vi "S2C_FPGA_SimulatedData.vi"(0 "sim I/O info in":T1, 9 "data from node input terminals":variant[](array[variant]), 11 "input from node terminal error in":errorcluster) -> (4 "sim I/O info out":T1, 10 "data to node output terminals":variant[](array[variant]), 15 "output to node terminal error out":errorcluster)   [LabVIEW 2015]
uses:
  <vilib>/FPGA/viExecutionOnDevComputer/simIO/customVI/Sim IO Info.ctl
  <vilib>/rvi/customViForEmulation/niLvFPGAUserSpecifiedEmulationVISupport.lvclass
  S2C_FPGA_InterfaceGlobals.vi
  <vilib>/FPGA/viExecutionOnDevComputer/simIO/customVI/niFPGA Simulated IO.lvlib
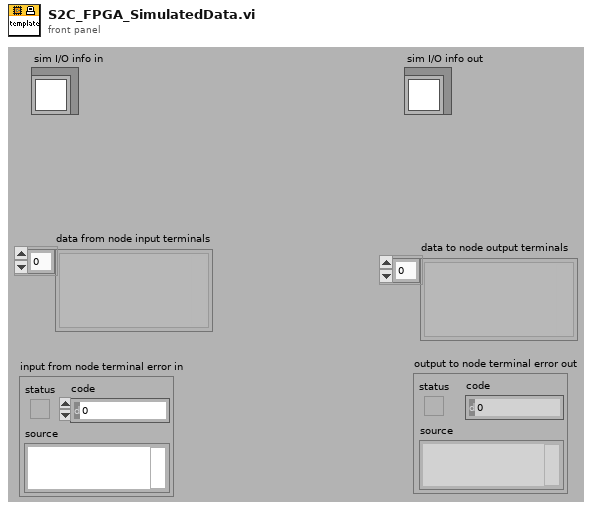
[diagram p1: front panel]
types:
  T1 = typedef "niFPGA Simulated IO.lvlib/Sim IO Info.ctl" = refnum<class "niLvFPGAUserSpecifiedEmulationVISupport.lvclass">
  T2 = typedef "niFPGA Simulated IO.lvlib/Execution Stage.ctl" = enum16{"Initializing", "Running", "Shutting Down"}
  T3 = typedef "niFPGA Simulated IO.lvlib/Node or Element Type.ctl" = enum16{"Read I/O", "Write I/O", "Method", "Read Property", "Write Property"}
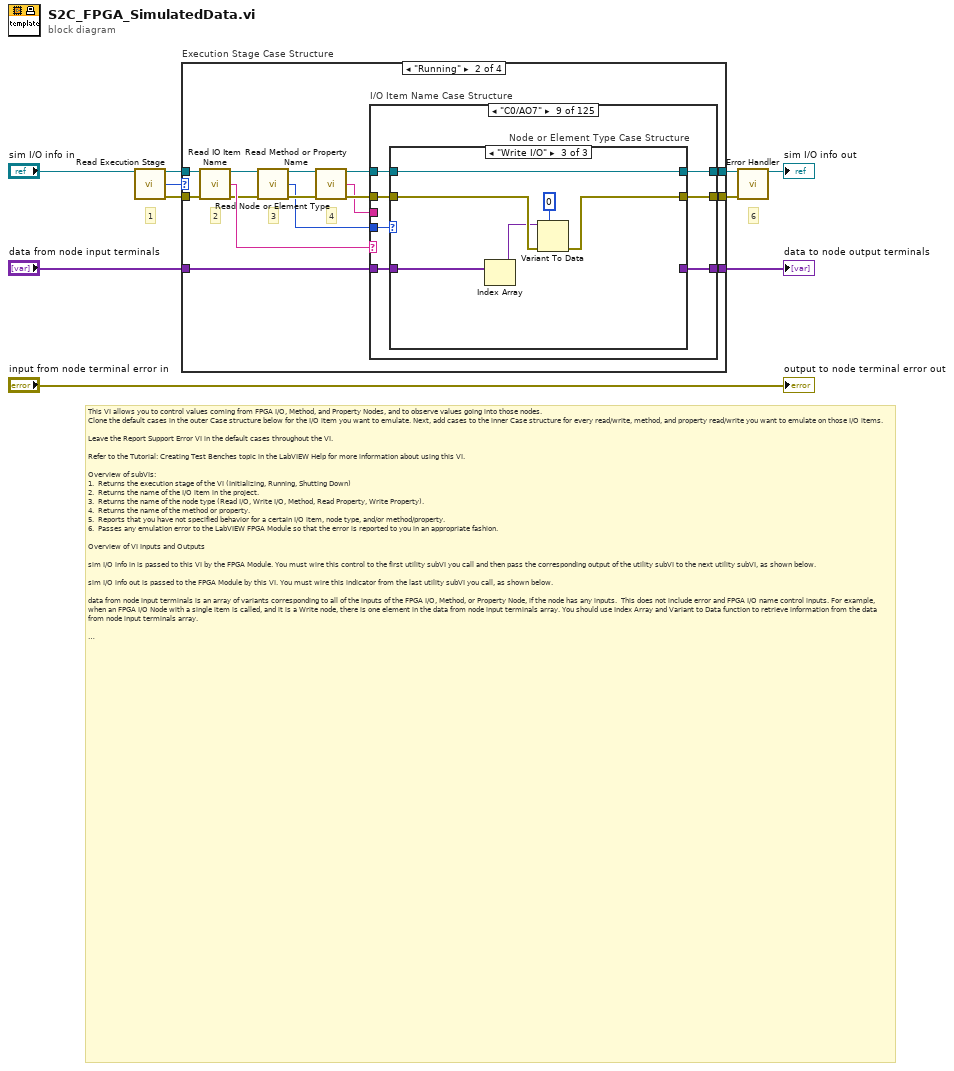
[diagram p0: block diagram]
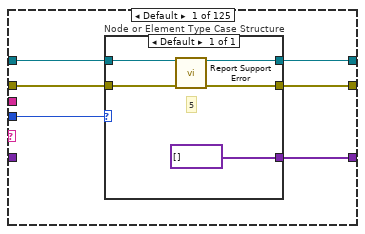
[diagram p3: hidden frame]
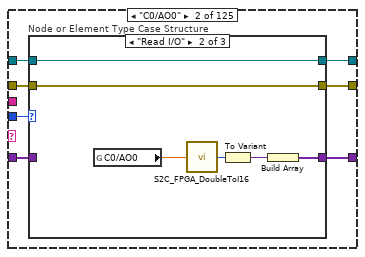
[diagram p4: hidden frame]
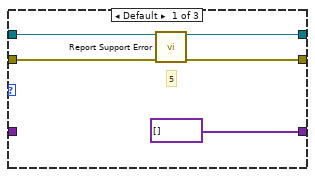
[diagram p5: hidden frame]
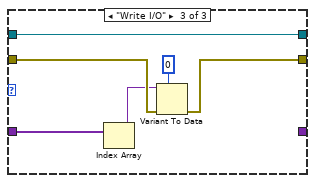
[diagram p6: hidden frame]
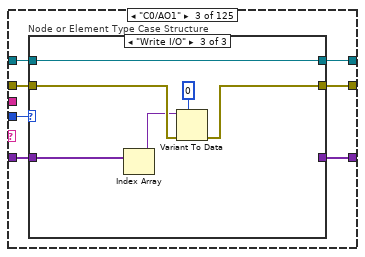
[diagram p7: hidden frame]
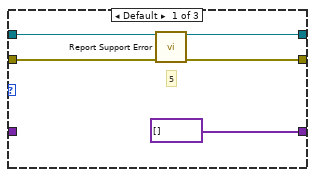
[diagram p8: hidden frame]
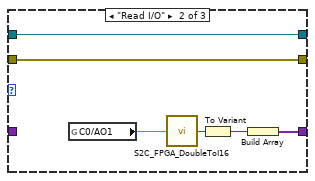
[diagram p9: hidden frame]
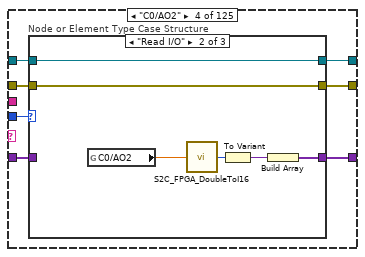
[diagram p10: hidden frame]
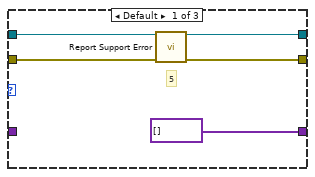
[diagram p11: hidden frame]
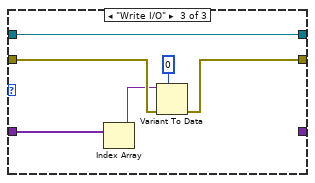
[diagram p12: hidden frame]
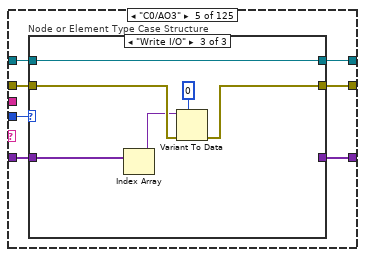
[diagram p13: hidden frame]
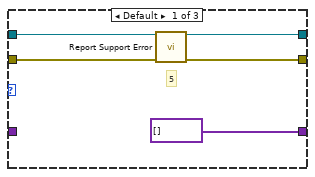
[diagram p14: hidden frame]
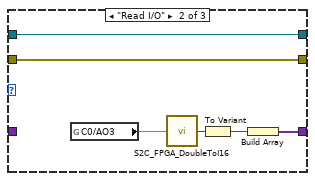
[diagram p15: hidden frame]
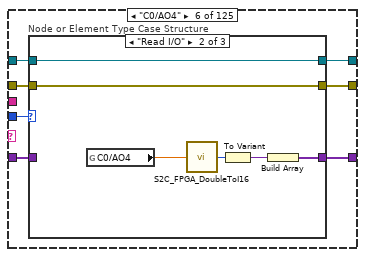
[diagram p16: hidden frame]
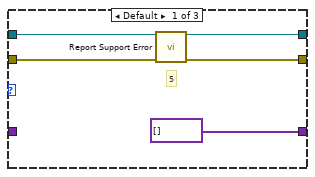
[diagram p17: hidden frame]
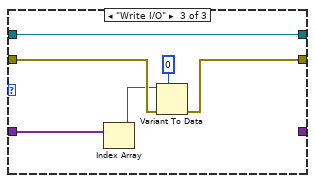
[diagram p18: hidden frame]
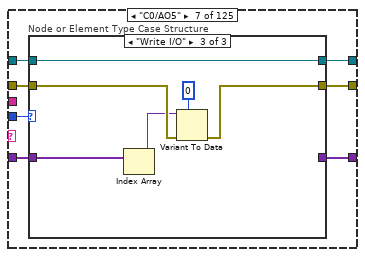
[diagram p19: hidden frame]
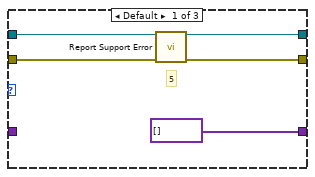
[diagram p20: hidden frame]
diagram:
  # "1"
  # "6"
  # "This VI allows you to control values coming from FPGA I/O, Method, and Property Nodes, and to observe values going into those nodes.\nClone the default cases in the outer Case structure below for the I/O item you want to emulate. Next, add cases to the inner Case structure for every read/write, method, and property read/write you want to emulate on those I/O items.  \n\nLeave the Report Support Error VI in the default cases throughout the VI.\n\nRefer to the Tutorial: Creating Test Benches topic in the LabVIEW Help for more information about using this VI.\n\nOverview of subVIs:\n1.  Returns the execution stage of the VI (Initializing, Running, Shutting Down)\n2.  Returns the name of the I/O item in the project.\n3.  Returns the name of the node type (Read I/O, Write I/O, Method, Read Property, Write Property).\n4.  Returns the name of the method or property.\n5.  Reports that you have not specified behavior for a certain I/O item, node type, and/or method/property.\n6.  Passes any emulation error to the LabVIEW FPGA Module so that the error is reported to you in an appropriate fashion.\n\nOverview of VI Inputs and Outputs\n\nsim I/O info in is passed to this VI by the FPGA Module. You must wire this control to the first utility subVI you call and then pass the corresponding output of the utility subVI to the next utility subVI, as shown below.\n\nsim I/O info out is passed to the FPGA Module by this VI. You must wire this indicator from the last utility subVI you call, as shown below.\n\ndata from node input terminals is an array of variants corresponding to all of the inputs of the FPGA I/O, Method, or Property Node, if the node has any inputs.  This does not include error and FPGA I/O name control inputs. For example, when an FPGA I/O Node with a single item is called, and it is a Write node, there is one element in the data from node input terminals array. You should use Index Array and Variant to Data function to retrieve information from the data from node input terminals array.\n\ndata to node output terminals is an array of variants corresponding to all the outputs of the FPGA I/O, Method, or Property Node, if the node has any outputs.  This does not include error and FPGA I/O name control outputs. For example, when an FPGA I/O node with a single item is called, and it is a Read node, there should be one element in the data to node output terminals array. You should use To Variant and Build Array functions to pass the information to the data to node output terminals array.\n\ninput from node terminal error in is the error that gets passed into the FPGA I/O, Method, or Property Node, if the node is configured so that the error input is shown. If the node is configured so that the error input is not shown, the value of this input corresponds to \"no error\" (status is false, error code is 0). \n\noutput to node terminal error out is the error that gets passed out of the FPGA I/O, Method, or Property Node, if the node is configured so that the error output is shown.  If the node is configured so that the error output is not shown, the value of this output is ignored."
  n1 = call <vilib>:"Read Execution Stage.vi"("sim I/O info in"="sim I/O info in") -> ("sim I/O info out"=w3:T1, "execution stage"=w1:T2, "error out"=w2:errorcluster)  [unwired: 1 in, 11 out]
  n2 = case "Execution Stage Case Structure" shown="\"Running\"" w1 {
    tunnel: [_ w26 _ _] -> w9
    tunnel: [w12 w21 w3124 w3126] -> w4
    tunnel: [w11 w17 w3123 w3125] -> w6
    tunnel: w3 -> [w11 w15 w3123 w3125]
    tunnel: w2 -> [w12 w14 w3124 w3126]
    tunnel: "data from node input terminals" -> [_ w27 _ _]
    frame "Initializing" {
    }
    frame "Running" {
      # "4"
      # "3"
      # "2"
      n3 = call <vilib>:"Read IO Item Name.vi"("sim I/O info in"=w15, "error in (no error)"=w14) -> ("sim I/O info out"=w16:T1, "I/O item name"=w25:string, "error out"=w24:errorcluster)  [unwired: 11 out]
      n4 = call <vilib>:"Read Node or Element Type.vi"("sim I/O info in"=w16, "error in (no error)"=w24) -> ("sim I/O info out"=w13:T1, "node or element type"=w22:T3, "error out"=w23:errorcluster)  [unwired: 11 out]
      n5 = call <vilib>:"Read Method or Property Name.vi"("sim I/O info in"=w13, "error in (no error)"=w23) -> ("sim I/O info out"=w19:T1, "method or property name"=w18:string, "error out"=w20:errorcluster)  [unwired: 11 out]
      n6 = case "I/O Item Name Case Structure" shown="\"C0/AO7\"" w25 {
        tunnel: w27 -> [_ w39 w63 w87 w111 w135 w159 w183 w207 w231 w255 w279 w303 w327 w351 w375 w399 w423 w456 w489 w522 w555 w588 w621 w654 w687 w720 w753 w786 w819 w843 w867 w891 w915 w939 w963 w987 w1011 w1035 w1059 w1083 w1107 w1131 w1155 w1179 w1203 w1227 w1251 w1275 w1299 w1323 w1347 w1371 w1395 w1419 w1443 w1467 w1491 w1515 w1539 w1563 w1587 w1611 w1635 w1659 w1683 w1707 w1731 w1755 w1779 w1803 w1827 w1851 w1875 w1899 w1923 w1947 w1971 w1995 w2019 w2043 w2067 w2091 w2115 w2139 w2163 w2187 w2211 w2235 w2259 w2283 w2307 w2331 w2355 w2379 w2403 w2427 w2451 w2475 w2499 w2523 w2547 w2571 w2595 w2619 w2643 w2667 w2691 w2715 w2739 w2763 w2787 w2811 w2835 w2859 w2883 w2907 w2931 w2955 w2979 w3003 w3027 w3051 w3075 w3099]
        tunnel: [w29 w41 w65 w89 w113 w137 w161 w185 w209 w233 w257 w281 w305 w329 w353 w377 w401 w425 w458 w491 w524 w557 w590 w623 w656 w689 w722 w755 w788 w821 w845 w869 w893 w917 w941 w965 w989 w1013 w1037 w1061 w1085 w1109 w1133 w1157 w1181 w1205 w1229 w1253 w1277 w1301 w1325 w1349 w1373 w1397 w1421 w1445 w1469 w1493 w1517 w1541 w1565 w1589 w1613 w1637 w1661 w1685 w1709 w1733 w1757 w1781 w1805 w1829 w1853 w1877 w1901 w1925 w1949 w1973 w1997 w2021 w2045 w2069 w2093 w2117 w2141 w2165 w2189 w2213 w2237 w2261 w2285 w2309 w2333 w2357 w2381 w2405 w2429 w2453 w2477 w2501 w2525 w2549 w2573 w2597 w2621 w2645 w2669 w2693 w2717 w2741 w2765 w2789 w2813 w2837 w2861 w2885 w2909 w2933 w2957 w2981 w3005 w3029 w3053 w3077 w3101] -> w26
        tunnel: w20 -> [w33 w45 w69 w93 w117 w141 w165 w189 w213 w237 w261 w285 w309 w333 w357 w381 w405 w429 w462 w495 w528 w561 w594 w627 w660 w693 w726 w759 w792 w825 w849 w873 w897 w921 w945 w969 w993 w1017 w1041 w1065 w1089 w1113 w1137 w1161 w1185 w1209 w1233 w1257 w1281 w1305 w1329 w1353 w1377 w1401 w1425 w1449 w1473 w1497 w1521 w1545 w1569 w1593 w1617 w1641 w1665 w1689 w1713 w1737 w1761 w1785 w1809 w1833 w1857 w1881 w1905 w1929 w1953 w1977 w2001 w2025 w2049 w2073 w2097 w2121 w2145 w2169 w2193 w2217 w2241 w2265 w2289 w2313 w2337 w2361 w2385 w2409 w2433 w2457 w2481 w2505 w2529 w2553 w2577 w2601 w2625 w2649 w2673 w2697 w2721 w2745 w2769 w2793 w2817 w2841 w2865 w2889 w2913 w2937 w2961 w2985 w3009 w3033 w3057 w3081 w3105]
        tunnel: [w32 w44 w68 w92 w116 w140 w164 w188 w212 w236 w260 w284 w308 w332 w356 w380 w404 w428 w461 w494 w527 w560 w593 w626 w659 w692 w725 w758 w791 w824 w848 w872 w896 w920 w944 w968 w992 w1016 w1040 w1064 w1088 w1112 w1136 w1160 w1184 w1208 w1232 w1256 w1280 w1304 w1328 w1352 w1376 w1400 w1424 w1448 w1472 w1496 w1520 w1544 w1568 w1592 w1616 w1640 w1664 w1688 w1712 w1736 w1760 w1784 w1808 w1832 w1856 w1880 w1904 w1928 w1952 w1976 w2000 w2024 w2048 w2072 w2096 w2120 w2144 w2168 w2192 w2216 w2240 w2264 w2288 w2312 w2336 w2360 w2384 w2408 w2432 w2456 w2480 w2504 w2528 w2552 w2576 w2600 w2624 w2648 w2672 w2696 w2720 w2744 w2768 w2792 w2816 w2840 w2864 w2888 w2912 w2936 w2960 w2984 w3008 w3032 w3056 w3080 w3104] -> w21
        tunnel: w19 -> [w31 w43 w67 w91 w115 w139 w163 w187 w211 w235 w259 w283 w307 w331 w355 w379 w403 w427 w460 w493 w526 w559 w592 w625 w658 w691 w724 w757 w790 w823 w847 w871 w895 w919 w943 w967 w991 w1015 w1039 w1063 w1087 w1111 w1135 w1159 w1183 w1207 w1231 w1255 w1279 w1303 w1327 w1351 w1375 w1399 w1423 w1447 w1471 w1495 w1519 w1543 w1567 w1591 w1615 w1639 w1663 w1687 w1711 w1735 w1759 w1783 w1807 w1831 w1855 w1879 w1903 w1927 w1951 w1975 w1999 w2023 w2047 w2071 w2095 w2119 w2143 w2167 w2191 w2215 w2239 w2263 w2287 w2311 w2335 w2359 w2383 w2407 w2431 w2455 w2479 w2503 w2527 w2551 w2575 w2599 w2623 w2647 w2671 w2695 w2719 w2743 w2767 w2791 w2815 w2839 w2863 w2887 w2911 w2935 w2959 w2983 w3007 w3031 w3055 w3079 w3103]
        tunnel: [w30 w42 w66 w90 w114 w138 w162 w186 w210 w234 w258 w282 w306 w330 w354 w378 w402 w426 w459 w492 w525 w558 w591 w624 w657 w690 w723 w756 w789 w822 w846 w870 w894 w918 w942 w966 w990 w1014 w1038 w1062 w1086 w1110 w1134 w1158 w1182 w1206 w1230 w1254 w1278 w1302 w1326 w1350 w1374 w1398 w1422 w1446 w1470 w1494 w1518 w1542 w1566 w1590 w1614 w1638 w1662 w1686 w1710 w1734 w1758 w1782 w1806 w1830 w1854 w1878 w1902 w1926 w1950 w1974 w1998 w2022 w2046 w2070 w2094 w2118 w2142 w2166 w2190 w2214 w2238 w2262 w2286 w2310 w2334 w2358 w2382 w2406 w2430 w2454 w2478 w2502 w2526 w2550 w2574 w2598 w2622 w2646 w2670 w2694 w2718 w2742 w2766 w2790 w2814 w2838 w2862 w2886 w2910 w2934 w2958 w2982 w3006 w3030 w3054 w3078 w3102] -> w17
        tunnel: w22 -> [w28 w40 w64 w88 w112 w136 w160 w184 w208 w232 w256 w280 w304 w328 w352 w376 w400 w424 w457 w490 w523 w556 w589 w622 w655 w688 w721 w754 w787 w820 w844 w868 w892 w916 w940 w964 w988 w1012 w1036 w1060 w1084 w1108 w1132 w1156 w1180 w1204 w1228 w1252 w1276 w1300 w1324 w1348 w1372 w1396 w1420 w1444 w1468 w1492 w1516 w1540 w1564 w1588 w1612 w1636 w1660 w1684 w1708 w1732 w1756 w1780 w1804 w1828 w1852 w1876 w1900 w1924 w1948 w1972 w1996 w2020 w2044 w2068 w2092 w2116 w2140 w2164 w2188 w2212 w2236 w2260 w2284 w2308 w2332 w2356 w2380 w2404 w2428 w2452 w2476 w2500 w2524 w2548 w2572 w2596 w2620 w2644 w2668 w2692 w2716 w2740 w2764 w2788 w2812 w2836 w2860 w2884 w2908 w2932 w2956 w2980 w3004 w3028 w3052 w3076 w3100]
        tunnel: w18 -> [_ _ _ _ _ _ _ _ _ _ _ _ _ _ _ _ _ _ _ _ _ _ _ _ _ _ _ _ _ _ _ _ _ _ _ _ _ _ _ _ _ _ _ _ _ _ _ _ _ _ _ _ _ _ _ _ _ _ _ _ _ _ _ _ _ _ _ _ _ _ _ _ _ _ _ _ _ _ _ _ _ _ _ _ _ _ _ _ _ _ _ _ _ _ _ _ _ _ _ _ _ _ _ _ _ _ _ _ _ _ _ _ _ _ _ _ _ _ _ _ _ _ _ _ _]
        frame Default {
          n7 = case "Node or Element Type Case Structure" shown="Default" w28 {
            tunnel: w33 -> [w38]
            tunnel: [w37] -> w32
            tunnel: w31 -> [w36]
            tunnel: [w35] -> w30
            tunnel: [variant[] []] -> w29
            frame Default {
              # "5"
              n8 = call <vilib>:"Report Support Error.vi"("sim I/O info in"=w36, "error in (no error)"=w38) -> ("sim I/O info out"=w35:T1, "error out"=w37:errorcluster)  [unwired: 12 out]
            }
          }
        }
        frame "C0/AO0" {
          n9 = case "Node or Element Type Case Structure" shown="\"Read I/O\"" w40 {
            tunnel: w45 -> [w50 w56 w60]
            tunnel: [w49 w56 w59] -> w44
            tunnel: w43 -> [w48 w55 w62]
            tunnel: [w47 w55 w62] -> w42
            tunnel: [variant[] [] w54 _] -> w41
            tunnel: w39 -> [_ _ w61]
            frame Default {
              # "5"
              n10 = call <vilib>:"Report Support Error.vi"("sim I/O info in"=w48, "error in (no error)"=w50) -> ("sim I/O info out"=w47:T1, "error out"=w49:errorcluster)  [unwired: 12 out]
            }
            frame "Read I/O" {
              n11 = global read "S2C_FPGA_InterfaceGlobals.vi" "C0/AO0"() -> (w52:dbl)
              n12 = call "S2C_FPGA_DoubleToI16.vi"("Double In"=w52) -> ("I16 Out"=w51:i16)  [unwired: 4 in]
              n13 = To Variant(anything=w51) -> (Variant=w53:variant)
              n14 = Build Array(w53) -> (w54:variant[])
            }
            frame "Write I/O" {
              n15 = Index Array(array=w61) -> (element=w58:variant)  [unwired: 1 in]
              n16 = Variant To Data(error in=w60, type=i16 0 ("C0/AI0"), Variant=w58) -> (error out=w59:errorcluster)  [unwired: 1 out]
            }
          }
        }
        frame "C0/AO1" {
          n17 = case "Node or Element Type Case Structure" shown="\"Write I/O\"" w64 {
            tunnel: w69 -> [w74 w80 w84]
            tunnel: [w73 w80 w83] -> w68
            tunnel: w67 -> [w72 w79 w86]
            tunnel: [w71 w79 w86] -> w66
            tunnel: [variant[] [] w77 _] -> w65
            tunnel: w63 -> [_ _ w85]
            frame Default {
              # "5"
              n18 = call <vilib>:"Report Support Error.vi"("sim I/O info in"=w72, "error in (no error)"=w74) -> ("sim I/O info out"=w71:T1, "error out"=w73:errorcluster)  [unwired: 12 out]
            }
            frame "Read I/O" {
              n19 = global read "S2C_FPGA_InterfaceGlobals.vi" "C0/AO1"() -> (w75:dbl)
              n20 = call "S2C_FPGA_DoubleToI16.vi"("Double In"=w75) -> ("I16 Out"=w76:i16)  [unwired: 4 in]
              n21 = To Variant(anything=w76) -> (Variant=w78:variant)
              n22 = Build Array(w78) -> (w77:variant[])
            }
            frame "Write I/O" {
              n23 = Index Array(array=w85) -> (element=w82:variant)  [unwired: 1 in]
              n24 = Variant To Data(error in=w84, type=i16 0 ("C0/AI0"), Variant=w82) -> (error out=w83:errorcluster)  [unwired: 1 out]
            }
          }
        }
        frame "C0/AO2" {
          n25 = case "Node or Element Type Case Structure" shown="\"Read I/O\"" w88 {
            tunnel: w93 -> [w98 w104 w108]
            tunnel: [w97 w104 w107] -> w92
            tunnel: w91 -> [w96 w103 w110]
            tunnel: [w95 w103 w110] -> w90
            tunnel: [variant[] [] w101 _] -> w89
            tunnel: w87 -> [_ _ w109]
            frame Default {
              # "5"
              n26 = call <vilib>:"Report Support Error.vi"("sim I/O info in"=w96, "error in (no error)"=w98) -> ("sim I/O info out"=w95:T1, "error out"=w97:errorcluster)  [unwired: 12 out]
            }
            frame "Read I/O" {
              n27 = global read "S2C_FPGA_InterfaceGlobals.vi" "C0/AO2"() -> (w99:dbl)
              n28 = call "S2C_FPGA_DoubleToI16.vi"("Double In"=w99) -> ("I16 Out"=w100:i16)  [unwired: 4 in]
              n29 = To Variant(anything=w100) -> (Variant=w102:variant)
              n30 = Build Array(w102) -> (w101:variant[])
            }
            frame "Write I/O" {
              n31 = Index Array(array=w109) -> (element=w106:variant)  [unwired: 1 in]
              n32 = Variant To Data(error in=w108, type=i16 0 ("C0/AI0"), Variant=w106) -> (error out=w107:errorcluster)  [unwired: 1 out]
            }
          }
        }
        frame "C0/AO3" {
          n33 = case "Node or Element Type Case Structure" shown="\"Write I/O\"" w112 {
            tunnel: w117 -> [w122 w128 w132]
            tunnel: [w121 w128 w131] -> w116
            tunnel: w115 -> [w120 w127 w134]
            tunnel: [w119 w127 w134] -> w114
            tunnel: [variant[] [] w125 _] -> w113
            tunnel: w111 -> [_ _ w133]
            frame Default {
              # "5"
              n34 = call <vilib>:"Report Support Error.vi"("sim I/O info in"=w120, "error in (no error)"=w122) -> ("sim I/O info out"=w119:T1, "error out"=w121:errorcluster)  [unwired: 12 out]
            }
            frame "Read I/O" {
              n35 = global read "S2C_FPGA_InterfaceGlobals.vi" "C0/AO3"() -> (w123:dbl)
              n36 = call "S2C_FPGA_DoubleToI16.vi"("Double In"=w123) -> ("I16 Out"=w124:i16)  [unwired: 4 in]
              n37 = To Variant(anything=w124) -> (Variant=w126:variant)
              n38 = Build Array(w126) -> (w125:variant[])
            }
            frame "Write I/O" {
              n39 = Index Array(array=w133) -> (element=w130:variant)  [unwired: 1 in]
              n40 = Variant To Data(error in=w132, type=i16 0 ("C0/AI0"), Variant=w130) -> (error out=w131:errorcluster)  [unwired: 1 out]
            }
          }
        }
        frame "C0/AO4" {
          n41 = case "Node or Element Type Case Structure" shown="\"Read I/O\"" w136 {
            tunnel: w141 -> [w146 w152 w156]
            tunnel: [w145 w152 w155] -> w140
            tunnel: w139 -> [w144 w151 w158]
            tunnel: [w143 w151 w158] -> w138
            tunnel: [variant[] [] w149 _] -> w137
            tunnel: w135 -> [_ _ w157]
            frame Default {
              # "5"
              n42 = call <vilib>:"Report Support Error.vi"("sim I/O info in"=w144, "error in (no error)"=w146) -> ("sim I/O info out"=w143:T1, "error out"=w145:errorcluster)  [unwired: 12 out]
            }
            frame "Read I/O" {
              n43 = global read "S2C_FPGA_InterfaceGlobals.vi" "C0/AO4"() -> (w147:dbl)
              n44 = call "S2C_FPGA_DoubleToI16.vi"("Double In"=w147) -> ("I16 Out"=w148:i16)  [unwired: 4 in]
              n45 = To Variant(anything=w148) -> (Variant=w150:variant)
              n46 = Build Array(w150) -> (w149:variant[])
            }
            frame "Write I/O" {
              n47 = Index Array(array=w157) -> (element=w154:variant)  [unwired: 1 in]
              n48 = Variant To Data(error in=w156, type=i16 0 ("C0/AI0"), Variant=w154) -> (error out=w155:errorcluster)  [unwired: 1 out]
            }
          }
        }
        frame "C0/AO5" {
          n49 = case "Node or Element Type Case Structure" shown="\"Write I/O\"" w160 {
            tunnel: w165 -> [w170 w176 w180]
            tunnel: [w169 w176 w179] -> w164
            tunnel: w163 -> [w168 w175 w182]
            tunnel: [w167 w175 w182] -> w162
            tunnel: [variant[] [] w173 _] -> w161
            tunnel: w159 -> [_ _ w181]
            frame Default {
              # "5"
              n50 = call <vilib>:"Report Support Error.vi"("sim I/O info in"=w168, "error in (no error)"=w170) -> ("sim I/O info out"=w167:T1, "error out"=w169:errorcluster)  [unwired: 12 out]
            }
            frame "Read I/O" {
              n51 = global read "S2C_FPGA_InterfaceGlobals.vi" "C0/AO5"() -> (w171:dbl)
              n52 = call "S2C_FPGA_DoubleToI16.vi"("Double In"=w171) -> ("I16 Out"=w172:i16)  [unwired: 4 in]
              n53 = To Variant(anything=w172) -> (Variant=w174:variant)
              n54 = Build Array(w174) -> (w173:variant[])
            }
            frame "Write I/O" {
              n55 = Index Array(array=w181) -> (element=w178:variant)  [unwired: 1 in]
              n56 = Variant To Data(error in=w180, type=i16 0 ("C0/AI0"), Variant=w178) -> (error out=w179:errorcluster)  [unwired: 1 out]
            }
          }
        }
        frame "C0/AO6" {
          n57 = case "Node or Element Type Case Structure" shown="\"Read I/O\"" w184 {
            tunnel: w189 -> [w194 w200 w204]
            tunnel: [w193 w200 w203] -> w188
            tunnel: w187 -> [w192 w199 w206]
            tunnel: [w191 w199 w206] -> w186
            tunnel: [variant[] [] w197 _] -> w185
            tunnel: w183 -> [_ _ w205]
            frame Default {
              # "5"
              n58 = call <vilib>:"Report Support Error.vi"("sim I/O info in"=w192, "error in (no error)"=w194) -> ("sim I/O info out"=w191:T1, "error out"=w193:errorcluster)  [unwired: 12 out]
            }
            frame "Read I/O" {
              n59 = global read "S2C_FPGA_InterfaceGlobals.vi" "C0/AO6"() -> (w195:dbl)
              n60 = call "S2C_FPGA_DoubleToI16.vi"("Double In"=w195) -> ("I16 Out"=w196:i16)  [unwired: 4 in]
              n61 = To Variant(anything=w196) -> (Variant=w198:variant)
              n62 = Build Array(w198) -> (w197:variant[])
            }
            frame "Write I/O" {
              n63 = Index Array(array=w205) -> (element=w202:variant)  [unwired: 1 in]
              n64 = Variant To Data(error in=w204, type=i16 0 ("C0/AI0"), Variant=w202) -> (error out=w203:errorcluster)  [unwired: 1 out]
            }
          }
        }
        frame "C0/AO7" {
          n65 = case "Node or Element Type Case Structure" shown="\"Write I/O\"" w208 {
            tunnel: w213 -> [w218 w224 w228]
            tunnel: [w217 w224 w227] -> w212
            tunnel: w211 -> [w216 w223 w230]
            tunnel: [w215 w223 w230] -> w210
            tunnel: [variant[] [] w221 _] -> w209
            tunnel: w207 -> [_ _ w229]
            frame Default {
              # "5"
              n66 = call <vilib>:"Report Support Error.vi"("sim I/O info in"=w216, "error in (no error)"=w218) -> ("sim I/O info out"=w215:T1, "error out"=w217:errorcluster)  [unwired: 12 out]
            }
            frame "Read I/O" {
              n67 = global read "S2C_FPGA_InterfaceGlobals.vi" "C0/AO7"() -> (w219:dbl)
              n68 = call "S2C_FPGA_DoubleToI16.vi"("Double In"=w219) -> ("I16 Out"=w220:i16)  [unwired: 4 in]
              n69 = To Variant(anything=w220) -> (Variant=w222:variant)
              n70 = Build Array(w222) -> (w221:variant[])
            }
            frame "Write I/O" {
              n71 = Index Array(array=w229) -> (element=w226:variant)  [unwired: 1 in]
              n72 = Variant To Data(error in=w228, type=i16 0 ("C0/AI0"), Variant=w226) -> (error out=w227:errorcluster)  [unwired: 1 out]
            }
          }
        }
        frame "C0/AI0" {
          n73 = case "Node or Element Type Case Structure" shown="\"Read I/O\"" w232 {
            tunnel: w237 -> [w242 w248 w252]
            tunnel: [w241 w248 w251] -> w236
            tunnel: w235 -> [w240 w247 w254]
            tunnel: [w239 w247 w254] -> w234
            tunnel: [variant[] [] w245 _] -> w233
            tunnel: w231 -> [_ _ w253]
            frame Default {
              # "5"
              n74 = call <vilib>:"Report Support Error.vi"("sim I/O info in"=w240, "error in (no error)"=w242) -> ("sim I/O info out"=w239:T1, "error out"=w241:errorcluster)  [unwired: 12 out]
            }
            frame "Read I/O" {
              n75 = global read "S2C_FPGA_InterfaceGlobals.vi" "C0/AI0"() -> (w244:dbl)
              n76 = call "S2C_FPGA_DoubleToI16.vi"("Double In"=w244) -> ("I16 Out"=w243:i16)  [unwired: 4 in]
              n77 = To Variant(anything=w243) -> (Variant=w246:variant)
              n78 = Build Array(w246) -> (w245:variant[])
            }
            frame "Write I/O" {
              n79 = Index Array(array=w253) -> (element=w250:variant)  [unwired: 1 in]
              n80 = Variant To Data(error in=w252, type=0.0 ("C0/AI0"), Variant=w250) -> (error out=w251:errorcluster)  [unwired: 1 out]
            }
          }
        }
        frame "C0/AI1" {
          n81 = case "Node or Element Type Case Structure" shown="\"Read I/O\"" w256 {
            tunnel: w261 -> [w266 w272 w276]
            tunnel: [w265 w272 w275] -> w260
            tunnel: w259 -> [w264 w271 w278]
            tunnel: [w263 w271 w278] -> w258
            tunnel: [variant[] [] w269 _] -> w257
            tunnel: w255 -> [_ _ w277]
            frame Default {
              # "5"
              n82 = call <vilib>:"Report Support Error.vi"("sim I/O info in"=w264, "error in (no error)"=w266) -> ("sim I/O info out"=w263:T1, "error out"=w265:errorcluster)  [unwired: 12 out]
            }
            frame "Read I/O" {
              n83 = global read "S2C_FPGA_InterfaceGlobals.vi" "C0/AI1"() -> (w267:dbl)
              n84 = call "S2C_FPGA_DoubleToI16.vi"("Double In"=w267) -> ("I16 Out"=w268:i16)  [unwired: 4 in]
              n85 = To Variant(anything=w268) -> (Variant=w270:variant)
              n86 = Build Array(w270) -> (w269:variant[])
            }
            frame "Write I/O" {
              n87 = Index Array(array=w277) -> (element=w274:variant)  [unwired: 1 in]
              n88 = Variant To Data(error in=w276, type=0.0 ("C0/AI0"), Variant=w274) -> (error out=w275:errorcluster)  [unwired: 1 out]
            }
          }
        }
        frame "C0/AI2" {
          n89 = case "Node or Element Type Case Structure" shown="\"Read I/O\"" w280 {
            tunnel: w285 -> [w290 w296 w300]
            tunnel: [w289 w296 w299] -> w284
            tunnel: w283 -> [w288 w295 w302]
            tunnel: [w287 w295 w302] -> w282
            tunnel: [variant[] [] w293 _] -> w281
            tunnel: w279 -> [_ _ w301]
            frame Default {
              # "5"
              n90 = call <vilib>:"Report Support Error.vi"("sim I/O info in"=w288, "error in (no error)"=w290) -> ("sim I/O info out"=w287:T1, "error out"=w289:errorcluster)  [unwired: 12 out]
            }
            frame "Read I/O" {
              n91 = global read "S2C_FPGA_InterfaceGlobals.vi" "C0/AI2"() -> (w291:dbl)
              n92 = call "S2C_FPGA_DoubleToI16.vi"("Double In"=w291) -> ("I16 Out"=w292:i16)  [unwired: 4 in]
              n93 = To Variant(anything=w292) -> (Variant=w294:variant)
              n94 = Build Array(w294) -> (w293:variant[])
            }
            frame "Write I/O" {
              n95 = Index Array(array=w301) -> (element=w298:variant)  [unwired: 1 in]
              n96 = Variant To Data(error in=w300, type=0.0 ("C0/AI0"), Variant=w298) -> (error out=w299:errorcluster)  [unwired: 1 out]
            }
          }
        }
        frame "C0/AI3" {
          n97 = case "Node or Element Type Case Structure" shown="\"Read I/O\"" w304 {
            tunnel: w309 -> [w314 w320 w324]
            tunnel: [w313 w320 w323] -> w308
            tunnel: w307 -> [w312 w319 w326]
            tunnel: [w311 w319 w326] -> w306
            tunnel: [variant[] [] w317 _] -> w305
            tunnel: w303 -> [_ _ w325]
            frame Default {
              # "5"
              n98 = call <vilib>:"Report Support Error.vi"("sim I/O info in"=w312, "error in (no error)"=w314) -> ("sim I/O info out"=w311:T1, "error out"=w313:errorcluster)  [unwired: 12 out]
            }
            frame "Read I/O" {
              n99 = global read "S2C_FPGA_InterfaceGlobals.vi" "C0/AI3"() -> (w315:dbl)
              n100 = call "S2C_FPGA_DoubleToI16.vi"("Double In"=w315) -> ("I16 Out"=w316:i16)  [unwired: 4 in]
              n101 = To Variant(anything=w316) -> (Variant=w318:variant)
              n102 = Build Array(w318) -> (w317:variant[])
            }
            frame "Write I/O" {
              n103 = Index Array(array=w325) -> (element=w322:variant)  [unwired: 1 in]
              n104 = Variant To Data(error in=w324, type=0.0 ("C0/AI0"), Variant=w322) -> (error out=w323:errorcluster)  [unwired: 1 out]
            }
          }
        }
        frame "C0/AI4" {
          n105 = case "Node or Element Type Case Structure" shown="\"Read I/O\"" w328 {
            tunnel: w333 -> [w338 w344 w348]
            tunnel: [w337 w344 w347] -> w332
            tunnel: w331 -> [w336 w343 w350]
            tunnel: [w335 w343 w350] -> w330
            tunnel: [variant[] [] w341 _] -> w329
            tunnel: w327 -> [_ _ w349]
            frame Default {
              # "5"
              n106 = call <vilib>:"Report Support Error.vi"("sim I/O info in"=w336, "error in (no error)"=w338) -> ("sim I/O info out"=w335:T1, "error out"=w337:errorcluster)  [unwired: 12 out]
            }
            frame "Read I/O" {
              n107 = global read "S2C_FPGA_InterfaceGlobals.vi" "C0/AI4"() -> (w339:dbl)
              n108 = call "S2C_FPGA_DoubleToI16.vi"("Double In"=w339) -> ("I16 Out"=w340:i16)  [unwired: 4 in]
              n109 = To Variant(anything=w340) -> (Variant=w342:variant)
              n110 = Build Array(w342) -> (w341:variant[])
            }
            frame "Write I/O" {
              n111 = Index Array(array=w349) -> (element=w346:variant)  [unwired: 1 in]
              n112 = Variant To Data(error in=w348, type=0.0 ("C0/AI0"), Variant=w346) -> (error out=w347:errorcluster)  [unwired: 1 out]
            }
          }
        }
        frame "C0/AI5" {
          n113 = case "Node or Element Type Case Structure" shown="\"Read I/O\"" w352 {
            tunnel: w357 -> [w362 w368 w372]
            tunnel: [w361 w368 w371] -> w356
            tunnel: w355 -> [w360 w367 w374]
            tunnel: [w359 w367 w374] -> w354
            tunnel: [variant[] [] w365 _] -> w353
            tunnel: w351 -> [_ _ w373]
            frame Default {
              # "5"
              n114 = call <vilib>:"Report Support Error.vi"("sim I/O info in"=w360, "error in (no error)"=w362) -> ("sim I/O info out"=w359:T1, "error out"=w361:errorcluster)  [unwired: 12 out]
            }
            frame "Read I/O" {
              n115 = global read "S2C_FPGA_InterfaceGlobals.vi" "C0/AI5"() -> (w363:dbl)
              n116 = call "S2C_FPGA_DoubleToI16.vi"("Double In"=w363) -> ("I16 Out"=w364:i16)  [unwired: 4 in]
              n117 = To Variant(anything=w364) -> (Variant=w366:variant)
              n118 = Build Array(w366) -> (w365:variant[])
            }
            frame "Write I/O" {
              n119 = Index Array(array=w373) -> (element=w370:variant)  [unwired: 1 in]
              n120 = Variant To Data(error in=w372, type=0.0 ("C0/AI0"), Variant=w370) -> (error out=w371:errorcluster)  [unwired: 1 out]
            }
          }
        }
        frame "C0/AI6" {
          n121 = case "Node or Element Type Case Structure" shown="\"Read I/O\"" w376 {
            tunnel: w381 -> [w386 w392 w396]
            tunnel: [w385 w392 w395] -> w380
            tunnel: w379 -> [w384 w391 w398]
            tunnel: [w383 w391 w398] -> w378
            tunnel: [variant[] [] w389 _] -> w377
            tunnel: w375 -> [_ _ w397]
            frame Default {
              # "5"
              n122 = call <vilib>:"Report Support Error.vi"("sim I/O info in"=w384, "error in (no error)"=w386) -> ("sim I/O info out"=w383:T1, "error out"=w385:errorcluster)  [unwired: 12 out]
            }
            frame "Read I/O" {
              n123 = global read "S2C_FPGA_InterfaceGlobals.vi" "C0/AI6"() -> (w387:dbl)
              n124 = call "S2C_FPGA_DoubleToI16.vi"("Double In"=w387) -> ("I16 Out"=w388:i16)  [unwired: 4 in]
              n125 = To Variant(anything=w388) -> (Variant=w390:variant)
              n126 = Build Array(w390) -> (w389:variant[])
            }
            frame "Write I/O" {
              n127 = Index Array(array=w397) -> (element=w394:variant)  [unwired: 1 in]
              n128 = Variant To Data(error in=w396, type=0.0 ("C0/AI0"), Variant=w394) -> (error out=w395:errorcluster)  [unwired: 1 out]
            }
          }
        }
        frame "C0/AI7" {
          n129 = case "Node or Element Type Case Structure" shown="\"Read I/O\"" w400 {
            tunnel: w405 -> [w410 w416 w420]
            tunnel: [w409 w416 w419] -> w404
            tunnel: w403 -> [w408 w415 w422]
            tunnel: [w407 w415 w422] -> w402
            tunnel: [variant[] [] w413 _] -> w401
            tunnel: w399 -> [_ _ w421]
            frame Default {
              # "5"
              n130 = call <vilib>:"Report Support Error.vi"("sim I/O info in"=w408, "error in (no error)"=w410) -> ("sim I/O info out"=w407:T1, "error out"=w409:errorcluster)  [unwired: 12 out]
            }
            frame "Read I/O" {
              n131 = global read "S2C_FPGA_InterfaceGlobals.vi" "C0/AI7"() -> (w411:dbl)
              n132 = call "S2C_FPGA_DoubleToI16.vi"("Double In"=w411) -> ("I16 Out"=w412:i16)  [unwired: 4 in]
              n133 = To Variant(anything=w412) -> (Variant=w414:variant)
              n134 = Build Array(w414) -> (w413:variant[])
            }
            frame "Write I/O" {
              n135 = Index Array(array=w421) -> (element=w418:variant)  [unwired: 1 in]
              n136 = Variant To Data(error in=w420, type=0.0 ("C0/AI0"), Variant=w418) -> (error out=w419:errorcluster)  [unwired: 1 out]
            }
          }
        }
        frame "C0/P0" {
          n137 = case "Node or Element Type Case Structure" shown="\"Read I/O\"" w424 {
            tunnel: w429 -> [w434 w448 w453]
            tunnel: [w433 w448 w452] -> w428
            tunnel: w427 -> [w432 w447 w455]
            tunnel: [w431 w447 w455] -> w426
            tunnel: [variant[] [] w445 _] -> w425
            tunnel: w423 -> [_ _ w454]
            frame Default {
              # "5"
              n138 = call <vilib>:"Report Support Error.vi"("sim I/O info in"=w432, "error in (no error)"=w434) -> ("sim I/O info out"=w431:T1, "error out"=w433:errorcluster)  [unwired: 12 out]
            }
            frame "Read I/O" {
              n139 = global read "S2C_FPGA_InterfaceGlobals.vi" "C0/P0/B0"() -> (w444:bool)
              n140 = global read "S2C_FPGA_InterfaceGlobals.vi" "C0/P0/B1"() -> (w441:bool)
              n141 = global read "S2C_FPGA_InterfaceGlobals.vi" "C0/P0/B2"() -> (w439:bool)
              n142 = global read "S2C_FPGA_InterfaceGlobals.vi" "C0/P0/B3"() -> (w438:bool)
              n143 = global read "S2C_FPGA_InterfaceGlobals.vi" "C0/P0/B4"() -> (w437:bool)
              n144 = global read "S2C_FPGA_InterfaceGlobals.vi" "C0/P0/B5"() -> (w440:bool)
              n145 = global read "S2C_FPGA_InterfaceGlobals.vi" "C0/P0/B6"() -> (w442:bool)
              n146 = global read "S2C_FPGA_InterfaceGlobals.vi" "C0/P0/B7"() -> (w443:bool)
              n147 = Build Array(w444, w441, w439, w438, w437, w440, w442, w443) -> (w436:bool[])
              n148 = Boolean Array To Number(Boolean array=w436) -> (number=w435:u32)
              n149 = To Variant(anything=w435) -> (Variant=w446:variant)
              n150 = Build Array(w446) -> (w445:variant[])
            }
            frame "Write I/O" {
              n151 = Index Array(array=w454) -> (element=w450:variant)  [unwired: 1 in]
              n152 = Variant To Data(error in=w453, type=u8 0, Variant=w450) -> (data=w449:u8, error out=w452:errorcluster)
              n153 = global write "S2C_FPGA_InterfaceGlobals.vi" "C0_P0 Out"(w449) -> ()
            }
          }
        }
        frame "C0/P1" {
          n154 = case "Node or Element Type Case Structure" shown="\"Read I/O\"" w457 {
            tunnel: w462 -> [w467 w481 w486]
            tunnel: [w466 w481 w485] -> w461
            tunnel: w460 -> [w465 w480 w488]
            tunnel: [w464 w480 w488] -> w459
            tunnel: [variant[] [] w478 _] -> w458
            tunnel: w456 -> [_ _ w487]
            frame Default {
              # "5"
              n155 = call <vilib>:"Report Support Error.vi"("sim I/O info in"=w465, "error in (no error)"=w467) -> ("sim I/O info out"=w464:T1, "error out"=w466:errorcluster)  [unwired: 12 out]
            }
            frame "Read I/O" {
              n156 = global read "S2C_FPGA_InterfaceGlobals.vi" "C0/P1/B0"() -> (w477:bool)
              n157 = global read "S2C_FPGA_InterfaceGlobals.vi" "C0/P1/B1"() -> (w474:bool)
              n158 = global read "S2C_FPGA_InterfaceGlobals.vi" "C0/P1/B2"() -> (w472:bool)
              n159 = global read "S2C_FPGA_InterfaceGlobals.vi" "C0/P1/B3"() -> (w471:bool)
              n160 = global read "S2C_FPGA_InterfaceGlobals.vi" "C0/P1/B4"() -> (w470:bool)
              n161 = global read "S2C_FPGA_InterfaceGlobals.vi" "C0/P1/B5"() -> (w473:bool)
              n162 = global read "S2C_FPGA_InterfaceGlobals.vi" "C0/P1/B6"() -> (w475:bool)
              n163 = global read "S2C_FPGA_InterfaceGlobals.vi" "C0/P1/B7"() -> (w476:bool)
              n164 = Build Array(w477, w474, w472, w471, w470, w473, w475, w476) -> (w469:bool[])
              n165 = Boolean Array To Number(Boolean array=w469) -> (number=w468:u32)
              n166 = To Variant(anything=w468) -> (Variant=w479:variant)
              n167 = Build Array(w479) -> (w478:variant[])
            }
            frame "Write I/O" {
              n168 = Index Array(array=w487) -> (element=w483:variant)  [unwired: 1 in]
              n169 = Variant To Data(error in=w486, type=u8 0, Variant=w483) -> (data=w482:u8, error out=w485:errorcluster)
              n170 = global write "S2C_FPGA_InterfaceGlobals.vi" "C0_P1 Out"(w482) -> ()
            }
          }
        }
        frame "C1/P0" {
          n171 = case "Node or Element Type Case Structure" shown="\"Read I/O\"" w490 {
            tunnel: w495 -> [w500 w514 w519]
            tunnel: [w499 w514 w518] -> w494
            tunnel: w493 -> [w498 w513 w521]
            tunnel: [w497 w513 w521] -> w492
            tunnel: [variant[] [] w511 _] -> w491
            tunnel: w489 -> [_ _ w520]
            frame Default {
              # "5"
              n172 = call <vilib>:"Report Support Error.vi"("sim I/O info in"=w498, "error in (no error)"=w500) -> ("sim I/O info out"=w497:T1, "error out"=w499:errorcluster)  [unwired: 12 out]
            }
            frame "Read I/O" {
              n173 = global read "S2C_FPGA_InterfaceGlobals.vi" "C1/P0/B0"() -> (w510:bool)
              n174 = global read "S2C_FPGA_InterfaceGlobals.vi" "C1/P0/B1"() -> (w507:bool)
              n175 = global read "S2C_FPGA_InterfaceGlobals.vi" "C1/P0/B2"() -> (w505:bool)
              n176 = global read "S2C_FPGA_InterfaceGlobals.vi" "C1/P0/B3"() -> (w504:bool)
              n177 = global read "S2C_FPGA_InterfaceGlobals.vi" "C1/P0/B4"() -> (w503:bool)
              n178 = global read "S2C_FPGA_InterfaceGlobals.vi" "C1/P0/B5"() -> (w506:bool)
              n179 = global read "S2C_FPGA_InterfaceGlobals.vi" "C1/P0/B6"() -> (w508:bool)
              n180 = global read "S2C_FPGA_InterfaceGlobals.vi" "C1/P0/B7"() -> (w509:bool)
              n181 = Build Array(w510, w507, w505, w504, w503, w506, w508, w509) -> (w501:bool[])
              n182 = Boolean Array To Number(Boolean array=w501) -> (number=w502:u32)
              n183 = To Variant(anything=w502) -> (Variant=w512:variant)
              n184 = Build Array(w512) -> (w511:variant[])
            }
            frame "Write I/O" {
              n185 = Index Array(array=w520) -> (element=w516:variant)  [unwired: 1 in]
              n186 = Variant To Data(error in=w519, type=u8 0, Variant=w516) -> (data=w515:u8, error out=w518:errorcluster)
              n187 = global write "S2C_FPGA_InterfaceGlobals.vi" "C1_P0 Out"(w515) -> ()
            }
          }
        }
        frame "C1/P1" {
          n188 = case "Node or Element Type Case Structure" shown="\"Read I/O\"" w523 {
            tunnel: w528 -> [w533 w547 w552]
            tunnel: [w532 w547 w551] -> w527
            tunnel: w526 -> [w531 w546 w554]
            tunnel: [w530 w546 w554] -> w525
            tunnel: [variant[] [] w544 _] -> w524
            tunnel: w522 -> [_ _ w553]
            frame Default {
              # "5"
              n189 = call <vilib>:"Report Support Error.vi"("sim I/O info in"=w531, "error in (no error)"=w533) -> ("sim I/O info out"=w530:T1, "error out"=w532:errorcluster)  [unwired: 12 out]
            }
            frame "Read I/O" {
              n190 = global read "S2C_FPGA_InterfaceGlobals.vi" "C1/P1/B0"() -> (w542:bool)
              n191 = global read "S2C_FPGA_InterfaceGlobals.vi" "C1/P1/B1"() -> (w539:bool)
              n192 = global read "S2C_FPGA_InterfaceGlobals.vi" "C1/P1/B2"() -> (w537:bool)
              n193 = global read "S2C_FPGA_InterfaceGlobals.vi" "C1/P1/B3"() -> (w536:bool)
              n194 = global read "S2C_FPGA_InterfaceGlobals.vi" "C1/P1/B4"() -> (w535:bool)
              n195 = global read "S2C_FPGA_InterfaceGlobals.vi" "C1/P1/B5"() -> (w538:bool)
              n196 = global read "S2C_FPGA_InterfaceGlobals.vi" "C1/P1/B6"() -> (w540:bool)
              n197 = global read "S2C_FPGA_InterfaceGlobals.vi" "C1/P1/B7"() -> (w541:bool)
              n198 = Build Array(w542, w539, w537, w536, w535, w538, w540, w541) -> (w543:bool[])
              n199 = Boolean Array To Number(Boolean array=w543) -> (number=w534:u32)
              n200 = To Variant(anything=w534) -> (Variant=w545:variant)
              n201 = Build Array(w545) -> (w544:variant[])
            }
            frame "Write I/O" {
              n202 = Index Array(array=w553) -> (element=w549:variant)  [unwired: 1 in]
              n203 = Variant To Data(error in=w552, type=u8 0, Variant=w549) -> (data=w548:u8, error out=w551:errorcluster)
              n204 = global write "S2C_FPGA_InterfaceGlobals.vi" "C1_P1 Out"(w548) -> ()
            }
          }
        }
        frame "C1/P2" {
          n205 = case "Node or Element Type Case Structure" shown="\"Read I/O\"" w556 {
            tunnel: w561 -> [w566 w580 w585]
            tunnel: [w565 w580 w584] -> w560
            tunnel: w559 -> [w564 w579 w587]
            tunnel: [w563 w579 w587] -> w558
            tunnel: [variant[] [] w577 _] -> w557
            tunnel: w555 -> [_ _ w586]
            frame Default {
              # "5"
              n206 = call <vilib>:"Report Support Error.vi"("sim I/O info in"=w564, "error in (no error)"=w566) -> ("sim I/O info out"=w563:T1, "error out"=w565:errorcluster)  [unwired: 12 out]
            }
            frame "Read I/O" {
              n207 = global read "S2C_FPGA_InterfaceGlobals.vi" "C1/P2/B0"() -> (w575:bool)
              n208 = global read "S2C_FPGA_InterfaceGlobals.vi" "C1/P2/B1"() -> (w572:bool)
              n209 = global read "S2C_FPGA_InterfaceGlobals.vi" "C1/P2/B2"() -> (w570:bool)
              n210 = global read "S2C_FPGA_InterfaceGlobals.vi" "C1/P2/B3"() -> (w569:bool)
              n211 = global read "S2C_FPGA_InterfaceGlobals.vi" "C1/P2/B4"() -> (w568:bool)
              n212 = global read "S2C_FPGA_InterfaceGlobals.vi" "C1/P2/B5"() -> (w571:bool)
              n213 = global read "S2C_FPGA_InterfaceGlobals.vi" "C1/P2/B6"() -> (w573:bool)
              n214 = global read "S2C_FPGA_InterfaceGlobals.vi" "C1/P2/B7"() -> (w574:bool)
              n215 = Build Array(w575, w572, w570, w569, w568, w571, w573, w574) -> (w576:bool[])
              n216 = Boolean Array To Number(Boolean array=w576) -> (number=w567:u32)
              n217 = To Variant(anything=w567) -> (Variant=w578:variant)
              n218 = Build Array(w578) -> (w577:variant[])
            }
            frame "Write I/O" {
              n219 = Index Array(array=w586) -> (element=w582:variant)  [unwired: 1 in]
              n220 = Variant To Data(error in=w585, type=u8 0, Variant=w582) -> (data=w581:u8, error out=w584:errorcluster)
              n221 = global write "S2C_FPGA_InterfaceGlobals.vi" "C1_P2 Out"(w581) -> ()
            }
          }
        }
        frame "C1/P3" {
          n222 = case "Node or Element Type Case Structure" shown="\"Read I/O\"" w589 {
            tunnel: w594 -> [w599 w613 w618]
            tunnel: [w598 w613 w617] -> w593
            tunnel: w592 -> [w597 w612 w620]
            tunnel: [w596 w612 w620] -> w591
            tunnel: [variant[] [] w610 _] -> w590
            tunnel: w588 -> [_ _ w619]
            frame Default {
              # "5"
              n223 = call <vilib>:"Report Support Error.vi"("sim I/O info in"=w597, "error in (no error)"=w599) -> ("sim I/O info out"=w596:T1, "error out"=w598:errorcluster)  [unwired: 12 out]
            }
            frame "Read I/O" {
              n224 = global read "S2C_FPGA_InterfaceGlobals.vi" "C1/P3/B0"() -> (w608:bool)
              n225 = global read "S2C_FPGA_InterfaceGlobals.vi" "C1/P3/B1"() -> (w605:bool)
              n226 = global read "S2C_FPGA_InterfaceGlobals.vi" "C1/P3/B2"() -> (w603:bool)
              n227 = global read "S2C_FPGA_InterfaceGlobals.vi" "C1/P3/B3"() -> (w602:bool)
              n228 = global read "S2C_FPGA_InterfaceGlobals.vi" "C1/P3/B4"() -> (w601:bool)
              n229 = global read "S2C_FPGA_InterfaceGlobals.vi" "C1/P3/B5"() -> (w604:bool)
              n230 = global read "S2C_FPGA_InterfaceGlobals.vi" "C1/P3/B6"() -> (w606:bool)
              n231 = global read "S2C_FPGA_InterfaceGlobals.vi" "C1/P3/B7"() -> (w607:bool)
              n232 = Build Array(w608, w605, w603, w602, w601, w604, w606, w607) -> (w609:bool[])
              n233 = Boolean Array To Number(Boolean array=w609) -> (number=w600:u32)
              n234 = To Variant(anything=w600) -> (Variant=w611:variant)
              n235 = Build Array(w611) -> (w610:variant[])
            }
            frame "Write I/O" {
              n236 = Index Array(array=w619) -> (element=w615:variant)  [unwired: 1 in]
              n237 = Variant To Data(error in=w618, type=u8 0, Variant=w615) -> (data=w614:u8, error out=w617:errorcluster)
              n238 = global write "S2C_FPGA_InterfaceGlobals.vi" "C1_P3 Out"(w614) -> ()
            }
          }
        }
        frame "C1/P4" {
          n239 = case "Node or Element Type Case Structure" shown="\"Read I/O\"" w622 {
            tunnel: w627 -> [w632 w646 w651]
            tunnel: [w631 w646 w650] -> w626
            tunnel: w625 -> [w630 w645 w653]
            tunnel: [w629 w645 w653] -> w624
            tunnel: [variant[] [] w643 _] -> w623
            tunnel: w621 -> [_ _ w652]
            frame Default {
              # "5"
              n240 = call <vilib>:"Report Support Error.vi"("sim I/O info in"=w630, "error in (no error)"=w632) -> ("sim I/O info out"=w629:T1, "error out"=w631:errorcluster)  [unwired: 12 out]
            }
            frame "Read I/O" {
              n241 = global read "S2C_FPGA_InterfaceGlobals.vi" "C1/P4/B0"() -> (w641:bool)
              n242 = global read "S2C_FPGA_InterfaceGlobals.vi" "C1/P4/B1"() -> (w638:bool)
              n243 = global read "S2C_FPGA_InterfaceGlobals.vi" "C1/P4/B2"() -> (w636:bool)
              n244 = global read "S2C_FPGA_InterfaceGlobals.vi" "C1/P4/B3"() -> (w635:bool)
              n245 = global read "S2C_FPGA_InterfaceGlobals.vi" "C1/P4/B4"() -> (w634:bool)
              n246 = global read "S2C_FPGA_InterfaceGlobals.vi" "C1/P4/B5"() -> (w637:bool)
              n247 = global read "S2C_FPGA_InterfaceGlobals.vi" "C1/P4/B6"() -> (w639:bool)
              n248 = global read "S2C_FPGA_InterfaceGlobals.vi" "C1/P4/B7"() -> (w640:bool)
              n249 = Build Array(w641, w638, w636, w635, w634, w637, w639, w640) -> (w642:bool[])
              n250 = Boolean Array To Number(Boolean array=w642) -> (number=w633:u32)
              n251 = To Variant(anything=w633) -> (Variant=w644:variant)
              n252 = Build Array(w644) -> (w643:variant[])
            }
            frame "Write I/O" {
              n253 = Index Array(array=w652) -> (element=w648:variant)  [unwired: 1 in]
              n254 = Variant To Data(error in=w651, type=u8 0, Variant=w648) -> (data=w647:u8, error out=w650:errorcluster)
              n255 = global write "S2C_FPGA_InterfaceGlobals.vi" "C1_P4 Out"(w647) -> ()
            }
          }
        }
        frame "C2/P0" {
          n256 = case "Node or Element Type Case Structure" shown="\"Read I/O\"" w655 {
            tunnel: w660 -> [w665 w679 w684]
            tunnel: [w664 w679 w683] -> w659
            tunnel: w658 -> [w663 w678 w686]
            tunnel: [w662 w678 w686] -> w657
            tunnel: [variant[] [] w676 _] -> w656
            tunnel: w654 -> [_ _ w685]
            frame Default {
              # "5"
              n257 = call <vilib>:"Report Support Error.vi"("sim I/O info in"=w663, "error in (no error)"=w665) -> ("sim I/O info out"=w662:T1, "error out"=w664:errorcluster)  [unwired: 12 out]
            }
            frame "Read I/O" {
              n258 = global read "S2C_FPGA_InterfaceGlobals.vi" "C2/P0/B0"() -> (w674:bool)
              n259 = global read "S2C_FPGA_InterfaceGlobals.vi" "C2/P0/B1"() -> (w671:bool)
              n260 = global read "S2C_FPGA_InterfaceGlobals.vi" "C2/P0/B2"() -> (w669:bool)
              n261 = global read "S2C_FPGA_InterfaceGlobals.vi" "C2/P0/B3"() -> (w668:bool)
              n262 = global read "S2C_FPGA_InterfaceGlobals.vi" "C2/P0/B4"() -> (w667:bool)
              n263 = global read "S2C_FPGA_InterfaceGlobals.vi" "C2/P0/B5"() -> (w670:bool)
              n264 = global read "S2C_FPGA_InterfaceGlobals.vi" "C2/P0/B6"() -> (w672:bool)
              n265 = global read "S2C_FPGA_InterfaceGlobals.vi" "C2/P0/B7"() -> (w673:bool)
              n266 = Build Array(w674, w671, w669, w668, w667, w670, w672, w673) -> (w675:bool[])
              n267 = Boolean Array To Number(Boolean array=w675) -> (number=w666:u32)
              n268 = To Variant(anything=w666) -> (Variant=w677:variant)
              n269 = Build Array(w677) -> (w676:variant[])
            }
            frame "Write I/O" {
              n270 = Index Array(array=w685) -> (element=w681:variant)  [unwired: 1 in]
              n271 = Variant To Data(error in=w684, type=u8 0, Variant=w681) -> (data=w680:u8, error out=w683:errorcluster)
              n272 = global write "S2C_FPGA_InterfaceGlobals.vi" "C2_P0 Out"(w680) -> ()
            }
          }
        }
        frame "C2/P1" {
          n273 = case "Node or Element Type Case Structure" shown="\"Read I/O\"" w688 {
            tunnel: w693 -> [w698 w712 w717]
            tunnel: [w697 w712 w716] -> w692
            tunnel: w691 -> [w696 w711 w719]
            tunnel: [w695 w711 w719] -> w690
            tunnel: [variant[] [] w709 _] -> w689
            tunnel: w687 -> [_ _ w718]
            frame Default {
              # "5"
              n274 = call <vilib>:"Report Support Error.vi"("sim I/O info in"=w696, "error in (no error)"=w698) -> ("sim I/O info out"=w695:T1, "error out"=w697:errorcluster)  [unwired: 12 out]
            }
            frame "Read I/O" {
              n275 = global read "S2C_FPGA_InterfaceGlobals.vi" "C2/P1/B0"() -> (w707:bool)
              n276 = global read "S2C_FPGA_InterfaceGlobals.vi" "C2/P1/B1"() -> (w704:bool)
              n277 = global read "S2C_FPGA_InterfaceGlobals.vi" "C2/P1/B2"() -> (w702:bool)
              n278 = global read "S2C_FPGA_InterfaceGlobals.vi" "C2/P1/B3"() -> (w701:bool)
              n279 = global read "S2C_FPGA_InterfaceGlobals.vi" "C2/P1/B4"() -> (w700:bool)
              n280 = global read "S2C_FPGA_InterfaceGlobals.vi" "C2/P1/B5"() -> (w703:bool)
              n281 = global read "S2C_FPGA_InterfaceGlobals.vi" "C2/P1/B6"() -> (w705:bool)
              n282 = global read "S2C_FPGA_InterfaceGlobals.vi" "C2/P1/B7"() -> (w706:bool)
              n283 = Build Array(w707, w704, w702, w701, w700, w703, w705, w706) -> (w708:bool[])
              n284 = Boolean Array To Number(Boolean array=w708) -> (number=w699:u32)
              n285 = To Variant(anything=w699) -> (Variant=w710:variant)
              n286 = Build Array(w710) -> (w709:variant[])
            }
            frame "Write I/O" {
              n287 = Index Array(array=w718) -> (element=w714:variant)  [unwired: 1 in]
              n288 = Variant To Data(error in=w717, type=u8 0, Variant=w714) -> (data=w713:u8, error out=w716:errorcluster)
              n289 = global write "S2C_FPGA_InterfaceGlobals.vi" "C2_P1 Out"(w713) -> ()
            }
          }
        }
        frame "C2/P2" {
          n290 = case "Node or Element Type Case Structure" shown="\"Read I/O\"" w721 {
            tunnel: w726 -> [w731 w745 w750]
            tunnel: [w730 w745 w749] -> w725
            tunnel: w724 -> [w729 w744 w752]
            tunnel: [w728 w744 w752] -> w723
            tunnel: [variant[] [] w742 _] -> w722
            tunnel: w720 -> [_ _ w751]
            frame Default {
              # "5"
              n291 = call <vilib>:"Report Support Error.vi"("sim I/O info in"=w729, "error in (no error)"=w731) -> ("sim I/O info out"=w728:T1, "error out"=w730:errorcluster)  [unwired: 12 out]
            }
            frame "Read I/O" {
              n292 = global read "S2C_FPGA_InterfaceGlobals.vi" "C2/P2/B0"() -> (w740:bool)
              n293 = global read "S2C_FPGA_InterfaceGlobals.vi" "C2/P2/B1"() -> (w737:bool)
              n294 = global read "S2C_FPGA_InterfaceGlobals.vi" "C2/P2/B2"() -> (w735:bool)
              n295 = global read "S2C_FPGA_InterfaceGlobals.vi" "C2/P2/B3"() -> (w734:bool)
              n296 = global read "S2C_FPGA_InterfaceGlobals.vi" "C2/P2/B4"() -> (w733:bool)
              n297 = global read "S2C_FPGA_InterfaceGlobals.vi" "C2/P2/B5"() -> (w736:bool)
              n298 = global read "S2C_FPGA_InterfaceGlobals.vi" "C2/P2/B6"() -> (w738:bool)
              n299 = global read "S2C_FPGA_InterfaceGlobals.vi" "C2/P2/B7"() -> (w739:bool)
              n300 = Build Array(w740, w737, w735, w734, w733, w736, w738, w739) -> (w741:bool[])
              n301 = Boolean Array To Number(Boolean array=w741) -> (number=w732:u32)
              n302 = To Variant(anything=w732) -> (Variant=w743:variant)
              n303 = Build Array(w743) -> (w742:variant[])
            }
            frame "Write I/O" {
              n304 = Index Array(array=w751) -> (element=w747:variant)  [unwired: 1 in]
              n305 = Variant To Data(error in=w750, type=u8 0, Variant=w747) -> (data=w746:u8, error out=w749:errorcluster)
              n306 = global write "S2C_FPGA_InterfaceGlobals.vi" "C2_P2 Out"(w746) -> ()
            }
          }
        }
        frame "C2/P3" {
          n307 = case "Node or Element Type Case Structure" shown="\"Read I/O\"" w754 {
            tunnel: w759 -> [w764 w778 w783]
            tunnel: [w763 w778 w782] -> w758
            tunnel: w757 -> [w762 w777 w785]
            tunnel: [w761 w777 w785] -> w756
            tunnel: [variant[] [] w775 _] -> w755
            tunnel: w753 -> [_ _ w784]
            frame Default {
              # "5"
              n308 = call <vilib>:"Report Support Error.vi"("sim I/O info in"=w762, "error in (no error)"=w764) -> ("sim I/O info out"=w761:T1, "error out"=w763:errorcluster)  [unwired: 12 out]
            }
            frame "Read I/O" {
              n309 = global read "S2C_FPGA_InterfaceGlobals.vi" "C2/P3/B0"() -> (w773:bool)
              n310 = global read "S2C_FPGA_InterfaceGlobals.vi" "C2/P3/B1"() -> (w770:bool)
              n311 = global read "S2C_FPGA_InterfaceGlobals.vi" "C2/P3/B2"() -> (w768:bool)
              n312 = global read "S2C_FPGA_InterfaceGlobals.vi" "C2/P3/B3"() -> (w767:bool)
              n313 = global read "S2C_FPGA_InterfaceGlobals.vi" "C2/P3/B4"() -> (w766:bool)
              n314 = global read "S2C_FPGA_InterfaceGlobals.vi" "C2/P3/B5"() -> (w769:bool)
              n315 = global read "S2C_FPGA_InterfaceGlobals.vi" "C2/P3/B6"() -> (w771:bool)
              n316 = global read "S2C_FPGA_InterfaceGlobals.vi" "C2/P3/B7"() -> (w772:bool)
              n317 = Build Array(w773, w770, w768, w767, w766, w769, w771, w772) -> (w774:bool[])
              n318 = Boolean Array To Number(Boolean array=w774) -> (number=w765:u32)
              n319 = To Variant(anything=w765) -> (Variant=w776:variant)
              n320 = Build Array(w776) -> (w775:variant[])
            }
            frame "Write I/O" {
              n321 = Index Array(array=w784) -> (element=w780:variant)  [unwired: 1 in]
              n322 = Variant To Data(error in=w783, type=u8 0, Variant=w780) -> (data=w779:u8, error out=w782:errorcluster)
              n323 = global write "S2C_FPGA_InterfaceGlobals.vi" "C2_P3 Out"(w779) -> ()
            }
          }
        }
        frame "C2/P4" {
          n324 = case "Node or Element Type Case Structure" shown="\"Read I/O\"" w787 {
            tunnel: w792 -> [w797 w811 w816]
            tunnel: [w796 w811 w815] -> w791
            tunnel: w790 -> [w795 w810 w818]
            tunnel: [w794 w810 w818] -> w789
            tunnel: [variant[] [] w808 _] -> w788
            tunnel: w786 -> [_ _ w817]
            frame Default {
              # "5"
              n325 = call <vilib>:"Report Support Error.vi"("sim I/O info in"=w795, "error in (no error)"=w797) -> ("sim I/O info out"=w794:T1, "error out"=w796:errorcluster)  [unwired: 12 out]
            }
            frame "Read I/O" {
              n326 = global read "S2C_FPGA_InterfaceGlobals.vi" "C2/P4/B0"() -> (w806:bool)
              n327 = global read "S2C_FPGA_InterfaceGlobals.vi" "C2/P4/B1"() -> (w803:bool)
              n328 = global read "S2C_FPGA_InterfaceGlobals.vi" "C2/P4/B2"() -> (w801:bool)
              n329 = global read "S2C_FPGA_InterfaceGlobals.vi" "C2/P4/B3"() -> (w800:bool)
              n330 = global read "S2C_FPGA_InterfaceGlobals.vi" "C2/P4/B4"() -> (w799:bool)
              n331 = global read "S2C_FPGA_InterfaceGlobals.vi" "C2/P4/B5"() -> (w802:bool)
              n332 = global read "S2C_FPGA_InterfaceGlobals.vi" "C2/P4/B6"() -> (w804:bool)
              n333 = global read "S2C_FPGA_InterfaceGlobals.vi" "C2/P4/B7"() -> (w805:bool)
              n334 = Build Array(w806, w803, w801, w800, w799, w802, w804, w805) -> (w807:bool[])
              n335 = Boolean Array To Number(Boolean array=w807) -> (number=w798:u32)
              n336 = To Variant(anything=w798) -> (Variant=w809:variant)
              n337 = Build Array(w809) -> (w808:variant[])
            }
            frame "Write I/O" {
              n338 = Index Array(array=w817) -> (element=w813:variant)  [unwired: 1 in]
              n339 = Variant To Data(error in=w816, type=u8 0, Variant=w813) -> (data=w812:u8, error out=w815:errorcluster)
              n340 = global write "S2C_FPGA_InterfaceGlobals.vi" "C2_P4 Out"(w812) -> ()
            }
          }
        }
        frame "C0/P0/B0" {
          n341 = case "Node or Element Type Case Structure" shown="\"Read I/O\"" w820 {
            tunnel: w825 -> [w830 w835 w840]
            tunnel: [w829 w835 w839] -> w824
            tunnel: w823 -> [w828 w834 w842]
            tunnel: [w827 w834 w842] -> w822
            tunnel: [variant[] [] w831 _] -> w821
            tunnel: w819 -> [_ _ w841]
            frame Default {
              # "5"
              n342 = call <vilib>:"Report Support Error.vi"("sim I/O info in"=w828, "error in (no error)"=w830) -> ("sim I/O info out"=w827:T1, "error out"=w829:errorcluster)  [unwired: 12 out]
            }
            frame "Read I/O" {
              n343 = global read "S2C_FPGA_InterfaceGlobals.vi" "C0/P0/B0"() -> (w833:bool)
              n344 = To Variant(anything=w833) -> (Variant=w832:variant)
              n345 = Build Array(w832) -> (w831:variant[])
            }
            frame "Write I/O" {
              n346 = Index Array(array=w841) -> (element=w837:variant)  [unwired: 1 in]
              n347 = Variant To Data(error in=w840, type=TRUE, Variant=w837) -> (data=w836:bool, error out=w839:errorcluster)
              n348 = global write "S2C_FPGA_InterfaceGlobals.vi" "C0/P0/B0"(w836) -> ()
            }
          }
        }
        frame "C0/P0/B1" {
          n349 = case "Node or Element Type Case Structure" shown="\"Write I/O\"" w844 {
            tunnel: w849 -> [w854 w859 w864]
            tunnel: [w853 w859 w863] -> w848
            tunnel: w847 -> [w852 w858 w866]
            tunnel: [w851 w858 w866] -> w846
            tunnel: [variant[] [] w855 _] -> w845
            tunnel: w843 -> [_ _ w865]
            frame Default {
              # "5"
              n350 = call <vilib>:"Report Support Error.vi"("sim I/O info in"=w852, "error in (no error)"=w854) -> ("sim I/O info out"=w851:T1, "error out"=w853:errorcluster)  [unwired: 12 out]
            }
            frame "Read I/O" {
              n351 = global read "S2C_FPGA_InterfaceGlobals.vi" "C0/P0/B1"() -> (w857:bool)
              n352 = To Variant(anything=w857) -> (Variant=w856:variant)
              n353 = Build Array(w856) -> (w855:variant[])
            }
            frame "Write I/O" {
              n354 = Index Array(array=w865) -> (element=w861:variant)  [unwired: 1 in]
              n355 = Variant To Data(error in=w864, type=TRUE, Variant=w861) -> (data=w860:bool, error out=w863:errorcluster)
              n356 = global write "S2C_FPGA_InterfaceGlobals.vi" "C0/P0/B1"(w860) -> ()
            }
          }
        }
        frame "C0/P0/B2" {
          n357 = case "Node or Element Type Case Structure" shown="\"Write I/O\"" w868 {
            tunnel: w873 -> [w878 w883 w888]
            tunnel: [w877 w883 w887] -> w872
            tunnel: w871 -> [w876 w882 w890]
            tunnel: [w875 w882 w890] -> w870
            tunnel: [variant[] [] w879 _] -> w869
            tunnel: w867 -> [_ _ w889]
            frame Default {
              # "5"
              n358 = call <vilib>:"Report Support Error.vi"("sim I/O info in"=w876, "error in (no error)"=w878) -> ("sim I/O info out"=w875:T1, "error out"=w877:errorcluster)  [unwired: 12 out]
            }
            frame "Read I/O" {
              n359 = global read "S2C_FPGA_InterfaceGlobals.vi" "C0/P0/B2"() -> (w880:bool)
              n360 = To Variant(anything=w880) -> (Variant=w881:variant)
              n361 = Build Array(w881) -> (w879:variant[])
            }
            frame "Write I/O" {
              n362 = Index Array(array=w889) -> (element=w885:variant)  [unwired: 1 in]
              n363 = Variant To Data(error in=w888, type=TRUE, Variant=w885) -> (data=w884:bool, error out=w887:errorcluster)
              n364 = global write "S2C_FPGA_InterfaceGlobals.vi" "C0/P0/B2"(w884) -> ()
            }
          }
        }
        frame "C0/P0/B3" {
          n365 = case "Node or Element Type Case Structure" shown="\"Read I/O\"" w892 {
            tunnel: w897 -> [w902 w907 w912]
            tunnel: [w901 w907 w911] -> w896
            tunnel: w895 -> [w900 w906 w914]
            tunnel: [w899 w906 w914] -> w894
            tunnel: [variant[] [] w903 _] -> w893
            tunnel: w891 -> [_ _ w913]
            frame Default {
              # "5"
              n366 = call <vilib>:"Report Support Error.vi"("sim I/O info in"=w900, "error in (no error)"=w902) -> ("sim I/O info out"=w899:T1, "error out"=w901:errorcluster)  [unwired: 12 out]
            }
            frame "Read I/O" {
              n367 = global read "S2C_FPGA_InterfaceGlobals.vi" "C0/P0/B3"() -> (w905:bool)
              n368 = To Variant(anything=w905) -> (Variant=w904:variant)
              n369 = Build Array(w904) -> (w903:variant[])
            }
            frame "Write I/O" {
              n370 = Index Array(array=w913) -> (element=w909:variant)  [unwired: 1 in]
              n371 = Variant To Data(error in=w912, type=TRUE, Variant=w909) -> (data=w908:bool, error out=w911:errorcluster)
              n372 = global write "S2C_FPGA_InterfaceGlobals.vi" "C0/P0/B3"(w908) -> ()
            }
          }
        }
        frame "C0/P0/B4" {
          n373 = case "Node or Element Type Case Structure" shown="\"Read I/O\"" w916 {
            tunnel: w921 -> [w926 w931 w936]
            tunnel: [w925 w931 w935] -> w920
            tunnel: w919 -> [w924 w930 w938]
            tunnel: [w923 w930 w938] -> w918
            tunnel: [variant[] [] w927 _] -> w917
            tunnel: w915 -> [_ _ w937]
            frame Default {
              # "5"
              n374 = call <vilib>:"Report Support Error.vi"("sim I/O info in"=w924, "error in (no error)"=w926) -> ("sim I/O info out"=w923:T1, "error out"=w925:errorcluster)  [unwired: 12 out]
            }
            frame "Read I/O" {
              n375 = global read "S2C_FPGA_InterfaceGlobals.vi" "C0/P0/B4"() -> (w929:bool)
              n376 = To Variant(anything=w929) -> (Variant=w928:variant)
              n377 = Build Array(w928) -> (w927:variant[])
            }
            frame "Write I/O" {
              n378 = Index Array(array=w937) -> (element=w933:variant)  [unwired: 1 in]
              n379 = Variant To Data(error in=w936, type=TRUE, Variant=w933) -> (data=w932:bool, error out=w935:errorcluster)
              n380 = global write "S2C_FPGA_InterfaceGlobals.vi" "C0/P0/B4"(w932) -> ()
            }
          }
        }
        frame "C0/P0/B5" {
          n381 = case "Node or Element Type Case Structure" shown="\"Read I/O\"" w940 {
            tunnel: w945 -> [w950 w955 w960]
            tunnel: [w949 w955 w959] -> w944
            tunnel: w943 -> [w948 w954 w962]
            tunnel: [w947 w954 w962] -> w942
            tunnel: [variant[] [] w951 _] -> w941
            tunnel: w939 -> [_ _ w961]
            frame Default {
              # "5"
              n382 = call <vilib>:"Report Support Error.vi"("sim I/O info in"=w948, "error in (no error)"=w950) -> ("sim I/O info out"=w947:T1, "error out"=w949:errorcluster)  [unwired: 12 out]
            }
            frame "Read I/O" {
              n383 = global read "S2C_FPGA_InterfaceGlobals.vi" "C0/P0/B5"() -> (w953:bool)
              n384 = To Variant(anything=w953) -> (Variant=w952:variant)
              n385 = Build Array(w952) -> (w951:variant[])
            }
            frame "Write I/O" {
              n386 = Index Array(array=w961) -> (element=w957:variant)  [unwired: 1 in]
              n387 = Variant To Data(error in=w960, type=TRUE, Variant=w957) -> (data=w956:bool, error out=w959:errorcluster)
              n388 = global write "S2C_FPGA_InterfaceGlobals.vi" "C0/P0/B5"(w956) -> ()
            }
          }
        }
        frame "C0/P0/B6" {
          n389 = case "Node or Element Type Case Structure" shown="\"Read I/O\"" w964 {
            tunnel: w969 -> [w974 w979 w984]
            tunnel: [w973 w979 w983] -> w968
            tunnel: w967 -> [w972 w978 w986]
            tunnel: [w971 w978 w986] -> w966
            tunnel: [variant[] [] w975 _] -> w965
            tunnel: w963 -> [_ _ w985]
            frame Default {
              # "5"
              n390 = call <vilib>:"Report Support Error.vi"("sim I/O info in"=w972, "error in (no error)"=w974) -> ("sim I/O info out"=w971:T1, "error out"=w973:errorcluster)  [unwired: 12 out]
            }
            frame "Read I/O" {
              n391 = global read "S2C_FPGA_InterfaceGlobals.vi" "C0/P0/B6"() -> (w977:bool)
              n392 = To Variant(anything=w977) -> (Variant=w976:variant)
              n393 = Build Array(w976) -> (w975:variant[])
            }
            frame "Write I/O" {
              n394 = Index Array(array=w985) -> (element=w981:variant)  [unwired: 1 in]
              n395 = Variant To Data(error in=w984, type=TRUE, Variant=w981) -> (data=w980:bool, error out=w983:errorcluster)
              n396 = global write "S2C_FPGA_InterfaceGlobals.vi" "C0/P0/B6"(w980) -> ()
            }
          }
        }
        frame "C0/P0/B7" {
          n397 = case "Node or Element Type Case Structure" shown="\"Read I/O\"" w988 {
            tunnel: w993 -> [w998 w1003 w1008]
            tunnel: [w997 w1003 w1007] -> w992
            tunnel: w991 -> [w996 w1002 w1010]
            tunnel: [w995 w1002 w1010] -> w990
            tunnel: [variant[] [] w999 _] -> w989
            tunnel: w987 -> [_ _ w1009]
            frame Default {
              # "5"
              n398 = call <vilib>:"Report Support Error.vi"("sim I/O info in"=w996, "error in (no error)"=w998) -> ("sim I/O info out"=w995:T1, "error out"=w997:errorcluster)  [unwired: 12 out]
            }
            frame "Read I/O" {
              n399 = global read "S2C_FPGA_InterfaceGlobals.vi" "C0/P0/B7"() -> (w1001:bool)
              n400 = To Variant(anything=w1001) -> (Variant=w1000:variant)
              n401 = Build Array(w1000) -> (w999:variant[])
            }
            frame "Write I/O" {
              n402 = Index Array(array=w1009) -> (element=w1005:variant)  [unwired: 1 in]
              n403 = Variant To Data(error in=w1008, type=TRUE, Variant=w1005) -> (data=w1004:bool, error out=w1007:errorcluster)
              n404 = global write "S2C_FPGA_InterfaceGlobals.vi" "C0/P0/B7"(w1004) -> ()
            }
          }
        }
        frame "C0/P1/B0" {
          n405 = case "Node or Element Type Case Structure" shown="\"Read I/O\"" w1012 {
            tunnel: w1017 -> [w1022 w1027 w1032]
            tunnel: [w1021 w1027 w1031] -> w1016
            tunnel: w1015 -> [w1020 w1026 w1034]
            tunnel: [w1019 w1026 w1034] -> w1014
            tunnel: [variant[] [] w1023 _] -> w1013
            tunnel: w1011 -> [_ _ w1033]
            frame Default {
              # "5"
              n406 = call <vilib>:"Report Support Error.vi"("sim I/O info in"=w1020, "error in (no error)"=w1022) -> ("sim I/O info out"=w1019:T1, "error out"=w1021:errorcluster)  [unwired: 12 out]
            }
            frame "Read I/O" {
              n407 = global read "S2C_FPGA_InterfaceGlobals.vi" "C0/P1/B0"() -> (w1025:bool)
              n408 = To Variant(anything=w1025) -> (Variant=w1024:variant)
              n409 = Build Array(w1024) -> (w1023:variant[])
            }
            frame "Write I/O" {
              n410 = Index Array(array=w1033) -> (element=w1029:variant)  [unwired: 1 in]
              n411 = Variant To Data(error in=w1032, type=TRUE, Variant=w1029) -> (data=w1028:bool, error out=w1031:errorcluster)
              n412 = global write "S2C_FPGA_InterfaceGlobals.vi" "C0/P1/B0"(w1028) -> ()
            }
          }
        }
        frame "C0/P1/B1" {
          n413 = case "Node or Element Type Case Structure" shown="\"Read I/O\"" w1036 {
            tunnel: w1041 -> [w1046 w1051 w1056]
            tunnel: [w1045 w1051 w1055] -> w1040
            tunnel: w1039 -> [w1044 w1050 w1058]
            tunnel: [w1043 w1050 w1058] -> w1038
            tunnel: [variant[] [] w1047 _] -> w1037
            tunnel: w1035 -> [_ _ w1057]
            frame Default {
              # "5"
              n414 = call <vilib>:"Report Support Error.vi"("sim I/O info in"=w1044, "error in (no error)"=w1046) -> ("sim I/O info out"=w1043:T1, "error out"=w1045:errorcluster)  [unwired: 12 out]
            }
            frame "Read I/O" {
              n415 = global read "S2C_FPGA_InterfaceGlobals.vi" "C0/P1/B1"() -> (w1049:bool)
              n416 = To Variant(anything=w1049) -> (Variant=w1048:variant)
              n417 = Build Array(w1048) -> (w1047:variant[])
            }
            frame "Write I/O" {
              n418 = Index Array(array=w1057) -> (element=w1053:variant)  [unwired: 1 in]
              n419 = Variant To Data(error in=w1056, type=TRUE, Variant=w1053) -> (data=w1052:bool, error out=w1055:errorcluster)
              n420 = global write "S2C_FPGA_InterfaceGlobals.vi" "C0/P1/B1"(w1052) -> ()
            }
          }
        }
        frame "C0/P1/B2" {
          n421 = case "Node or Element Type Case Structure" shown="\"Read I/O\"" w1060 {
            tunnel: w1065 -> [w1070 w1075 w1080]
            tunnel: [w1069 w1075 w1079] -> w1064
            tunnel: w1063 -> [w1068 w1074 w1082]
            tunnel: [w1067 w1074 w1082] -> w1062
            tunnel: [variant[] [] w1071 _] -> w1061
            tunnel: w1059 -> [_ _ w1081]
            frame Default {
              # "5"
              n422 = call <vilib>:"Report Support Error.vi"("sim I/O info in"=w1068, "error in (no error)"=w1070) -> ("sim I/O info out"=w1067:T1, "error out"=w1069:errorcluster)  [unwired: 12 out]
            }
            frame "Read I/O" {
              n423 = global read "S2C_FPGA_InterfaceGlobals.vi" "C0/P1/B2"() -> (w1073:bool)
              n424 = To Variant(anything=w1073) -> (Variant=w1072:variant)
              n425 = Build Array(w1072) -> (w1071:variant[])
            }
            frame "Write I/O" {
              n426 = Index Array(array=w1081) -> (element=w1077:variant)  [unwired: 1 in]
              n427 = Variant To Data(error in=w1080, type=TRUE, Variant=w1077) -> (data=w1076:bool, error out=w1079:errorcluster)
              n428 = global write "S2C_FPGA_InterfaceGlobals.vi" "C0/P1/B2"(w1076) -> ()
            }
          }
        }
        frame "C0/P1/B3" {
          n429 = case "Node or Element Type Case Structure" shown="\"Read I/O\"" w1084 {
            tunnel: w1089 -> [w1094 w1099 w1104]
            tunnel: [w1093 w1099 w1103] -> w1088
            tunnel: w1087 -> [w1092 w1098 w1106]
            tunnel: [w1091 w1098 w1106] -> w1086
            tunnel: [variant[] [] w1095 _] -> w1085
            tunnel: w1083 -> [_ _ w1105]
            frame Default {
              # "5"
              n430 = call <vilib>:"Report Support Error.vi"("sim I/O info in"=w1092, "error in (no error)"=w1094) -> ("sim I/O info out"=w1091:T1, "error out"=w1093:errorcluster)  [unwired: 12 out]
            }
            frame "Read I/O" {
              n431 = global read "S2C_FPGA_InterfaceGlobals.vi" "C0/P1/B3"() -> (w1097:bool)
              n432 = To Variant(anything=w1097) -> (Variant=w1096:variant)
              n433 = Build Array(w1096) -> (w1095:variant[])
            }
            frame "Write I/O" {
              n434 = Index Array(array=w1105) -> (element=w1101:variant)  [unwired: 1 in]
              n435 = Variant To Data(error in=w1104, type=TRUE, Variant=w1101) -> (data=w1100:bool, error out=w1103:errorcluster)
              n436 = global write "S2C_FPGA_InterfaceGlobals.vi" "C0/P1/B3"(w1100) -> ()
            }
          }
        }
        frame "C0/P1/B4" {
          n437 = case "Node or Element Type Case Structure" shown="\"Read I/O\"" w1108 {
            tunnel: w1113 -> [w1118 w1123 w1128]
            tunnel: [w1117 w1123 w1127] -> w1112
            tunnel: w1111 -> [w1116 w1122 w1130]
            tunnel: [w1115 w1122 w1130] -> w1110
            tunnel: [variant[] [] w1119 _] -> w1109
            tunnel: w1107 -> [_ _ w1129]
            frame Default {
              # "5"
              n438 = call <vilib>:"Report Support Error.vi"("sim I/O info in"=w1116, "error in (no error)"=w1118) -> ("sim I/O info out"=w1115:T1, "error out"=w1117:errorcluster)  [unwired: 12 out]
            }
            frame "Read I/O" {
              n439 = global read "S2C_FPGA_InterfaceGlobals.vi" "C0/P1/B4"() -> (w1121:bool)
              n440 = To Variant(anything=w1121) -> (Variant=w1120:variant)
              n441 = Build Array(w1120) -> (w1119:variant[])
            }
            frame "Write I/O" {
              n442 = Index Array(array=w1129) -> (element=w1125:variant)  [unwired: 1 in]
              n443 = Variant To Data(error in=w1128, type=TRUE, Variant=w1125) -> (data=w1124:bool, error out=w1127:errorcluster)
              n444 = global write "S2C_FPGA_InterfaceGlobals.vi" "C0/P1/B4"(w1124) -> ()
            }
          }
        }
        frame "C0/P1/B5" {
          n445 = case "Node or Element Type Case Structure" shown="\"Read I/O\"" w1132 {
            tunnel: w1137 -> [w1142 w1147 w1152]
            tunnel: [w1141 w1147 w1151] -> w1136
            tunnel: w1135 -> [w1140 w1146 w1154]
            tunnel: [w1139 w1146 w1154] -> w1134
            tunnel: [variant[] [] w1143 _] -> w1133
            tunnel: w1131 -> [_ _ w1153]
            frame Default {
              # "5"
              n446 = call <vilib>:"Report Support Error.vi"("sim I/O info in"=w1140, "error in (no error)"=w1142) -> ("sim I/O info out"=w1139:T1, "error out"=w1141:errorcluster)  [unwired: 12 out]
            }
            frame "Read I/O" {
              n447 = global read "S2C_FPGA_InterfaceGlobals.vi" "C0/P1/B5"() -> (w1145:bool)
              n448 = To Variant(anything=w1145) -> (Variant=w1144:variant)
              n449 = Build Array(w1144) -> (w1143:variant[])
            }
            frame "Write I/O" {
              n450 = Index Array(array=w1153) -> (element=w1149:variant)  [unwired: 1 in]
              n451 = Variant To Data(error in=w1152, type=TRUE, Variant=w1149) -> (data=w1148:bool, error out=w1151:errorcluster)
              n452 = global write "S2C_FPGA_InterfaceGlobals.vi" "C0/P1/B5"(w1148) -> ()
            }
          }
        }
        frame "C0/P1/B6" {
          n453 = case "Node or Element Type Case Structure" shown="\"Read I/O\"" w1156 {
            tunnel: w1161 -> [w1166 w1171 w1176]
            tunnel: [w1165 w1171 w1175] -> w1160
            tunnel: w1159 -> [w1164 w1170 w1178]
            tunnel: [w1163 w1170 w1178] -> w1158
            tunnel: [variant[] [] w1167 _] -> w1157
            tunnel: w1155 -> [_ _ w1177]
            frame Default {
              # "5"
              n454 = call <vilib>:"Report Support Error.vi"("sim I/O info in"=w1164, "error in (no error)"=w1166) -> ("sim I/O info out"=w1163:T1, "error out"=w1165:errorcluster)  [unwired: 12 out]
            }
            frame "Read I/O" {
              n455 = global read "S2C_FPGA_InterfaceGlobals.vi" "C0/P1/B6"() -> (w1169:bool)
              n456 = To Variant(anything=w1169) -> (Variant=w1168:variant)
              n457 = Build Array(w1168) -> (w1167:variant[])
            }
            frame "Write I/O" {
              n458 = Index Array(array=w1177) -> (element=w1173:variant)  [unwired: 1 in]
              n459 = Variant To Data(error in=w1176, type=TRUE, Variant=w1173) -> (data=w1172:bool, error out=w1175:errorcluster)
              n460 = global write "S2C_FPGA_InterfaceGlobals.vi" "C0/P1/B6"(w1172) -> ()
            }
          }
        }
        frame "C0/P1/B7" {
          n461 = case "Node or Element Type Case Structure" shown="\"Write I/O\"" w1180 {
            tunnel: w1185 -> [w1190 w1195 w1200]
            tunnel: [w1189 w1195 w1199] -> w1184
            tunnel: w1183 -> [w1188 w1194 w1202]
            tunnel: [w1187 w1194 w1202] -> w1182
            tunnel: [variant[] [] w1191 _] -> w1181
            tunnel: w1179 -> [_ _ w1201]
            frame Default {
              # "5"
              n462 = call <vilib>:"Report Support Error.vi"("sim I/O info in"=w1188, "error in (no error)"=w1190) -> ("sim I/O info out"=w1187:T1, "error out"=w1189:errorcluster)  [unwired: 12 out]
            }
            frame "Read I/O" {
              n463 = global read "S2C_FPGA_InterfaceGlobals.vi" "C0/P1/B7"() -> (w1193:bool)
              n464 = To Variant(anything=w1193) -> (Variant=w1192:variant)
              n465 = Build Array(w1192) -> (w1191:variant[])
            }
            frame "Write I/O" {
              n466 = Index Array(array=w1201) -> (element=w1197:variant)  [unwired: 1 in]
              n467 = Variant To Data(error in=w1200, type=TRUE, Variant=w1197) -> (data=w1196:bool, error out=w1199:errorcluster)
              n468 = global write "S2C_FPGA_InterfaceGlobals.vi" "C0/P1/B7"(w1196) -> ()
            }
          }
        }
        frame "C1/P0/B0" {
          n469 = case "Node or Element Type Case Structure" shown="\"Read I/O\"" w1204 {
            tunnel: w1209 -> [w1214 w1219 w1224]
            tunnel: [w1213 w1219 w1223] -> w1208
            tunnel: w1207 -> [w1212 w1218 w1226]
            tunnel: [w1211 w1218 w1226] -> w1206
            tunnel: [variant[] [] w1215 _] -> w1205
            tunnel: w1203 -> [_ _ w1225]
            frame Default {
              # "5"
              n470 = call <vilib>:"Report Support Error.vi"("sim I/O info in"=w1212, "error in (no error)"=w1214) -> ("sim I/O info out"=w1211:T1, "error out"=w1213:errorcluster)  [unwired: 12 out]
            }
            frame "Read I/O" {
              n471 = global read "S2C_FPGA_InterfaceGlobals.vi" "C1/P0/B0"() -> (w1217:bool)
              n472 = To Variant(anything=w1217) -> (Variant=w1216:variant)
              n473 = Build Array(w1216) -> (w1215:variant[])
            }
            frame "Write I/O" {
              n474 = Index Array(array=w1225) -> (element=w1221:variant)  [unwired: 1 in]
              n475 = Variant To Data(error in=w1224, type=TRUE, Variant=w1221) -> (data=w1220:bool, error out=w1223:errorcluster)
              n476 = global write "S2C_FPGA_InterfaceGlobals.vi" "C1/P0/B0"(w1220) -> ()
            }
          }
        }
        frame "C1/P0/B1" {
          n477 = case "Node or Element Type Case Structure" shown="\"Read I/O\"" w1228 {
            tunnel: w1233 -> [w1238 w1243 w1248]
            tunnel: [w1237 w1243 w1247] -> w1232
            tunnel: w1231 -> [w1236 w1242 w1250]
            tunnel: [w1235 w1242 w1250] -> w1230
            tunnel: [variant[] [] w1239 _] -> w1229
            tunnel: w1227 -> [_ _ w1249]
            frame Default {
              # "5"
              n478 = call <vilib>:"Report Support Error.vi"("sim I/O info in"=w1236, "error in (no error)"=w1238) -> ("sim I/O info out"=w1235:T1, "error out"=w1237:errorcluster)  [unwired: 12 out]
            }
            frame "Read I/O" {
              n479 = global read "S2C_FPGA_InterfaceGlobals.vi" "C1/P0/B1"() -> (w1241:bool)
              n480 = To Variant(anything=w1241) -> (Variant=w1240:variant)
              n481 = Build Array(w1240) -> (w1239:variant[])
            }
            frame "Write I/O" {
              n482 = Index Array(array=w1249) -> (element=w1245:variant)  [unwired: 1 in]
              n483 = Variant To Data(error in=w1248, type=TRUE, Variant=w1245) -> (data=w1244:bool, error out=w1247:errorcluster)
              n484 = global write "S2C_FPGA_InterfaceGlobals.vi" "C1/P0/B1"(w1244) -> ()
            }
          }
        }
        frame "C1/P0/B2" {
          n485 = case "Node or Element Type Case Structure" shown="\"Read I/O\"" w1252 {
            tunnel: w1257 -> [w1262 w1267 w1272]
            tunnel: [w1261 w1267 w1271] -> w1256
            tunnel: w1255 -> [w1260 w1266 w1274]
            tunnel: [w1259 w1266 w1274] -> w1254
            tunnel: [variant[] [] w1263 _] -> w1253
            tunnel: w1251 -> [_ _ w1273]
            frame Default {
              # "5"
              n486 = call <vilib>:"Report Support Error.vi"("sim I/O info in"=w1260, "error in (no error)"=w1262) -> ("sim I/O info out"=w1259:T1, "error out"=w1261:errorcluster)  [unwired: 12 out]
            }
            frame "Read I/O" {
              n487 = global read "S2C_FPGA_InterfaceGlobals.vi" "C1/P0/B2"() -> (w1265:bool)
              n488 = To Variant(anything=w1265) -> (Variant=w1264:variant)
              n489 = Build Array(w1264) -> (w1263:variant[])
            }
            frame "Write I/O" {
              n490 = Index Array(array=w1273) -> (element=w1269:variant)  [unwired: 1 in]
              n491 = Variant To Data(error in=w1272, type=TRUE, Variant=w1269) -> (data=w1268:bool, error out=w1271:errorcluster)
              n492 = global write "S2C_FPGA_InterfaceGlobals.vi" "C1/P0/B2"(w1268) -> ()
            }
          }
        }
        frame "C1/P0/B3" {
          n493 = case "Node or Element Type Case Structure" shown="\"Read I/O\"" w1276 {
            tunnel: w1281 -> [w1286 w1291 w1296]
            tunnel: [w1285 w1291 w1295] -> w1280
            tunnel: w1279 -> [w1284 w1290 w1298]
            tunnel: [w1283 w1290 w1298] -> w1278
            tunnel: [variant[] [] w1287 _] -> w1277
            tunnel: w1275 -> [_ _ w1297]
            frame Default {
              # "5"
              n494 = call <vilib>:"Report Support Error.vi"("sim I/O info in"=w1284, "error in (no error)"=w1286) -> ("sim I/O info out"=w1283:T1, "error out"=w1285:errorcluster)  [unwired: 12 out]
            }
            frame "Read I/O" {
              n495 = global read "S2C_FPGA_InterfaceGlobals.vi" "C1/P0/B3"() -> (w1289:bool)
              n496 = To Variant(anything=w1289) -> (Variant=w1288:variant)
              n497 = Build Array(w1288) -> (w1287:variant[])
            }
            frame "Write I/O" {
              n498 = Index Array(array=w1297) -> (element=w1293:variant)  [unwired: 1 in]
              n499 = Variant To Data(error in=w1296, type=TRUE, Variant=w1293) -> (data=w1292:bool, error out=w1295:errorcluster)
              n500 = global write "S2C_FPGA_InterfaceGlobals.vi" "C1/P0/B3"(w1292) -> ()
            }
          }
        }
        frame "C1/P0/B4" {
          n501 = case "Node or Element Type Case Structure" shown="\"Read I/O\"" w1300 {
            tunnel: w1305 -> [w1310 w1315 w1320]
            tunnel: [w1309 w1315 w1319] -> w1304
            tunnel: w1303 -> [w1308 w1314 w1322]
            tunnel: [w1307 w1314 w1322] -> w1302
            tunnel: [variant[] [] w1311 _] -> w1301
            tunnel: w1299 -> [_ _ w1321]
            frame Default {
              # "5"
              n502 = call <vilib>:"Report Support Error.vi"("sim I/O info in"=w1308, "error in (no error)"=w1310) -> ("sim I/O info out"=w1307:T1, "error out"=w1309:errorcluster)  [unwired: 12 out]
            }
            frame "Read I/O" {
              n503 = global read "S2C_FPGA_InterfaceGlobals.vi" "C1/P0/B4"() -> (w1313:bool)
              n504 = To Variant(anything=w1313) -> (Variant=w1312:variant)
              n505 = Build Array(w1312) -> (w1311:variant[])
            }
            frame "Write I/O" {
              n506 = Index Array(array=w1321) -> (element=w1317:variant)  [unwired: 1 in]
              n507 = Variant To Data(error in=w1320, type=TRUE, Variant=w1317) -> (data=w1316:bool, error out=w1319:errorcluster)
              n508 = global write "S2C_FPGA_InterfaceGlobals.vi" "C1/P0/B4"(w1316) -> ()
            }
          }
        }
        frame "C1/P0/B5" {
          n509 = case "Node or Element Type Case Structure" shown="\"Read I/O\"" w1324 {
            tunnel: w1329 -> [w1334 w1339 w1344]
            tunnel: [w1333 w1339 w1343] -> w1328
            tunnel: w1327 -> [w1332 w1338 w1346]
            tunnel: [w1331 w1338 w1346] -> w1326
            tunnel: [variant[] [] w1335 _] -> w1325
            tunnel: w1323 -> [_ _ w1345]
            frame Default {
              # "5"
              n510 = call <vilib>:"Report Support Error.vi"("sim I/O info in"=w1332, "error in (no error)"=w1334) -> ("sim I/O info out"=w1331:T1, "error out"=w1333:errorcluster)  [unwired: 12 out]
            }
            frame "Read I/O" {
              n511 = global read "S2C_FPGA_InterfaceGlobals.vi" "C1/P0/B5"() -> (w1337:bool)
              n512 = To Variant(anything=w1337) -> (Variant=w1336:variant)
              n513 = Build Array(w1336) -> (w1335:variant[])
            }
            frame "Write I/O" {
              n514 = Index Array(array=w1345) -> (element=w1341:variant)  [unwired: 1 in]
              n515 = Variant To Data(error in=w1344, type=TRUE, Variant=w1341) -> (data=w1340:bool, error out=w1343:errorcluster)
              n516 = global write "S2C_FPGA_InterfaceGlobals.vi" "C1/P0/B5"(w1340) -> ()
            }
          }
        }
        frame "C1/P0/B6" {
          n517 = case "Node or Element Type Case Structure" shown="\"Read I/O\"" w1348 {
            tunnel: w1353 -> [w1358 w1363 w1368]
            tunnel: [w1357 w1363 w1367] -> w1352
            tunnel: w1351 -> [w1356 w1362 w1370]
            tunnel: [w1355 w1362 w1370] -> w1350
            tunnel: [variant[] [] w1359 _] -> w1349
            tunnel: w1347 -> [_ _ w1369]
            frame Default {
              # "5"
              n518 = call <vilib>:"Report Support Error.vi"("sim I/O info in"=w1356, "error in (no error)"=w1358) -> ("sim I/O info out"=w1355:T1, "error out"=w1357:errorcluster)  [unwired: 12 out]
            }
            frame "Read I/O" {
              n519 = global read "S2C_FPGA_InterfaceGlobals.vi" "C1/P0/B6"() -> (w1361:bool)
              n520 = To Variant(anything=w1361) -> (Variant=w1360:variant)
              n521 = Build Array(w1360) -> (w1359:variant[])
            }
            frame "Write I/O" {
              n522 = Index Array(array=w1369) -> (element=w1365:variant)  [unwired: 1 in]
              n523 = Variant To Data(error in=w1368, type=TRUE, Variant=w1365) -> (data=w1364:bool, error out=w1367:errorcluster)
              n524 = global write "S2C_FPGA_InterfaceGlobals.vi" "C1/P0/B6"(w1364) -> ()
            }
          }
        }
        frame "C1/P0/B7" {
          n525 = case "Node or Element Type Case Structure" shown="\"Read I/O\"" w1372 {
            tunnel: w1377 -> [w1382 w1387 w1392]
            tunnel: [w1381 w1387 w1391] -> w1376
            tunnel: w1375 -> [w1380 w1386 w1394]
            tunnel: [w1379 w1386 w1394] -> w1374
            tunnel: [variant[] [] w1383 _] -> w1373
            tunnel: w1371 -> [_ _ w1393]
            frame Default {
              # "5"
              n526 = call <vilib>:"Report Support Error.vi"("sim I/O info in"=w1380, "error in (no error)"=w1382) -> ("sim I/O info out"=w1379:T1, "error out"=w1381:errorcluster)  [unwired: 12 out]
            }
            frame "Read I/O" {
              n527 = global read "S2C_FPGA_InterfaceGlobals.vi" "C1/P0/B7"() -> (w1385:bool)
              n528 = To Variant(anything=w1385) -> (Variant=w1384:variant)
              n529 = Build Array(w1384) -> (w1383:variant[])
            }
            frame "Write I/O" {
              n530 = Index Array(array=w1393) -> (element=w1389:variant)  [unwired: 1 in]
              n531 = Variant To Data(error in=w1392, type=TRUE, Variant=w1389) -> (data=w1388:bool, error out=w1391:errorcluster)
              n532 = global write "S2C_FPGA_InterfaceGlobals.vi" "C1/P0/B7"(w1388) -> ()
            }
          }
        }
        frame "C1/P1/B0" {
          n533 = case "Node or Element Type Case Structure" shown="\"Read I/O\"" w1396 {
            tunnel: w1401 -> [w1406 w1411 w1416]
            tunnel: [w1405 w1411 w1415] -> w1400
            tunnel: w1399 -> [w1404 w1410 w1418]
            tunnel: [w1403 w1410 w1418] -> w1398
            tunnel: [variant[] [] w1407 _] -> w1397
            tunnel: w1395 -> [_ _ w1417]
            frame Default {
              # "5"
              n534 = call <vilib>:"Report Support Error.vi"("sim I/O info in"=w1404, "error in (no error)"=w1406) -> ("sim I/O info out"=w1403:T1, "error out"=w1405:errorcluster)  [unwired: 12 out]
            }
            frame "Read I/O" {
              n535 = global read "S2C_FPGA_InterfaceGlobals.vi" "C1/P1/B0"() -> (w1409:bool)
              n536 = To Variant(anything=w1409) -> (Variant=w1408:variant)
              n537 = Build Array(w1408) -> (w1407:variant[])
            }
            frame "Write I/O" {
              n538 = Index Array(array=w1417) -> (element=w1413:variant)  [unwired: 1 in]
              n539 = Variant To Data(error in=w1416, type=TRUE, Variant=w1413) -> (data=w1412:bool, error out=w1415:errorcluster)
              n540 = global write "S2C_FPGA_InterfaceGlobals.vi" "C1/P1/B0"(w1412) -> ()
            }
          }
        }
        frame "C1/P1/B1" {
          n541 = case "Node or Element Type Case Structure" shown="\"Read I/O\"" w1420 {
            tunnel: w1425 -> [w1430 w1435 w1440]
            tunnel: [w1429 w1435 w1439] -> w1424
            tunnel: w1423 -> [w1428 w1434 w1442]
            tunnel: [w1427 w1434 w1442] -> w1422
            tunnel: [variant[] [] w1431 _] -> w1421
            tunnel: w1419 -> [_ _ w1441]
            frame Default {
              # "5"
              n542 = call <vilib>:"Report Support Error.vi"("sim I/O info in"=w1428, "error in (no error)"=w1430) -> ("sim I/O info out"=w1427:T1, "error out"=w1429:errorcluster)  [unwired: 12 out]
            }
            frame "Read I/O" {
              n543 = global read "S2C_FPGA_InterfaceGlobals.vi" "C1/P1/B1"() -> (w1433:bool)
              n544 = To Variant(anything=w1433) -> (Variant=w1432:variant)
              n545 = Build Array(w1432) -> (w1431:variant[])
            }
            frame "Write I/O" {
              n546 = Index Array(array=w1441) -> (element=w1437:variant)  [unwired: 1 in]
              n547 = Variant To Data(error in=w1440, type=TRUE, Variant=w1437) -> (data=w1436:bool, error out=w1439:errorcluster)
              n548 = global write "S2C_FPGA_InterfaceGlobals.vi" "C1/P1/B1"(w1436) -> ()
            }
          }
        }
        frame "C1/P1/B2" {
          n549 = case "Node or Element Type Case Structure" shown="\"Read I/O\"" w1444 {
            tunnel: w1449 -> [w1454 w1459 w1464]
            tunnel: [w1453 w1459 w1463] -> w1448
            tunnel: w1447 -> [w1452 w1458 w1466]
            tunnel: [w1451 w1458 w1466] -> w1446
            tunnel: [variant[] [] w1455 _] -> w1445
            tunnel: w1443 -> [_ _ w1465]
            frame Default {
              # "5"
              n550 = call <vilib>:"Report Support Error.vi"("sim I/O info in"=w1452, "error in (no error)"=w1454) -> ("sim I/O info out"=w1451:T1, "error out"=w1453:errorcluster)  [unwired: 12 out]
            }
            frame "Read I/O" {
              n551 = global read "S2C_FPGA_InterfaceGlobals.vi" "C1/P1/B2"() -> (w1457:bool)
              n552 = To Variant(anything=w1457) -> (Variant=w1456:variant)
              n553 = Build Array(w1456) -> (w1455:variant[])
            }
            frame "Write I/O" {
              n554 = Index Array(array=w1465) -> (element=w1461:variant)  [unwired: 1 in]
              n555 = Variant To Data(error in=w1464, type=TRUE, Variant=w1461) -> (data=w1460:bool, error out=w1463:errorcluster)
              n556 = global write "S2C_FPGA_InterfaceGlobals.vi" "C1/P1/B2"(w1460) -> ()
            }
          }
        }
        frame "C1/P1/B3" {
          n557 = case "Node or Element Type Case Structure" shown="\"Read I/O\"" w1468 {
            tunnel: w1473 -> [w1478 w1483 w1488]
            tunnel: [w1477 w1483 w1487] -> w1472
            tunnel: w1471 -> [w1476 w1482 w1490]
            tunnel: [w1475 w1482 w1490] -> w1470
            tunnel: [variant[] [] w1479 _] -> w1469
            tunnel: w1467 -> [_ _ w1489]
            frame Default {
              # "5"
              n558 = call <vilib>:"Report Support Error.vi"("sim I/O info in"=w1476, "error in (no error)"=w1478) -> ("sim I/O info out"=w1475:T1, "error out"=w1477:errorcluster)  [unwired: 12 out]
            }
            frame "Read I/O" {
              n559 = global read "S2C_FPGA_InterfaceGlobals.vi" "C1/P1/B3"() -> (w1481:bool)
              n560 = To Variant(anything=w1481) -> (Variant=w1480:variant)
              n561 = Build Array(w1480) -> (w1479:variant[])
            }
            frame "Write I/O" {
              n562 = Index Array(array=w1489) -> (element=w1485:variant)  [unwired: 1 in]
              n563 = Variant To Data(error in=w1488, type=TRUE, Variant=w1485) -> (data=w1484:bool, error out=w1487:errorcluster)
              n564 = global write "S2C_FPGA_InterfaceGlobals.vi" "C1/P1/B3"(w1484) -> ()
            }
          }
        }
        frame "C1/P1/B4" {
          n565 = case "Node or Element Type Case Structure" shown="\"Read I/O\"" w1492 {
            tunnel: w1497 -> [w1502 w1507 w1512]
            tunnel: [w1501 w1507 w1511] -> w1496
            tunnel: w1495 -> [w1500 w1506 w1514]
            tunnel: [w1499 w1506 w1514] -> w1494
            tunnel: [variant[] [] w1503 _] -> w1493
            tunnel: w1491 -> [_ _ w1513]
            frame Default {
              # "5"
              n566 = call <vilib>:"Report Support Error.vi"("sim I/O info in"=w1500, "error in (no error)"=w1502) -> ("sim I/O info out"=w1499:T1, "error out"=w1501:errorcluster)  [unwired: 12 out]
            }
            frame "Read I/O" {
              n567 = global read "S2C_FPGA_InterfaceGlobals.vi" "C1/P1/B4"() -> (w1505:bool)
              n568 = To Variant(anything=w1505) -> (Variant=w1504:variant)
              n569 = Build Array(w1504) -> (w1503:variant[])
            }
            frame "Write I/O" {
              n570 = Index Array(array=w1513) -> (element=w1509:variant)  [unwired: 1 in]
              n571 = Variant To Data(error in=w1512, type=TRUE, Variant=w1509) -> (data=w1508:bool, error out=w1511:errorcluster)
              n572 = global write "S2C_FPGA_InterfaceGlobals.vi" "C1/P1/B4"(w1508) -> ()
            }
          }
        }
        frame "C1/P1/B5" {
          n573 = case "Node or Element Type Case Structure" shown="\"Read I/O\"" w1516 {
            tunnel: w1521 -> [w1526 w1531 w1536]
            tunnel: [w1525 w1531 w1535] -> w1520
            tunnel: w1519 -> [w1524 w1530 w1538]
            tunnel: [w1523 w1530 w1538] -> w1518
            tunnel: [variant[] [] w1527 _] -> w1517
            tunnel: w1515 -> [_ _ w1537]
            frame Default {
              # "5"
              n574 = call <vilib>:"Report Support Error.vi"("sim I/O info in"=w1524, "error in (no error)"=w1526) -> ("sim I/O info out"=w1523:T1, "error out"=w1525:errorcluster)  [unwired: 12 out]
            }
            frame "Read I/O" {
              n575 = global read "S2C_FPGA_InterfaceGlobals.vi" "C1/P1/B5"() -> (w1529:bool)
              n576 = To Variant(anything=w1529) -> (Variant=w1528:variant)
              n577 = Build Array(w1528) -> (w1527:variant[])
            }
            frame "Write I/O" {
              n578 = Index Array(array=w1537) -> (element=w1533:variant)  [unwired: 1 in]
              n579 = Variant To Data(error in=w1536, type=TRUE, Variant=w1533) -> (data=w1532:bool, error out=w1535:errorcluster)
              n580 = global write "S2C_FPGA_InterfaceGlobals.vi" "C1/P1/B5"(w1532) -> ()
            }
          }
        }
        frame "C1/P1/B6" {
          n581 = case "Node or Element Type Case Structure" shown="\"Read I/O\"" w1540 {
            tunnel: w1545 -> [w1550 w1555 w1560]
            tunnel: [w1549 w1555 w1559] -> w1544
            tunnel: w1543 -> [w1548 w1554 w1562]
            tunnel: [w1547 w1554 w1562] -> w1542
            tunnel: [variant[] [] w1551 _] -> w1541
            tunnel: w1539 -> [_ _ w1561]
            frame Default {
              # "5"
              n582 = call <vilib>:"Report Support Error.vi"("sim I/O info in"=w1548, "error in (no error)"=w1550) -> ("sim I/O info out"=w1547:T1, "error out"=w1549:errorcluster)  [unwired: 12 out]
            }
            frame "Read I/O" {
              n583 = global read "S2C_FPGA_InterfaceGlobals.vi" "C1/P1/B6"() -> (w1553:bool)
              n584 = To Variant(anything=w1553) -> (Variant=w1552:variant)
              n585 = Build Array(w1552) -> (w1551:variant[])
            }
            frame "Write I/O" {
              n586 = Index Array(array=w1561) -> (element=w1557:variant)  [unwired: 1 in]
              n587 = Variant To Data(error in=w1560, type=TRUE, Variant=w1557) -> (data=w1556:bool, error out=w1559:errorcluster)
              n588 = global write "S2C_FPGA_InterfaceGlobals.vi" "C1/P1/B6"(w1556) -> ()
            }
          }
        }
        frame "C1/P1/B7" {
          n589 = case "Node or Element Type Case Structure" shown="\"Read I/O\"" w1564 {
            tunnel: w1569 -> [w1574 w1579 w1584]
            tunnel: [w1573 w1579 w1583] -> w1568
            tunnel: w1567 -> [w1572 w1578 w1586]
            tunnel: [w1571 w1578 w1586] -> w1566
            tunnel: [variant[] [] w1575 _] -> w1565
            tunnel: w1563 -> [_ _ w1585]
            frame Default {
              # "5"
              n590 = call <vilib>:"Report Support Error.vi"("sim I/O info in"=w1572, "error in (no error)"=w1574) -> ("sim I/O info out"=w1571:T1, "error out"=w1573:errorcluster)  [unwired: 12 out]
            }
            frame "Read I/O" {
              n591 = global read "S2C_FPGA_InterfaceGlobals.vi" "C1/P1/B7"() -> (w1577:bool)
              n592 = To Variant(anything=w1577) -> (Variant=w1576:variant)
              n593 = Build Array(w1576) -> (w1575:variant[])
            }
            frame "Write I/O" {
              n594 = Index Array(array=w1585) -> (element=w1581:variant)  [unwired: 1 in]
              n595 = Variant To Data(error in=w1584, type=TRUE, Variant=w1581) -> (data=w1580:bool, error out=w1583:errorcluster)
              n596 = global write "S2C_FPGA_InterfaceGlobals.vi" "C1/P1/B7"(w1580) -> ()
            }
          }
        }
        frame "C1/P2/B0" {
          n597 = case "Node or Element Type Case Structure" shown="\"Read I/O\"" w1588 {
            tunnel: w1593 -> [w1598 w1603 w1608]
            tunnel: [w1597 w1603 w1607] -> w1592
            tunnel: w1591 -> [w1596 w1602 w1610]
            tunnel: [w1595 w1602 w1610] -> w1590
            tunnel: [variant[] [] w1599 _] -> w1589
            tunnel: w1587 -> [_ _ w1609]
            frame Default {
              # "5"
              n598 = call <vilib>:"Report Support Error.vi"("sim I/O info in"=w1596, "error in (no error)"=w1598) -> ("sim I/O info out"=w1595:T1, "error out"=w1597:errorcluster)  [unwired: 12 out]
            }
            frame "Read I/O" {
              n599 = global read "S2C_FPGA_InterfaceGlobals.vi" "C1/P2/B0"() -> (w1601:bool)
              n600 = To Variant(anything=w1601) -> (Variant=w1600:variant)
              n601 = Build Array(w1600) -> (w1599:variant[])
            }
            frame "Write I/O" {
              n602 = Index Array(array=w1609) -> (element=w1605:variant)  [unwired: 1 in]
              n603 = Variant To Data(error in=w1608, type=TRUE, Variant=w1605) -> (data=w1604:bool, error out=w1607:errorcluster)
              n604 = global write "S2C_FPGA_InterfaceGlobals.vi" "C1/P2/B0"(w1604) -> ()
            }
          }
        }
        frame "C1/P2/B1" {
          n605 = case "Node or Element Type Case Structure" shown="\"Read I/O\"" w1612 {
            tunnel: w1617 -> [w1622 w1627 w1632]
            tunnel: [w1621 w1627 w1631] -> w1616
            tunnel: w1615 -> [w1620 w1626 w1634]
            tunnel: [w1619 w1626 w1634] -> w1614
            tunnel: [variant[] [] w1623 _] -> w1613
            tunnel: w1611 -> [_ _ w1633]
            frame Default {
              # "5"
              n606 = call <vilib>:"Report Support Error.vi"("sim I/O info in"=w1620, "error in (no error)"=w1622) -> ("sim I/O info out"=w1619:T1, "error out"=w1621:errorcluster)  [unwired: 12 out]
            }
            frame "Read I/O" {
              n607 = global read "S2C_FPGA_InterfaceGlobals.vi" "C1/P2/B1"() -> (w1625:bool)
              n608 = To Variant(anything=w1625) -> (Variant=w1624:variant)
              n609 = Build Array(w1624) -> (w1623:variant[])
            }
            frame "Write I/O" {
              n610 = Index Array(array=w1633) -> (element=w1629:variant)  [unwired: 1 in]
              n611 = Variant To Data(error in=w1632, type=TRUE, Variant=w1629) -> (data=w1628:bool, error out=w1631:errorcluster)
              n612 = global write "S2C_FPGA_InterfaceGlobals.vi" "C1/P2/B1"(w1628) -> ()
            }
          }
        }
        frame "C1/P2/B2" {
          n613 = case "Node or Element Type Case Structure" shown="\"Read I/O\"" w1636 {
            tunnel: w1641 -> [w1646 w1651 w1656]
            tunnel: [w1645 w1651 w1655] -> w1640
            tunnel: w1639 -> [w1644 w1650 w1658]
            tunnel: [w1643 w1650 w1658] -> w1638
            tunnel: [variant[] [] w1647 _] -> w1637
            tunnel: w1635 -> [_ _ w1657]
            frame Default {
              # "5"
              n614 = call <vilib>:"Report Support Error.vi"("sim I/O info in"=w1644, "error in (no error)"=w1646) -> ("sim I/O info out"=w1643:T1, "error out"=w1645:errorcluster)  [unwired: 12 out]
            }
            frame "Read I/O" {
              n615 = global read "S2C_FPGA_InterfaceGlobals.vi" "C1/P2/B2"() -> (w1649:bool)
              n616 = To Variant(anything=w1649) -> (Variant=w1648:variant)
              n617 = Build Array(w1648) -> (w1647:variant[])
            }
            frame "Write I/O" {
              n618 = Index Array(array=w1657) -> (element=w1653:variant)  [unwired: 1 in]
              n619 = Variant To Data(error in=w1656, type=TRUE, Variant=w1653) -> (data=w1652:bool, error out=w1655:errorcluster)
              n620 = global write "S2C_FPGA_InterfaceGlobals.vi" "C1/P2/B2"(w1652) -> ()
            }
          }
        }
        frame "C1/P2/B3" {
          n621 = case "Node or Element Type Case Structure" shown="\"Read I/O\"" w1660 {
            tunnel: w1665 -> [w1670 w1675 w1680]
            tunnel: [w1669 w1675 w1679] -> w1664
            tunnel: w1663 -> [w1668 w1674 w1682]
            tunnel: [w1667 w1674 w1682] -> w1662
            tunnel: [variant[] [] w1671 _] -> w1661
            tunnel: w1659 -> [_ _ w1681]
            frame Default {
              # "5"
              n622 = call <vilib>:"Report Support Error.vi"("sim I/O info in"=w1668, "error in (no error)"=w1670) -> ("sim I/O info out"=w1667:T1, "error out"=w1669:errorcluster)  [unwired: 12 out]
            }
            frame "Read I/O" {
              n623 = global read "S2C_FPGA_InterfaceGlobals.vi" "C1/P2/B3"() -> (w1673:bool)
              n624 = To Variant(anything=w1673) -> (Variant=w1672:variant)
              n625 = Build Array(w1672) -> (w1671:variant[])
            }
            frame "Write I/O" {
              n626 = Index Array(array=w1681) -> (element=w1677:variant)  [unwired: 1 in]
              n627 = Variant To Data(error in=w1680, type=TRUE, Variant=w1677) -> (data=w1676:bool, error out=w1679:errorcluster)
              n628 = global write "S2C_FPGA_InterfaceGlobals.vi" "C1/P2/B3"(w1676) -> ()
            }
          }
        }
        frame "C1/P2/B4" {
          n629 = case "Node or Element Type Case Structure" shown="\"Read I/O\"" w1684 {
            tunnel: w1689 -> [w1694 w1699 w1704]
            tunnel: [w1693 w1699 w1703] -> w1688
            tunnel: w1687 -> [w1692 w1698 w1706]
            tunnel: [w1691 w1698 w1706] -> w1686
            tunnel: [variant[] [] w1695 _] -> w1685
            tunnel: w1683 -> [_ _ w1705]
            frame Default {
              # "5"
              n630 = call <vilib>:"Report Support Error.vi"("sim I/O info in"=w1692, "error in (no error)"=w1694) -> ("sim I/O info out"=w1691:T1, "error out"=w1693:errorcluster)  [unwired: 12 out]
            }
            frame "Read I/O" {
              n631 = global read "S2C_FPGA_InterfaceGlobals.vi" "C1/P2/B4"() -> (w1697:bool)
              n632 = To Variant(anything=w1697) -> (Variant=w1696:variant)
              n633 = Build Array(w1696) -> (w1695:variant[])
            }
            frame "Write I/O" {
              n634 = Index Array(array=w1705) -> (element=w1701:variant)  [unwired: 1 in]
              n635 = Variant To Data(error in=w1704, type=TRUE, Variant=w1701) -> (data=w1700:bool, error out=w1703:errorcluster)
              n636 = global write "S2C_FPGA_InterfaceGlobals.vi" "C1/P2/B4"(w1700) -> ()
            }
          }
        }
        frame "C1/P2/B5" {
          n637 = case "Node or Element Type Case Structure" shown="\"Read I/O\"" w1708 {
            tunnel: w1713 -> [w1718 w1723 w1728]
            tunnel: [w1717 w1723 w1727] -> w1712
            tunnel: w1711 -> [w1716 w1722 w1730]
            tunnel: [w1715 w1722 w1730] -> w1710
            tunnel: [variant[] [] w1719 _] -> w1709
            tunnel: w1707 -> [_ _ w1729]
            frame Default {
              # "5"
              n638 = call <vilib>:"Report Support Error.vi"("sim I/O info in"=w1716, "error in (no error)"=w1718) -> ("sim I/O info out"=w1715:T1, "error out"=w1717:errorcluster)  [unwired: 12 out]
            }
            frame "Read I/O" {
              n639 = global read "S2C_FPGA_InterfaceGlobals.vi" "C1/P2/B5"() -> (w1721:bool)
              n640 = To Variant(anything=w1721) -> (Variant=w1720:variant)
              n641 = Build Array(w1720) -> (w1719:variant[])
            }
            frame "Write I/O" {
              n642 = Index Array(array=w1729) -> (element=w1725:variant)  [unwired: 1 in]
              n643 = Variant To Data(error in=w1728, type=TRUE, Variant=w1725) -> (data=w1724:bool, error out=w1727:errorcluster)
              n644 = global write "S2C_FPGA_InterfaceGlobals.vi" "C1/P2/B5"(w1724) -> ()
            }
          }
        }
        frame "C1/P2/B6" {
          n645 = case "Node or Element Type Case Structure" shown="\"Read I/O\"" w1732 {
            tunnel: w1737 -> [w1742 w1747 w1752]
            tunnel: [w1741 w1747 w1751] -> w1736
            tunnel: w1735 -> [w1740 w1746 w1754]
            tunnel: [w1739 w1746 w1754] -> w1734
            tunnel: [variant[] [] w1743 _] -> w1733
            tunnel: w1731 -> [_ _ w1753]
            frame Default {
              # "5"
              n646 = call <vilib>:"Report Support Error.vi"("sim I/O info in"=w1740, "error in (no error)"=w1742) -> ("sim I/O info out"=w1739:T1, "error out"=w1741:errorcluster)  [unwired: 12 out]
            }
            frame "Read I/O" {
              n647 = global read "S2C_FPGA_InterfaceGlobals.vi" "C1/P2/B6"() -> (w1745:bool)
              n648 = To Variant(anything=w1745) -> (Variant=w1744:variant)
              n649 = Build Array(w1744) -> (w1743:variant[])
            }
            frame "Write I/O" {
              n650 = Index Array(array=w1753) -> (element=w1749:variant)  [unwired: 1 in]
              n651 = Variant To Data(error in=w1752, type=TRUE, Variant=w1749) -> (data=w1748:bool, error out=w1751:errorcluster)
              n652 = global write "S2C_FPGA_InterfaceGlobals.vi" "C1/P2/B6"(w1748) -> ()
            }
          }
        }
        frame "C1/P2/B7" {
          n653 = case "Node or Element Type Case Structure" shown="\"Write I/O\"" w1756 {
            tunnel: w1761 -> [w1766 w1771 w1776]
            tunnel: [w1765 w1771 w1775] -> w1760
            tunnel: w1759 -> [w1764 w1770 w1778]
            tunnel: [w1763 w1770 w1778] -> w1758
            tunnel: [variant[] [] w1767 _] -> w1757
            tunnel: w1755 -> [_ _ w1777]
            frame Default {
              # "5"
              n654 = call <vilib>:"Report Support Error.vi"("sim I/O info in"=w1764, "error in (no error)"=w1766) -> ("sim I/O info out"=w1763:T1, "error out"=w1765:errorcluster)  [unwired: 12 out]
            }
            frame "Read I/O" {
              n655 = global read "S2C_FPGA_InterfaceGlobals.vi" "C1/P2/B7"() -> (w1769:bool)
              n656 = To Variant(anything=w1769) -> (Variant=w1768:variant)
              n657 = Build Array(w1768) -> (w1767:variant[])
            }
            frame "Write I/O" {
              n658 = Index Array(array=w1777) -> (element=w1773:variant)  [unwired: 1 in]
              n659 = Variant To Data(error in=w1776, type=TRUE, Variant=w1773) -> (data=w1772:bool, error out=w1775:errorcluster)
              n660 = global write "S2C_FPGA_InterfaceGlobals.vi" "C1/P2/B7"(w1772) -> ()
            }
          }
        }
        frame "C1/P3/B0" {
          n661 = case "Node or Element Type Case Structure" shown="\"Read I/O\"" w1780 {
            tunnel: w1785 -> [w1790 w1795 w1800]
            tunnel: [w1789 w1795 w1799] -> w1784
            tunnel: w1783 -> [w1788 w1794 w1802]
            tunnel: [w1787 w1794 w1802] -> w1782
            tunnel: [variant[] [] w1791 _] -> w1781
            tunnel: w1779 -> [_ _ w1801]
            frame Default {
              # "5"
              n662 = call <vilib>:"Report Support Error.vi"("sim I/O info in"=w1788, "error in (no error)"=w1790) -> ("sim I/O info out"=w1787:T1, "error out"=w1789:errorcluster)  [unwired: 12 out]
            }
            frame "Read I/O" {
              n663 = global read "S2C_FPGA_InterfaceGlobals.vi" "C1/P3/B0"() -> (w1793:bool)
              n664 = To Variant(anything=w1793) -> (Variant=w1792:variant)
              n665 = Build Array(w1792) -> (w1791:variant[])
            }
            frame "Write I/O" {
              n666 = Index Array(array=w1801) -> (element=w1797:variant)  [unwired: 1 in]
              n667 = Variant To Data(error in=w1800, type=TRUE, Variant=w1797) -> (data=w1796:bool, error out=w1799:errorcluster)
              n668 = global write "S2C_FPGA_InterfaceGlobals.vi" "C1/P3/B0"(w1796) -> ()
            }
          }
        }
        frame "C1/P3/B1" {
          n669 = case "Node or Element Type Case Structure" shown="\"Read I/O\"" w1804 {
            tunnel: w1809 -> [w1814 w1819 w1824]
            tunnel: [w1813 w1819 w1823] -> w1808
            tunnel: w1807 -> [w1812 w1818 w1826]
            tunnel: [w1811 w1818 w1826] -> w1806
            tunnel: [variant[] [] w1815 _] -> w1805
            tunnel: w1803 -> [_ _ w1825]
            frame Default {
              # "5"
              n670 = call <vilib>:"Report Support Error.vi"("sim I/O info in"=w1812, "error in (no error)"=w1814) -> ("sim I/O info out"=w1811:T1, "error out"=w1813:errorcluster)  [unwired: 12 out]
            }
            frame "Read I/O" {
              n671 = global read "S2C_FPGA_InterfaceGlobals.vi" "C1/P3/B1"() -> (w1817:bool)
              n672 = To Variant(anything=w1817) -> (Variant=w1816:variant)
              n673 = Build Array(w1816) -> (w1815:variant[])
            }
            frame "Write I/O" {
              n674 = Index Array(array=w1825) -> (element=w1821:variant)  [unwired: 1 in]
              n675 = Variant To Data(error in=w1824, type=TRUE, Variant=w1821) -> (data=w1820:bool, error out=w1823:errorcluster)
              n676 = global write "S2C_FPGA_InterfaceGlobals.vi" "C1/P3/B1"(w1820) -> ()
            }
          }
        }
        frame "C1/P3/B2" {
          n677 = case "Node or Element Type Case Structure" shown="\"Read I/O\"" w1828 {
            tunnel: w1833 -> [w1838 w1843 w1848]
            tunnel: [w1837 w1843 w1847] -> w1832
            tunnel: w1831 -> [w1836 w1842 w1850]
            tunnel: [w1835 w1842 w1850] -> w1830
            tunnel: [variant[] [] w1839 _] -> w1829
            tunnel: w1827 -> [_ _ w1849]
            frame Default {
              # "5"
              n678 = call <vilib>:"Report Support Error.vi"("sim I/O info in"=w1836, "error in (no error)"=w1838) -> ("sim I/O info out"=w1835:T1, "error out"=w1837:errorcluster)  [unwired: 12 out]
            }
            frame "Read I/O" {
              n679 = global read "S2C_FPGA_InterfaceGlobals.vi" "C1/P3/B2"() -> (w1841:bool)
              n680 = To Variant(anything=w1841) -> (Variant=w1840:variant)
              n681 = Build Array(w1840) -> (w1839:variant[])
            }
            frame "Write I/O" {
              n682 = Index Array(array=w1849) -> (element=w1845:variant)  [unwired: 1 in]
              n683 = Variant To Data(error in=w1848, type=TRUE, Variant=w1845) -> (data=w1844:bool, error out=w1847:errorcluster)
              n684 = global write "S2C_FPGA_InterfaceGlobals.vi" "C1/P3/B2"(w1844) -> ()
            }
          }
        }
        frame "C1/P3/B3" {
          n685 = case "Node or Element Type Case Structure" shown="\"Read I/O\"" w1852 {
            tunnel: w1857 -> [w1862 w1867 w1872]
            tunnel: [w1861 w1867 w1871] -> w1856
            tunnel: w1855 -> [w1860 w1866 w1874]
            tunnel: [w1859 w1866 w1874] -> w1854
            tunnel: [variant[] [] w1863 _] -> w1853
            tunnel: w1851 -> [_ _ w1873]
            frame Default {
              # "5"
              n686 = call <vilib>:"Report Support Error.vi"("sim I/O info in"=w1860, "error in (no error)"=w1862) -> ("sim I/O info out"=w1859:T1, "error out"=w1861:errorcluster)  [unwired: 12 out]
            }
            frame "Read I/O" {
              n687 = global read "S2C_FPGA_InterfaceGlobals.vi" "C1/P3/B3"() -> (w1865:bool)
              n688 = To Variant(anything=w1865) -> (Variant=w1864:variant)
              n689 = Build Array(w1864) -> (w1863:variant[])
            }
            frame "Write I/O" {
              n690 = Index Array(array=w1873) -> (element=w1869:variant)  [unwired: 1 in]
              n691 = Variant To Data(error in=w1872, type=TRUE, Variant=w1869) -> (data=w1868:bool, error out=w1871:errorcluster)
              n692 = global write "S2C_FPGA_InterfaceGlobals.vi" "C1/P3/B3"(w1868) -> ()
            }
          }
        }
        frame "C1/P3/B4" {
          n693 = case "Node or Element Type Case Structure" shown="\"Read I/O\"" w1876 {
            tunnel: w1881 -> [w1886 w1891 w1896]
            tunnel: [w1885 w1891 w1895] -> w1880
            tunnel: w1879 -> [w1884 w1890 w1898]
            tunnel: [w1883 w1890 w1898] -> w1878
            tunnel: [variant[] [] w1887 _] -> w1877
            tunnel: w1875 -> [_ _ w1897]
            frame Default {
              # "5"
              n694 = call <vilib>:"Report Support Error.vi"("sim I/O info in"=w1884, "error in (no error)"=w1886) -> ("sim I/O info out"=w1883:T1, "error out"=w1885:errorcluster)  [unwired: 12 out]
            }
            frame "Read I/O" {
              n695 = global read "S2C_FPGA_InterfaceGlobals.vi" "C1/P3/B4"() -> (w1889:bool)
              n696 = To Variant(anything=w1889) -> (Variant=w1888:variant)
              n697 = Build Array(w1888) -> (w1887:variant[])
            }
            frame "Write I/O" {
              n698 = Index Array(array=w1897) -> (element=w1893:variant)  [unwired: 1 in]
              n699 = Variant To Data(error in=w1896, type=TRUE, Variant=w1893) -> (data=w1892:bool, error out=w1895:errorcluster)
              n700 = global write "S2C_FPGA_InterfaceGlobals.vi" "C1/P3/B4"(w1892) -> ()
            }
          }
        }
        frame "C1/P3/B5" {
          n701 = case "Node or Element Type Case Structure" shown="\"Read I/O\"" w1900 {
            tunnel: w1905 -> [w1910 w1915 w1920]
            tunnel: [w1909 w1915 w1919] -> w1904
            tunnel: w1903 -> [w1908 w1914 w1922]
            tunnel: [w1907 w1914 w1922] -> w1902
            tunnel: [variant[] [] w1911 _] -> w1901
            tunnel: w1899 -> [_ _ w1921]
            frame Default {
              # "5"
              n702 = call <vilib>:"Report Support Error.vi"("sim I/O info in"=w1908, "error in (no error)"=w1910) -> ("sim I/O info out"=w1907:T1, "error out"=w1909:errorcluster)  [unwired: 12 out]
            }
            frame "Read I/O" {
              n703 = global read "S2C_FPGA_InterfaceGlobals.vi" "C1/P3/B5"() -> (w1913:bool)
              n704 = To Variant(anything=w1913) -> (Variant=w1912:variant)
              n705 = Build Array(w1912) -> (w1911:variant[])
            }
            frame "Write I/O" {
              n706 = Index Array(array=w1921) -> (element=w1917:variant)  [unwired: 1 in]
              n707 = Variant To Data(error in=w1920, type=TRUE, Variant=w1917) -> (data=w1916:bool, error out=w1919:errorcluster)
              n708 = global write "S2C_FPGA_InterfaceGlobals.vi" "C1/P3/B5"(w1916) -> ()
            }
          }
        }
        frame "C1/P3/B6" {
          n709 = case "Node or Element Type Case Structure" shown="\"Read I/O\"" w1924 {
            tunnel: w1929 -> [w1934 w1939 w1944]
            tunnel: [w1933 w1939 w1943] -> w1928
            tunnel: w1927 -> [w1932 w1938 w1946]
            tunnel: [w1931 w1938 w1946] -> w1926
            tunnel: [variant[] [] w1935 _] -> w1925
            tunnel: w1923 -> [_ _ w1945]
            frame Default {
              # "5"
              n710 = call <vilib>:"Report Support Error.vi"("sim I/O info in"=w1932, "error in (no error)"=w1934) -> ("sim I/O info out"=w1931:T1, "error out"=w1933:errorcluster)  [unwired: 12 out]
            }
            frame "Read I/O" {
              n711 = global read "S2C_FPGA_InterfaceGlobals.vi" "C1/P3/B6"() -> (w1937:bool)
              n712 = To Variant(anything=w1937) -> (Variant=w1936:variant)
              n713 = Build Array(w1936) -> (w1935:variant[])
            }
            frame "Write I/O" {
              n714 = Index Array(array=w1945) -> (element=w1941:variant)  [unwired: 1 in]
              n715 = Variant To Data(error in=w1944, type=TRUE, Variant=w1941) -> (data=w1940:bool, error out=w1943:errorcluster)
              n716 = global write "S2C_FPGA_InterfaceGlobals.vi" "C1/P3/B6"(w1940) -> ()
            }
          }
        }
        frame "C1/P3/B7" {
          n717 = case "Node or Element Type Case Structure" shown="\"Read I/O\"" w1948 {
            tunnel: w1953 -> [w1958 w1963 w1968]
            tunnel: [w1957 w1963 w1967] -> w1952
            tunnel: w1951 -> [w1956 w1962 w1970]
            tunnel: [w1955 w1962 w1970] -> w1950
            tunnel: [variant[] [] w1959 _] -> w1949
            tunnel: w1947 -> [_ _ w1969]
            frame Default {
              # "5"
              n718 = call <vilib>:"Report Support Error.vi"("sim I/O info in"=w1956, "error in (no error)"=w1958) -> ("sim I/O info out"=w1955:T1, "error out"=w1957:errorcluster)  [unwired: 12 out]
            }
            frame "Read I/O" {
              n719 = global read "S2C_FPGA_InterfaceGlobals.vi" "C1/P3/B7"() -> (w1961:bool)
              n720 = To Variant(anything=w1961) -> (Variant=w1960:variant)
              n721 = Build Array(w1960) -> (w1959:variant[])
            }
            frame "Write I/O" {
              n722 = Index Array(array=w1969) -> (element=w1965:variant)  [unwired: 1 in]
              n723 = Variant To Data(error in=w1968, type=TRUE, Variant=w1965) -> (data=w1964:bool, error out=w1967:errorcluster)
              n724 = global write "S2C_FPGA_InterfaceGlobals.vi" "C1/P3/B7"(w1964) -> ()
            }
          }
        }
        frame "C1/P4/B0" {
          n725 = case "Node or Element Type Case Structure" shown="\"Read I/O\"" w1972 {
            tunnel: w1977 -> [w1982 w1987 w1992]
            tunnel: [w1981 w1987 w1991] -> w1976
            tunnel: w1975 -> [w1980 w1986 w1994]
            tunnel: [w1979 w1986 w1994] -> w1974
            tunnel: [variant[] [] w1983 _] -> w1973
            tunnel: w1971 -> [_ _ w1993]
            frame Default {
              # "5"
              n726 = call <vilib>:"Report Support Error.vi"("sim I/O info in"=w1980, "error in (no error)"=w1982) -> ("sim I/O info out"=w1979:T1, "error out"=w1981:errorcluster)  [unwired: 12 out]
            }
            frame "Read I/O" {
              n727 = global read "S2C_FPGA_InterfaceGlobals.vi" "C1/P4/B0"() -> (w1985:bool)
              n728 = To Variant(anything=w1985) -> (Variant=w1984:variant)
              n729 = Build Array(w1984) -> (w1983:variant[])
            }
            frame "Write I/O" {
              n730 = Index Array(array=w1993) -> (element=w1989:variant)  [unwired: 1 in]
              n731 = Variant To Data(error in=w1992, type=TRUE, Variant=w1989) -> (data=w1988:bool, error out=w1991:errorcluster)
              n732 = global write "S2C_FPGA_InterfaceGlobals.vi" "C1/P4/B0"(w1988) -> ()
            }
          }
        }
        frame "C1/P4/B1" {
          n733 = case "Node or Element Type Case Structure" shown="\"Read I/O\"" w1996 {
            tunnel: w2001 -> [w2006 w2011 w2016]
            tunnel: [w2005 w2011 w2015] -> w2000
            tunnel: w1999 -> [w2004 w2010 w2018]
            tunnel: [w2003 w2010 w2018] -> w1998
            tunnel: [variant[] [] w2007 _] -> w1997
            tunnel: w1995 -> [_ _ w2017]
            frame Default {
              # "5"
              n734 = call <vilib>:"Report Support Error.vi"("sim I/O info in"=w2004, "error in (no error)"=w2006) -> ("sim I/O info out"=w2003:T1, "error out"=w2005:errorcluster)  [unwired: 12 out]
            }
            frame "Read I/O" {
              n735 = global read "S2C_FPGA_InterfaceGlobals.vi" "C1/P4/B1"() -> (w2009:bool)
              n736 = To Variant(anything=w2009) -> (Variant=w2008:variant)
              n737 = Build Array(w2008) -> (w2007:variant[])
            }
            frame "Write I/O" {
              n738 = Index Array(array=w2017) -> (element=w2013:variant)  [unwired: 1 in]
              n739 = Variant To Data(error in=w2016, type=TRUE, Variant=w2013) -> (data=w2012:bool, error out=w2015:errorcluster)
              n740 = global write "S2C_FPGA_InterfaceGlobals.vi" "C1/P4/B1"(w2012) -> ()
            }
          }
        }
        frame "C1/P4/B2" {
          n741 = case "Node or Element Type Case Structure" shown="\"Read I/O\"" w2020 {
            tunnel: w2025 -> [w2030 w2035 w2040]
            tunnel: [w2029 w2035 w2039] -> w2024
            tunnel: w2023 -> [w2028 w2034 w2042]
            tunnel: [w2027 w2034 w2042] -> w2022
            tunnel: [variant[] [] w2031 _] -> w2021
            tunnel: w2019 -> [_ _ w2041]
            frame Default {
              # "5"
              n742 = call <vilib>:"Report Support Error.vi"("sim I/O info in"=w2028, "error in (no error)"=w2030) -> ("sim I/O info out"=w2027:T1, "error out"=w2029:errorcluster)  [unwired: 12 out]
            }
            frame "Read I/O" {
              n743 = global read "S2C_FPGA_InterfaceGlobals.vi" "C1/P4/B2"() -> (w2033:bool)
              n744 = To Variant(anything=w2033) -> (Variant=w2032:variant)
              n745 = Build Array(w2032) -> (w2031:variant[])
            }
            frame "Write I/O" {
              n746 = Index Array(array=w2041) -> (element=w2037:variant)  [unwired: 1 in]
              n747 = Variant To Data(error in=w2040, type=TRUE, Variant=w2037) -> (data=w2036:bool, error out=w2039:errorcluster)
              n748 = global write "S2C_FPGA_InterfaceGlobals.vi" "C1/P4/B2"(w2036) -> ()
            }
          }
        }
        frame "C1/P4/B3" {
          n749 = case "Node or Element Type Case Structure" shown="\"Read I/O\"" w2044 {
            tunnel: w2049 -> [w2054 w2059 w2064]
            tunnel: [w2053 w2059 w2063] -> w2048
            tunnel: w2047 -> [w2052 w2058 w2066]
            tunnel: [w2051 w2058 w2066] -> w2046
            tunnel: [variant[] [] w2055 _] -> w2045
            tunnel: w2043 -> [_ _ w2065]
            frame Default {
              # "5"
              n750 = call <vilib>:"Report Support Error.vi"("sim I/O info in"=w2052, "error in (no error)"=w2054) -> ("sim I/O info out"=w2051:T1, "error out"=w2053:errorcluster)  [unwired: 12 out]
            }
            frame "Read I/O" {
              n751 = global read "S2C_FPGA_InterfaceGlobals.vi" "C1/P4/B3"() -> (w2057:bool)
              n752 = To Variant(anything=w2057) -> (Variant=w2056:variant)
              n753 = Build Array(w2056) -> (w2055:variant[])
            }
            frame "Write I/O" {
              n754 = Index Array(array=w2065) -> (element=w2061:variant)  [unwired: 1 in]
              n755 = Variant To Data(error in=w2064, type=TRUE, Variant=w2061) -> (data=w2060:bool, error out=w2063:errorcluster)
              n756 = global write "S2C_FPGA_InterfaceGlobals.vi" "C1/P4/B3"(w2060) -> ()
            }
          }
        }
        frame "C1/P4/B4" {
          n757 = case "Node or Element Type Case Structure" shown="\"Read I/O\"" w2068 {
            tunnel: w2073 -> [w2078 w2083 w2088]
            tunnel: [w2077 w2083 w2087] -> w2072
            tunnel: w2071 -> [w2076 w2082 w2090]
            tunnel: [w2075 w2082 w2090] -> w2070
            tunnel: [variant[] [] w2079 _] -> w2069
            tunnel: w2067 -> [_ _ w2089]
            frame Default {
              # "5"
              n758 = call <vilib>:"Report Support Error.vi"("sim I/O info in"=w2076, "error in (no error)"=w2078) -> ("sim I/O info out"=w2075:T1, "error out"=w2077:errorcluster)  [unwired: 12 out]
            }
            frame "Read I/O" {
              n759 = global read "S2C_FPGA_InterfaceGlobals.vi" "C1/P4/B4"() -> (w2081:bool)
              n760 = To Variant(anything=w2081) -> (Variant=w2080:variant)
              n761 = Build Array(w2080) -> (w2079:variant[])
            }
            frame "Write I/O" {
              n762 = Index Array(array=w2089) -> (element=w2085:variant)  [unwired: 1 in]
              n763 = Variant To Data(error in=w2088, type=TRUE, Variant=w2085) -> (data=w2084:bool, error out=w2087:errorcluster)
              n764 = global write "S2C_FPGA_InterfaceGlobals.vi" "C1/P4/B4"(w2084) -> ()
            }
          }
        }
        frame "C1/P4/B5" {
          n765 = case "Node or Element Type Case Structure" shown="\"Read I/O\"" w2092 {
            tunnel: w2097 -> [w2102 w2107 w2112]
            tunnel: [w2101 w2107 w2111] -> w2096
            tunnel: w2095 -> [w2100 w2106 w2114]
            tunnel: [w2099 w2106 w2114] -> w2094
            tunnel: [variant[] [] w2103 _] -> w2093
            tunnel: w2091 -> [_ _ w2113]
            frame Default {
              # "5"
              n766 = call <vilib>:"Report Support Error.vi"("sim I/O info in"=w2100, "error in (no error)"=w2102) -> ("sim I/O info out"=w2099:T1, "error out"=w2101:errorcluster)  [unwired: 12 out]
            }
            frame "Read I/O" {
              n767 = global read "S2C_FPGA_InterfaceGlobals.vi" "C1/P4/B5"() -> (w2105:bool)
              n768 = To Variant(anything=w2105) -> (Variant=w2104:variant)
              n769 = Build Array(w2104) -> (w2103:variant[])
            }
            frame "Write I/O" {
              n770 = Index Array(array=w2113) -> (element=w2109:variant)  [unwired: 1 in]
              n771 = Variant To Data(error in=w2112, type=TRUE, Variant=w2109) -> (data=w2108:bool, error out=w2111:errorcluster)
              n772 = global write "S2C_FPGA_InterfaceGlobals.vi" "C1/P4/B5"(w2108) -> ()
            }
          }
        }
        frame "C1/P4/B6" {
          n773 = case "Node or Element Type Case Structure" shown="\"Read I/O\"" w2116 {
            tunnel: w2121 -> [w2126 w2131 w2136]
            tunnel: [w2125 w2131 w2135] -> w2120
            tunnel: w2119 -> [w2124 w2130 w2138]
            tunnel: [w2123 w2130 w2138] -> w2118
            tunnel: [variant[] [] w2127 _] -> w2117
            tunnel: w2115 -> [_ _ w2137]
            frame Default {
              # "5"
              n774 = call <vilib>:"Report Support Error.vi"("sim I/O info in"=w2124, "error in (no error)"=w2126) -> ("sim I/O info out"=w2123:T1, "error out"=w2125:errorcluster)  [unwired: 12 out]
            }
            frame "Read I/O" {
              n775 = global read "S2C_FPGA_InterfaceGlobals.vi" "C1/P4/B6"() -> (w2129:bool)
              n776 = To Variant(anything=w2129) -> (Variant=w2128:variant)
              n777 = Build Array(w2128) -> (w2127:variant[])
            }
            frame "Write I/O" {
              n778 = Index Array(array=w2137) -> (element=w2133:variant)  [unwired: 1 in]
              n779 = Variant To Data(error in=w2136, type=TRUE, Variant=w2133) -> (data=w2132:bool, error out=w2135:errorcluster)
              n780 = global write "S2C_FPGA_InterfaceGlobals.vi" "C1/P4/B6"(w2132) -> ()
            }
          }
        }
        frame "C1/P4/B7" {
          n781 = case "Node or Element Type Case Structure" shown="\"Write I/O\"" w2140 {
            tunnel: w2145 -> [w2150 w2155 w2160]
            tunnel: [w2149 w2155 w2159] -> w2144
            tunnel: w2143 -> [w2148 w2154 w2162]
            tunnel: [w2147 w2154 w2162] -> w2142
            tunnel: [variant[] [] w2151 _] -> w2141
            tunnel: w2139 -> [_ _ w2161]
            frame Default {
              # "5"
              n782 = call <vilib>:"Report Support Error.vi"("sim I/O info in"=w2148, "error in (no error)"=w2150) -> ("sim I/O info out"=w2147:T1, "error out"=w2149:errorcluster)  [unwired: 12 out]
            }
            frame "Read I/O" {
              n783 = global read "S2C_FPGA_InterfaceGlobals.vi" "C1/P4/B7"() -> (w2153:bool)
              n784 = To Variant(anything=w2153) -> (Variant=w2152:variant)
              n785 = Build Array(w2152) -> (w2151:variant[])
            }
            frame "Write I/O" {
              n786 = Index Array(array=w2161) -> (element=w2157:variant)  [unwired: 1 in]
              n787 = Variant To Data(error in=w2160, type=TRUE, Variant=w2157) -> (data=w2156:bool, error out=w2159:errorcluster)
              n788 = global write "S2C_FPGA_InterfaceGlobals.vi" "C1/P4/B7"(w2156) -> ()
            }
          }
        }
        frame "C2/P0/B0" {
          n789 = case "Node or Element Type Case Structure" shown="\"Read I/O\"" w2164 {
            tunnel: w2169 -> [w2174 w2179 w2184]
            tunnel: [w2173 w2179 w2183] -> w2168
            tunnel: w2167 -> [w2172 w2178 w2186]
            tunnel: [w2171 w2178 w2186] -> w2166
            tunnel: [variant[] [] w2175 _] -> w2165
            tunnel: w2163 -> [_ _ w2185]
            frame Default {
              # "5"
              n790 = call <vilib>:"Report Support Error.vi"("sim I/O info in"=w2172, "error in (no error)"=w2174) -> ("sim I/O info out"=w2171:T1, "error out"=w2173:errorcluster)  [unwired: 12 out]
            }
            frame "Read I/O" {
              n791 = global read "S2C_FPGA_InterfaceGlobals.vi" "C2/P0/B0"() -> (w2177:bool)
              n792 = To Variant(anything=w2177) -> (Variant=w2176:variant)
              n793 = Build Array(w2176) -> (w2175:variant[])
            }
            frame "Write I/O" {
              n794 = Index Array(array=w2185) -> (element=w2181:variant)  [unwired: 1 in]
              n795 = Variant To Data(error in=w2184, type=TRUE, Variant=w2181) -> (data=w2180:bool, error out=w2183:errorcluster)
              n796 = global write "S2C_FPGA_InterfaceGlobals.vi" "C2/P0/B0"(w2180) -> ()
            }
          }
        }
        frame "C2/P0/B1" {
          n797 = case "Node or Element Type Case Structure" shown="\"Write I/O\"" w2188 {
            tunnel: w2193 -> [w2198 w2203 w2208]
            tunnel: [w2197 w2203 w2207] -> w2192
            tunnel: w2191 -> [w2196 w2202 w2210]
            tunnel: [w2195 w2202 w2210] -> w2190
            tunnel: [variant[] [] w2199 _] -> w2189
            tunnel: w2187 -> [_ _ w2209]
            frame Default {
              # "5"
              n798 = call <vilib>:"Report Support Error.vi"("sim I/O info in"=w2196, "error in (no error)"=w2198) -> ("sim I/O info out"=w2195:T1, "error out"=w2197:errorcluster)  [unwired: 12 out]
            }
            frame "Read I/O" {
              n799 = global read "S2C_FPGA_InterfaceGlobals.vi" "C2/P0/B1"() -> (w2201:bool)
              n800 = To Variant(anything=w2201) -> (Variant=w2200:variant)
              n801 = Build Array(w2200) -> (w2199:variant[])
            }
            frame "Write I/O" {
              n802 = Index Array(array=w2209) -> (element=w2205:variant)  [unwired: 1 in]
              n803 = Variant To Data(error in=w2208, type=TRUE, Variant=w2205) -> (data=w2204:bool, error out=w2207:errorcluster)
              n804 = global write "S2C_FPGA_InterfaceGlobals.vi" "C2/P0/B1"(w2204) -> ()
            }
          }
        }
        frame "C2/P0/B2" {
          n805 = case "Node or Element Type Case Structure" shown="\"Read I/O\"" w2212 {
            tunnel: w2217 -> [w2222 w2227 w2232]
            tunnel: [w2221 w2227 w2231] -> w2216
            tunnel: w2215 -> [w2220 w2226 w2234]
            tunnel: [w2219 w2226 w2234] -> w2214
            tunnel: [variant[] [] w2223 _] -> w2213
            tunnel: w2211 -> [_ _ w2233]
            frame Default {
              # "5"
              n806 = call <vilib>:"Report Support Error.vi"("sim I/O info in"=w2220, "error in (no error)"=w2222) -> ("sim I/O info out"=w2219:T1, "error out"=w2221:errorcluster)  [unwired: 12 out]
            }
            frame "Read I/O" {
              n807 = global read "S2C_FPGA_InterfaceGlobals.vi" "C2/P0/B2"() -> (w2225:bool)
              n808 = To Variant(anything=w2225) -> (Variant=w2224:variant)
              n809 = Build Array(w2224) -> (w2223:variant[])
            }
            frame "Write I/O" {
              n810 = Index Array(array=w2233) -> (element=w2229:variant)  [unwired: 1 in]
              n811 = Variant To Data(error in=w2232, type=TRUE, Variant=w2229) -> (data=w2228:bool, error out=w2231:errorcluster)
              n812 = global write "S2C_FPGA_InterfaceGlobals.vi" "C2/P0/B2"(w2228) -> ()
            }
          }
        }
        frame "C2/P0/B3" {
          n813 = case "Node or Element Type Case Structure" shown="\"Write I/O\"" w2236 {
            tunnel: w2241 -> [w2246 w2251 w2256]
            tunnel: [w2245 w2251 w2255] -> w2240
            tunnel: w2239 -> [w2244 w2250 w2258]
            tunnel: [w2243 w2250 w2258] -> w2238
            tunnel: [variant[] [] w2247 _] -> w2237
            tunnel: w2235 -> [_ _ w2257]
            frame Default {
              # "5"
              n814 = call <vilib>:"Report Support Error.vi"("sim I/O info in"=w2244, "error in (no error)"=w2246) -> ("sim I/O info out"=w2243:T1, "error out"=w2245:errorcluster)  [unwired: 12 out]
            }
            frame "Read I/O" {
              n815 = global read "S2C_FPGA_InterfaceGlobals.vi" "C2/P0/B3"() -> (w2249:bool)
              n816 = To Variant(anything=w2249) -> (Variant=w2248:variant)
              n817 = Build Array(w2248) -> (w2247:variant[])
            }
            frame "Write I/O" {
              n818 = Index Array(array=w2257) -> (element=w2253:variant)  [unwired: 1 in]
              n819 = Variant To Data(error in=w2256, type=TRUE, Variant=w2253) -> (data=w2252:bool, error out=w2255:errorcluster)
              n820 = global write "S2C_FPGA_InterfaceGlobals.vi" "C2/P0/B3"(w2252) -> ()
            }
          }
        }
        frame "C2/P0/B4" {
          n821 = case "Node or Element Type Case Structure" shown="\"Read I/O\"" w2260 {
            tunnel: w2265 -> [w2270 w2275 w2280]
            tunnel: [w2269 w2275 w2279] -> w2264
            tunnel: w2263 -> [w2268 w2274 w2282]
            tunnel: [w2267 w2274 w2282] -> w2262
            tunnel: [variant[] [] w2271 _] -> w2261
            tunnel: w2259 -> [_ _ w2281]
            frame Default {
              # "5"
              n822 = call <vilib>:"Report Support Error.vi"("sim I/O info in"=w2268, "error in (no error)"=w2270) -> ("sim I/O info out"=w2267:T1, "error out"=w2269:errorcluster)  [unwired: 12 out]
            }
            frame "Read I/O" {
              n823 = global read "S2C_FPGA_InterfaceGlobals.vi" "C2/P0/B4"() -> (w2273:bool)
              n824 = To Variant(anything=w2273) -> (Variant=w2272:variant)
              n825 = Build Array(w2272) -> (w2271:variant[])
            }
            frame "Write I/O" {
              n826 = Index Array(array=w2281) -> (element=w2277:variant)  [unwired: 1 in]
              n827 = Variant To Data(error in=w2280, type=TRUE, Variant=w2277) -> (data=w2276:bool, error out=w2279:errorcluster)
              n828 = global write "S2C_FPGA_InterfaceGlobals.vi" "C2/P0/B4"(w2276) -> ()
            }
          }
        }
        frame "C2/P0/B5" {
          n829 = case "Node or Element Type Case Structure" shown="\"Write I/O\"" w2284 {
            tunnel: w2289 -> [w2294 w2299 w2304]
            tunnel: [w2293 w2299 w2303] -> w2288
            tunnel: w2287 -> [w2292 w2298 w2306]
            tunnel: [w2291 w2298 w2306] -> w2286
            tunnel: [variant[] [] w2295 _] -> w2285
            tunnel: w2283 -> [_ _ w2305]
            frame Default {
              # "5"
              n830 = call <vilib>:"Report Support Error.vi"("sim I/O info in"=w2292, "error in (no error)"=w2294) -> ("sim I/O info out"=w2291:T1, "error out"=w2293:errorcluster)  [unwired: 12 out]
            }
            frame "Read I/O" {
              n831 = global read "S2C_FPGA_InterfaceGlobals.vi" "C2/P0/B5"() -> (w2297:bool)
              n832 = To Variant(anything=w2297) -> (Variant=w2296:variant)
              n833 = Build Array(w2296) -> (w2295:variant[])
            }
            frame "Write I/O" {
              n834 = Index Array(array=w2305) -> (element=w2301:variant)  [unwired: 1 in]
              n835 = Variant To Data(error in=w2304, type=TRUE, Variant=w2301) -> (data=w2300:bool, error out=w2303:errorcluster)
              n836 = global write "S2C_FPGA_InterfaceGlobals.vi" "C2/P0/B5"(w2300) -> ()
            }
          }
        }
        frame "C2/P0/B6" {
          n837 = case "Node or Element Type Case Structure" shown="\"Read I/O\"" w2308 {
            tunnel: w2313 -> [w2318 w2323 w2328]
            tunnel: [w2317 w2323 w2327] -> w2312
            tunnel: w2311 -> [w2316 w2322 w2330]
            tunnel: [w2315 w2322 w2330] -> w2310
            tunnel: [variant[] [] w2319 _] -> w2309
            tunnel: w2307 -> [_ _ w2329]
            frame Default {
              # "5"
              n838 = call <vilib>:"Report Support Error.vi"("sim I/O info in"=w2316, "error in (no error)"=w2318) -> ("sim I/O info out"=w2315:T1, "error out"=w2317:errorcluster)  [unwired: 12 out]
            }
            frame "Read I/O" {
              n839 = global read "S2C_FPGA_InterfaceGlobals.vi" "C2/P0/B6"() -> (w2321:bool)
              n840 = To Variant(anything=w2321) -> (Variant=w2320:variant)
              n841 = Build Array(w2320) -> (w2319:variant[])
            }
            frame "Write I/O" {
              n842 = Index Array(array=w2329) -> (element=w2325:variant)  [unwired: 1 in]
              n843 = Variant To Data(error in=w2328, type=TRUE, Variant=w2325) -> (data=w2324:bool, error out=w2327:errorcluster)
              n844 = global write "S2C_FPGA_InterfaceGlobals.vi" "C2/P0/B6"(w2324) -> ()
            }
          }
        }
        frame "C2/P0/B7" {
          n845 = case "Node or Element Type Case Structure" shown="\"Write I/O\"" w2332 {
            tunnel: w2337 -> [w2342 w2347 w2352]
            tunnel: [w2341 w2347 w2351] -> w2336
            tunnel: w2335 -> [w2340 w2346 w2354]
            tunnel: [w2339 w2346 w2354] -> w2334
            tunnel: [variant[] [] w2343 _] -> w2333
            tunnel: w2331 -> [_ _ w2353]
            frame Default {
              # "5"
              n846 = call <vilib>:"Report Support Error.vi"("sim I/O info in"=w2340, "error in (no error)"=w2342) -> ("sim I/O info out"=w2339:T1, "error out"=w2341:errorcluster)  [unwired: 12 out]
            }
            frame "Read I/O" {
              n847 = global read "S2C_FPGA_InterfaceGlobals.vi" "C2/P0/B7"() -> (w2345:bool)
              n848 = To Variant(anything=w2345) -> (Variant=w2344:variant)
              n849 = Build Array(w2344) -> (w2343:variant[])
            }
            frame "Write I/O" {
              n850 = Index Array(array=w2353) -> (element=w2349:variant)  [unwired: 1 in]
              n851 = Variant To Data(error in=w2352, type=TRUE, Variant=w2349) -> (data=w2348:bool, error out=w2351:errorcluster)
              n852 = global write "S2C_FPGA_InterfaceGlobals.vi" "C2/P0/B7"(w2348) -> ()
            }
          }
        }
        frame "C2/P1/B0" {
          n853 = case "Node or Element Type Case Structure" shown="\"Read I/O\"" w2356 {
            tunnel: w2361 -> [w2366 w2371 w2376]
            tunnel: [w2365 w2371 w2375] -> w2360
            tunnel: w2359 -> [w2364 w2370 w2378]
            tunnel: [w2363 w2370 w2378] -> w2358
            tunnel: [variant[] [] w2367 _] -> w2357
            tunnel: w2355 -> [_ _ w2377]
            frame Default {
              # "5"
              n854 = call <vilib>:"Report Support Error.vi"("sim I/O info in"=w2364, "error in (no error)"=w2366) -> ("sim I/O info out"=w2363:T1, "error out"=w2365:errorcluster)  [unwired: 12 out]
            }
            frame "Read I/O" {
              n855 = global read "S2C_FPGA_InterfaceGlobals.vi" "C2/P1/B0"() -> (w2369:bool)
              n856 = To Variant(anything=w2369) -> (Variant=w2368:variant)
              n857 = Build Array(w2368) -> (w2367:variant[])
            }
            frame "Write I/O" {
              n858 = Index Array(array=w2377) -> (element=w2373:variant)  [unwired: 1 in]
              n859 = Variant To Data(error in=w2376, type=TRUE, Variant=w2373) -> (data=w2372:bool, error out=w2375:errorcluster)
              n860 = global write "S2C_FPGA_InterfaceGlobals.vi" "C2/P1/B0"(w2372) -> ()
            }
          }
        }
        frame "C2/P1/B1" {
          n861 = case "Node or Element Type Case Structure" shown="\"Write I/O\"" w2380 {
            tunnel: w2385 -> [w2390 w2395 w2400]
            tunnel: [w2389 w2395 w2399] -> w2384
            tunnel: w2383 -> [w2388 w2394 w2402]
            tunnel: [w2387 w2394 w2402] -> w2382
            tunnel: [variant[] [] w2391 _] -> w2381
            tunnel: w2379 -> [_ _ w2401]
            frame Default {
              # "5"
              n862 = call <vilib>:"Report Support Error.vi"("sim I/O info in"=w2388, "error in (no error)"=w2390) -> ("sim I/O info out"=w2387:T1, "error out"=w2389:errorcluster)  [unwired: 12 out]
            }
            frame "Read I/O" {
              n863 = global read "S2C_FPGA_InterfaceGlobals.vi" "C2/P1/B1"() -> (w2393:bool)
              n864 = To Variant(anything=w2393) -> (Variant=w2392:variant)
              n865 = Build Array(w2392) -> (w2391:variant[])
            }
            frame "Write I/O" {
              n866 = Index Array(array=w2401) -> (element=w2397:variant)  [unwired: 1 in]
              n867 = Variant To Data(error in=w2400, type=TRUE, Variant=w2397) -> (data=w2396:bool, error out=w2399:errorcluster)
              n868 = global write "S2C_FPGA_InterfaceGlobals.vi" "C2/P1/B1"(w2396) -> ()
            }
          }
        }
        frame "C2/P1/B2" {
          n869 = case "Node or Element Type Case Structure" shown="\"Read I/O\"" w2404 {
            tunnel: w2409 -> [w2414 w2419 w2424]
            tunnel: [w2413 w2419 w2423] -> w2408
            tunnel: w2407 -> [w2412 w2418 w2426]
            tunnel: [w2411 w2418 w2426] -> w2406
            tunnel: [variant[] [] w2415 _] -> w2405
            tunnel: w2403 -> [_ _ w2425]
            frame Default {
              # "5"
              n870 = call <vilib>:"Report Support Error.vi"("sim I/O info in"=w2412, "error in (no error)"=w2414) -> ("sim I/O info out"=w2411:T1, "error out"=w2413:errorcluster)  [unwired: 12 out]
            }
            frame "Read I/O" {
              n871 = global read "S2C_FPGA_InterfaceGlobals.vi" "C2/P1/B2"() -> (w2417:bool)
              n872 = To Variant(anything=w2417) -> (Variant=w2416:variant)
              n873 = Build Array(w2416) -> (w2415:variant[])
            }
            frame "Write I/O" {
              n874 = Index Array(array=w2425) -> (element=w2421:variant)  [unwired: 1 in]
              n875 = Variant To Data(error in=w2424, type=TRUE, Variant=w2421) -> (data=w2420:bool, error out=w2423:errorcluster)
              n876 = global write "S2C_FPGA_InterfaceGlobals.vi" "C2/P1/B2"(w2420) -> ()
            }
          }
        }
        frame "C2/P1/B3" {
          n877 = case "Node or Element Type Case Structure" shown="\"Write I/O\"" w2428 {
            tunnel: w2433 -> [w2438 w2443 w2448]
            tunnel: [w2437 w2443 w2447] -> w2432
            tunnel: w2431 -> [w2436 w2442 w2450]
            tunnel: [w2435 w2442 w2450] -> w2430
            tunnel: [variant[] [] w2439 _] -> w2429
            tunnel: w2427 -> [_ _ w2449]
            frame Default {
              # "5"
              n878 = call <vilib>:"Report Support Error.vi"("sim I/O info in"=w2436, "error in (no error)"=w2438) -> ("sim I/O info out"=w2435:T1, "error out"=w2437:errorcluster)  [unwired: 12 out]
            }
            frame "Read I/O" {
              n879 = global read "S2C_FPGA_InterfaceGlobals.vi" "C2/P1/B3"() -> (w2441:bool)
              n880 = To Variant(anything=w2441) -> (Variant=w2440:variant)
              n881 = Build Array(w2440) -> (w2439:variant[])
            }
            frame "Write I/O" {
              n882 = Index Array(array=w2449) -> (element=w2445:variant)  [unwired: 1 in]
              n883 = Variant To Data(error in=w2448, type=TRUE, Variant=w2445) -> (data=w2444:bool, error out=w2447:errorcluster)
              n884 = global write "S2C_FPGA_InterfaceGlobals.vi" "C2/P1/B3"(w2444) -> ()
            }
          }
        }
        frame "C2/P1/B4" {
          n885 = case "Node or Element Type Case Structure" shown="\"Read I/O\"" w2452 {
            tunnel: w2457 -> [w2462 w2467 w2472]
            tunnel: [w2461 w2467 w2471] -> w2456
            tunnel: w2455 -> [w2460 w2466 w2474]
            tunnel: [w2459 w2466 w2474] -> w2454
            tunnel: [variant[] [] w2463 _] -> w2453
            tunnel: w2451 -> [_ _ w2473]
            frame Default {
              # "5"
              n886 = call <vilib>:"Report Support Error.vi"("sim I/O info in"=w2460, "error in (no error)"=w2462) -> ("sim I/O info out"=w2459:T1, "error out"=w2461:errorcluster)  [unwired: 12 out]
            }
            frame "Read I/O" {
              n887 = global read "S2C_FPGA_InterfaceGlobals.vi" "C2/P1/B4"() -> (w2465:bool)
              n888 = To Variant(anything=w2465) -> (Variant=w2464:variant)
              n889 = Build Array(w2464) -> (w2463:variant[])
            }
            frame "Write I/O" {
              n890 = Index Array(array=w2473) -> (element=w2469:variant)  [unwired: 1 in]
              n891 = Variant To Data(error in=w2472, type=TRUE, Variant=w2469) -> (data=w2468:bool, error out=w2471:errorcluster)
              n892 = global write "S2C_FPGA_InterfaceGlobals.vi" "C2/P1/B4"(w2468) -> ()
            }
          }
        }
        frame "C2/P1/B5" {
          n893 = case "Node or Element Type Case Structure" shown="\"Write I/O\"" w2476 {
            tunnel: w2481 -> [w2486 w2491 w2496]
            tunnel: [w2485 w2491 w2495] -> w2480
            tunnel: w2479 -> [w2484 w2490 w2498]
            tunnel: [w2483 w2490 w2498] -> w2478
            tunnel: [variant[] [] w2487 _] -> w2477
            tunnel: w2475 -> [_ _ w2497]
            frame Default {
              # "5"
              n894 = call <vilib>:"Report Support Error.vi"("sim I/O info in"=w2484, "error in (no error)"=w2486) -> ("sim I/O info out"=w2483:T1, "error out"=w2485:errorcluster)  [unwired: 12 out]
            }
            frame "Read I/O" {
              n895 = global read "S2C_FPGA_InterfaceGlobals.vi" "C2/P1/B5"() -> (w2489:bool)
              n896 = To Variant(anything=w2489) -> (Variant=w2488:variant)
              n897 = Build Array(w2488) -> (w2487:variant[])
            }
            frame "Write I/O" {
              n898 = Index Array(array=w2497) -> (element=w2493:variant)  [unwired: 1 in]
              n899 = Variant To Data(error in=w2496, type=TRUE, Variant=w2493) -> (data=w2492:bool, error out=w2495:errorcluster)
              n900 = global write "S2C_FPGA_InterfaceGlobals.vi" "C2/P1/B5"(w2492) -> ()
            }
          }
        }
        frame "C2/P1/B6" {
          n901 = case "Node or Element Type Case Structure" shown="\"Read I/O\"" w2500 {
            tunnel: w2505 -> [w2510 w2515 w2520]
            tunnel: [w2509 w2515 w2519] -> w2504
            tunnel: w2503 -> [w2508 w2514 w2522]
            tunnel: [w2507 w2514 w2522] -> w2502
            tunnel: [variant[] [] w2511 _] -> w2501
            tunnel: w2499 -> [_ _ w2521]
            frame Default {
              # "5"
              n902 = call <vilib>:"Report Support Error.vi"("sim I/O info in"=w2508, "error in (no error)"=w2510) -> ("sim I/O info out"=w2507:T1, "error out"=w2509:errorcluster)  [unwired: 12 out]
            }
            frame "Read I/O" {
              n903 = global read "S2C_FPGA_InterfaceGlobals.vi" "C2/P1/B6"() -> (w2513:bool)
              n904 = To Variant(anything=w2513) -> (Variant=w2512:variant)
              n905 = Build Array(w2512) -> (w2511:variant[])
            }
            frame "Write I/O" {
              n906 = Index Array(array=w2521) -> (element=w2517:variant)  [unwired: 1 in]
              n907 = Variant To Data(error in=w2520, type=TRUE, Variant=w2517) -> (data=w2516:bool, error out=w2519:errorcluster)
              n908 = global write "S2C_FPGA_InterfaceGlobals.vi" "C2/P1/B6"(w2516) -> ()
            }
          }
        }
        frame "C2/P1/B7" {
          n909 = case "Node or Element Type Case Structure" shown="\"Write I/O\"" w2524 {
            tunnel: w2529 -> [w2534 w2539 w2544]
            tunnel: [w2533 w2539 w2543] -> w2528
            tunnel: w2527 -> [w2532 w2538 w2546]
            tunnel: [w2531 w2538 w2546] -> w2526
            tunnel: [variant[] [] w2535 _] -> w2525
            tunnel: w2523 -> [_ _ w2545]
            frame Default {
              # "5"
              n910 = call <vilib>:"Report Support Error.vi"("sim I/O info in"=w2532, "error in (no error)"=w2534) -> ("sim I/O info out"=w2531:T1, "error out"=w2533:errorcluster)  [unwired: 12 out]
            }
            frame "Read I/O" {
              n911 = global read "S2C_FPGA_InterfaceGlobals.vi" "C2/P1/B7"() -> (w2537:bool)
              n912 = To Variant(anything=w2537) -> (Variant=w2536:variant)
              n913 = Build Array(w2536) -> (w2535:variant[])
            }
            frame "Write I/O" {
              n914 = Index Array(array=w2545) -> (element=w2541:variant)  [unwired: 1 in]
              n915 = Variant To Data(error in=w2544, type=TRUE, Variant=w2541) -> (data=w2540:bool, error out=w2543:errorcluster)
              n916 = global write "S2C_FPGA_InterfaceGlobals.vi" "C2/P1/B7"(w2540) -> ()
            }
          }
        }
        frame "C2/P2/B0" {
          n917 = case "Node or Element Type Case Structure" shown="\"Read I/O\"" w2548 {
            tunnel: w2553 -> [w2558 w2563 w2568]
            tunnel: [w2557 w2563 w2567] -> w2552
            tunnel: w2551 -> [w2556 w2562 w2570]
            tunnel: [w2555 w2562 w2570] -> w2550
            tunnel: [variant[] [] w2559 _] -> w2549
            tunnel: w2547 -> [_ _ w2569]
            frame Default {
              # "5"
              n918 = call <vilib>:"Report Support Error.vi"("sim I/O info in"=w2556, "error in (no error)"=w2558) -> ("sim I/O info out"=w2555:T1, "error out"=w2557:errorcluster)  [unwired: 12 out]
            }
            frame "Read I/O" {
              n919 = global read "S2C_FPGA_InterfaceGlobals.vi" "C2/P2/B0"() -> (w2561:bool)
              n920 = To Variant(anything=w2561) -> (Variant=w2560:variant)
              n921 = Build Array(w2560) -> (w2559:variant[])
            }
            frame "Write I/O" {
              n922 = Index Array(array=w2569) -> (element=w2565:variant)  [unwired: 1 in]
              n923 = Variant To Data(error in=w2568, type=TRUE, Variant=w2565) -> (data=w2564:bool, error out=w2567:errorcluster)
              n924 = global write "S2C_FPGA_InterfaceGlobals.vi" "C2/P2/B0"(w2564) -> ()
            }
          }
        }
        frame "C2/P2/B1" {
          n925 = case "Node or Element Type Case Structure" shown="\"Write I/O\"" w2572 {
            tunnel: w2577 -> [w2582 w2587 w2592]
            tunnel: [w2581 w2587 w2591] -> w2576
            tunnel: w2575 -> [w2580 w2586 w2594]
            tunnel: [w2579 w2586 w2594] -> w2574
            tunnel: [variant[] [] w2583 _] -> w2573
            tunnel: w2571 -> [_ _ w2593]
            frame Default {
              # "5"
              n926 = call <vilib>:"Report Support Error.vi"("sim I/O info in"=w2580, "error in (no error)"=w2582) -> ("sim I/O info out"=w2579:T1, "error out"=w2581:errorcluster)  [unwired: 12 out]
            }
            frame "Read I/O" {
              n927 = global read "S2C_FPGA_InterfaceGlobals.vi" "C2/P2/B1"() -> (w2585:bool)
              n928 = To Variant(anything=w2585) -> (Variant=w2584:variant)
              n929 = Build Array(w2584) -> (w2583:variant[])
            }
            frame "Write I/O" {
              n930 = Index Array(array=w2593) -> (element=w2589:variant)  [unwired: 1 in]
              n931 = Variant To Data(error in=w2592, type=TRUE, Variant=w2589) -> (data=w2588:bool, error out=w2591:errorcluster)
              n932 = global write "S2C_FPGA_InterfaceGlobals.vi" "C2/P2/B1"(w2588) -> ()
            }
          }
        }
        frame "C2/P2/B2" {
          n933 = case "Node or Element Type Case Structure" shown="\"Read I/O\"" w2596 {
            tunnel: w2601 -> [w2606 w2611 w2616]
            tunnel: [w2605 w2611 w2615] -> w2600
            tunnel: w2599 -> [w2604 w2610 w2618]
            tunnel: [w2603 w2610 w2618] -> w2598
            tunnel: [variant[] [] w2607 _] -> w2597
            tunnel: w2595 -> [_ _ w2617]
            frame Default {
              # "5"
              n934 = call <vilib>:"Report Support Error.vi"("sim I/O info in"=w2604, "error in (no error)"=w2606) -> ("sim I/O info out"=w2603:T1, "error out"=w2605:errorcluster)  [unwired: 12 out]
            }
            frame "Read I/O" {
              n935 = global read "S2C_FPGA_InterfaceGlobals.vi" "C2/P2/B2"() -> (w2609:bool)
              n936 = To Variant(anything=w2609) -> (Variant=w2608:variant)
              n937 = Build Array(w2608) -> (w2607:variant[])
            }
            frame "Write I/O" {
              n938 = Index Array(array=w2617) -> (element=w2613:variant)  [unwired: 1 in]
              n939 = Variant To Data(error in=w2616, type=TRUE, Variant=w2613) -> (data=w2612:bool, error out=w2615:errorcluster)
              n940 = global write "S2C_FPGA_InterfaceGlobals.vi" "C2/P2/B2"(w2612) -> ()
            }
          }
        }
        frame "C2/P2/B3" {
          n941 = case "Node or Element Type Case Structure" shown="\"Write I/O\"" w2620 {
            tunnel: w2625 -> [w2630 w2635 w2640]
            tunnel: [w2629 w2635 w2639] -> w2624
            tunnel: w2623 -> [w2628 w2634 w2642]
            tunnel: [w2627 w2634 w2642] -> w2622
            tunnel: [variant[] [] w2631 _] -> w2621
            tunnel: w2619 -> [_ _ w2641]
            frame Default {
              # "5"
              n942 = call <vilib>:"Report Support Error.vi"("sim I/O info in"=w2628, "error in (no error)"=w2630) -> ("sim I/O info out"=w2627:T1, "error out"=w2629:errorcluster)  [unwired: 12 out]
            }
            frame "Read I/O" {
              n943 = global read "S2C_FPGA_InterfaceGlobals.vi" "C2/P2/B3"() -> (w2633:bool)
              n944 = To Variant(anything=w2633) -> (Variant=w2632:variant)
              n945 = Build Array(w2632) -> (w2631:variant[])
            }
            frame "Write I/O" {
              n946 = Index Array(array=w2641) -> (element=w2637:variant)  [unwired: 1 in]
              n947 = Variant To Data(error in=w2640, type=TRUE, Variant=w2637) -> (data=w2636:bool, error out=w2639:errorcluster)
              n948 = global write "S2C_FPGA_InterfaceGlobals.vi" "C2/P2/B3"(w2636) -> ()
            }
          }
        }
        frame "C2/P2/B4" {
          n949 = case "Node or Element Type Case Structure" shown="\"Read I/O\"" w2644 {
            tunnel: w2649 -> [w2654 w2659 w2664]
            tunnel: [w2653 w2659 w2663] -> w2648
            tunnel: w2647 -> [w2652 w2658 w2666]
            tunnel: [w2651 w2658 w2666] -> w2646
            tunnel: [variant[] [] w2655 _] -> w2645
            tunnel: w2643 -> [_ _ w2665]
            frame Default {
              # "5"
              n950 = call <vilib>:"Report Support Error.vi"("sim I/O info in"=w2652, "error in (no error)"=w2654) -> ("sim I/O info out"=w2651:T1, "error out"=w2653:errorcluster)  [unwired: 12 out]
            }
            frame "Read I/O" {
              n951 = global read "S2C_FPGA_InterfaceGlobals.vi" "C2/P2/B4"() -> (w2657:bool)
              n952 = To Variant(anything=w2657) -> (Variant=w2656:variant)
              n953 = Build Array(w2656) -> (w2655:variant[])
            }
            frame "Write I/O" {
              n954 = Index Array(array=w2665) -> (element=w2661:variant)  [unwired: 1 in]
              n955 = Variant To Data(error in=w2664, type=TRUE, Variant=w2661) -> (data=w2660:bool, error out=w2663:errorcluster)
              n956 = global write "S2C_FPGA_InterfaceGlobals.vi" "C2/P2/B4"(w2660) -> ()
            }
          }
        }
        frame "C2/P2/B5" {
          n957 = case "Node or Element Type Case Structure" shown="\"Write I/O\"" w2668 {
            tunnel: w2673 -> [w2678 w2683 w2688]
            tunnel: [w2677 w2683 w2687] -> w2672
            tunnel: w2671 -> [w2676 w2682 w2690]
            tunnel: [w2675 w2682 w2690] -> w2670
            tunnel: [variant[] [] w2679 _] -> w2669
            tunnel: w2667 -> [_ _ w2689]
            frame Default {
              # "5"
              n958 = call <vilib>:"Report Support Error.vi"("sim I/O info in"=w2676, "error in (no error)"=w2678) -> ("sim I/O info out"=w2675:T1, "error out"=w2677:errorcluster)  [unwired: 12 out]
            }
            frame "Read I/O" {
              n959 = global read "S2C_FPGA_InterfaceGlobals.vi" "C2/P2/B5"() -> (w2681:bool)
              n960 = To Variant(anything=w2681) -> (Variant=w2680:variant)
              n961 = Build Array(w2680) -> (w2679:variant[])
            }
            frame "Write I/O" {
              n962 = Index Array(array=w2689) -> (element=w2685:variant)  [unwired: 1 in]
              n963 = Variant To Data(error in=w2688, type=TRUE, Variant=w2685) -> (data=w2684:bool, error out=w2687:errorcluster)
              n964 = global write "S2C_FPGA_InterfaceGlobals.vi" "C2/P2/B5"(w2684) -> ()
            }
          }
        }
        frame "C2/P2/B6" {
          n965 = case "Node or Element Type Case Structure" shown="\"Read I/O\"" w2692 {
            tunnel: w2697 -> [w2702 w2707 w2712]
            tunnel: [w2701 w2707 w2711] -> w2696
            tunnel: w2695 -> [w2700 w2706 w2714]
            tunnel: [w2699 w2706 w2714] -> w2694
            tunnel: [variant[] [] w2703 _] -> w2693
            tunnel: w2691 -> [_ _ w2713]
            frame Default {
              # "5"
              n966 = call <vilib>:"Report Support Error.vi"("sim I/O info in"=w2700, "error in (no error)"=w2702) -> ("sim I/O info out"=w2699:T1, "error out"=w2701:errorcluster)  [unwired: 12 out]
            }
            frame "Read I/O" {
              n967 = global read "S2C_FPGA_InterfaceGlobals.vi" "C2/P2/B6"() -> (w2705:bool)
              n968 = To Variant(anything=w2705) -> (Variant=w2704:variant)
              n969 = Build Array(w2704) -> (w2703:variant[])
            }
            frame "Write I/O" {
              n970 = Index Array(array=w2713) -> (element=w2709:variant)  [unwired: 1 in]
              n971 = Variant To Data(error in=w2712, type=TRUE, Variant=w2709) -> (data=w2708:bool, error out=w2711:errorcluster)
              n972 = global write "S2C_FPGA_InterfaceGlobals.vi" "C2/P2/B6"(w2708) -> ()
            }
          }
        }
        frame "C2/P2/B7" {
          n973 = case "Node or Element Type Case Structure" shown="\"Write I/O\"" w2716 {
            tunnel: w2721 -> [w2726 w2731 w2736]
            tunnel: [w2725 w2731 w2735] -> w2720
            tunnel: w2719 -> [w2724 w2730 w2738]
            tunnel: [w2723 w2730 w2738] -> w2718
            tunnel: [variant[] [] w2727 _] -> w2717
            tunnel: w2715 -> [_ _ w2737]
            frame Default {
              # "5"
              n974 = call <vilib>:"Report Support Error.vi"("sim I/O info in"=w2724, "error in (no error)"=w2726) -> ("sim I/O info out"=w2723:T1, "error out"=w2725:errorcluster)  [unwired: 12 out]
            }
            frame "Read I/O" {
              n975 = global read "S2C_FPGA_InterfaceGlobals.vi" "C2/P2/B7"() -> (w2729:bool)
              n976 = To Variant(anything=w2729) -> (Variant=w2728:variant)
              n977 = Build Array(w2728) -> (w2727:variant[])
            }
            frame "Write I/O" {
              n978 = Index Array(array=w2737) -> (element=w2733:variant)  [unwired: 1 in]
              n979 = Variant To Data(error in=w2736, type=TRUE, Variant=w2733) -> (data=w2732:bool, error out=w2735:errorcluster)
              n980 = global write "S2C_FPGA_InterfaceGlobals.vi" "C2/P2/B7"(w2732) -> ()
            }
          }
        }
        frame "C2/P3/B0" {
          n981 = case "Node or Element Type Case Structure" shown="\"Read I/O\"" w2740 {
            tunnel: w2745 -> [w2750 w2755 w2760]
            tunnel: [w2749 w2755 w2759] -> w2744
            tunnel: w2743 -> [w2748 w2754 w2762]
            tunnel: [w2747 w2754 w2762] -> w2742
            tunnel: [variant[] [] w2751 _] -> w2741
            tunnel: w2739 -> [_ _ w2761]
            frame Default {
              # "5"
              n982 = call <vilib>:"Report Support Error.vi"("sim I/O info in"=w2748, "error in (no error)"=w2750) -> ("sim I/O info out"=w2747:T1, "error out"=w2749:errorcluster)  [unwired: 12 out]
            }
            frame "Read I/O" {
              n983 = global read "S2C_FPGA_InterfaceGlobals.vi" "C2/P3/B0"() -> (w2753:bool)
              n984 = To Variant(anything=w2753) -> (Variant=w2752:variant)
              n985 = Build Array(w2752) -> (w2751:variant[])
            }
            frame "Write I/O" {
              n986 = Index Array(array=w2761) -> (element=w2757:variant)  [unwired: 1 in]
              n987 = Variant To Data(error in=w2760, type=TRUE, Variant=w2757) -> (data=w2756:bool, error out=w2759:errorcluster)
              n988 = global write "S2C_FPGA_InterfaceGlobals.vi" "C2/P3/B0"(w2756) -> ()
            }
          }
        }
        frame "C2/P3/B1" {
          n989 = case "Node or Element Type Case Structure" shown="\"Write I/O\"" w2764 {
            tunnel: w2769 -> [w2774 w2779 w2784]
            tunnel: [w2773 w2779 w2783] -> w2768
            tunnel: w2767 -> [w2772 w2778 w2786]
            tunnel: [w2771 w2778 w2786] -> w2766
            tunnel: [variant[] [] w2775 _] -> w2765
            tunnel: w2763 -> [_ _ w2785]
            frame Default {
              # "5"
              n990 = call <vilib>:"Report Support Error.vi"("sim I/O info in"=w2772, "error in (no error)"=w2774) -> ("sim I/O info out"=w2771:T1, "error out"=w2773:errorcluster)  [unwired: 12 out]
            }
            frame "Read I/O" {
              n991 = global read "S2C_FPGA_InterfaceGlobals.vi" "C2/P3/B1"() -> (w2777:bool)
              n992 = To Variant(anything=w2777) -> (Variant=w2776:variant)
              n993 = Build Array(w2776) -> (w2775:variant[])
            }
            frame "Write I/O" {
              n994 = Index Array(array=w2785) -> (element=w2781:variant)  [unwired: 1 in]
              n995 = Variant To Data(error in=w2784, type=TRUE, Variant=w2781) -> (data=w2780:bool, error out=w2783:errorcluster)
              n996 = global write "S2C_FPGA_InterfaceGlobals.vi" "C2/P3/B1"(w2780) -> ()
            }
          }
        }
        frame "C2/P3/B2" {
          n997 = case "Node or Element Type Case Structure" shown="\"Read I/O\"" w2788 {
            tunnel: w2793 -> [w2798 w2803 w2808]
            tunnel: [w2797 w2803 w2807] -> w2792
            tunnel: w2791 -> [w2796 w2802 w2810]
            tunnel: [w2795 w2802 w2810] -> w2790
            tunnel: [variant[] [] w2799 _] -> w2789
            tunnel: w2787 -> [_ _ w2809]
            frame Default {
              # "5"
              n998 = call <vilib>:"Report Support Error.vi"("sim I/O info in"=w2796, "error in (no error)"=w2798) -> ("sim I/O info out"=w2795:T1, "error out"=w2797:errorcluster)  [unwired: 12 out]
            }
            frame "Read I/O" {
              n999 = global read "S2C_FPGA_InterfaceGlobals.vi" "C2/P3/B2"() -> (w2801:bool)
              n1000 = To Variant(anything=w2801) -> (Variant=w2800:variant)
              n1001 = Build Array(w2800) -> (w2799:variant[])
            }
            frame "Write I/O" {
              n1002 = Index Array(array=w2809) -> (element=w2805:variant)  [unwired: 1 in]
              n1003 = Variant To Data(error in=w2808, type=TRUE, Variant=w2805) -> (data=w2804:bool, error out=w2807:errorcluster)
              n1004 = global write "S2C_FPGA_InterfaceGlobals.vi" "C2/P3/B2"(w2804) -> ()
            }
          }
        }
        frame "C2/P3/B3" {
          n1005 = case "Node or Element Type Case Structure" shown="\"Write I/O\"" w2812 {
            tunnel: w2817 -> [w2822 w2827 w2832]
            tunnel: [w2821 w2827 w2831] -> w2816
            tunnel: w2815 -> [w2820 w2826 w2834]
            tunnel: [w2819 w2826 w2834] -> w2814
            tunnel: [variant[] [] w2823 _] -> w2813
            tunnel: w2811 -> [_ _ w2833]
            frame Default {
              # "5"
              n1006 = call <vilib>:"Report Support Error.vi"("sim I/O info in"=w2820, "error in (no error)"=w2822) -> ("sim I/O info out"=w2819:T1, "error out"=w2821:errorcluster)  [unwired: 12 out]
            }
            frame "Read I/O" {
              n1007 = global read "S2C_FPGA_InterfaceGlobals.vi" "C2/P3/B3"() -> (w2825:bool)
              n1008 = To Variant(anything=w2825) -> (Variant=w2824:variant)
              n1009 = Build Array(w2824) -> (w2823:variant[])
            }
            frame "Write I/O" {
              n1010 = Index Array(array=w2833) -> (element=w2829:variant)  [unwired: 1 in]
              n1011 = Variant To Data(error in=w2832, type=TRUE, Variant=w2829) -> (data=w2828:bool, error out=w2831:errorcluster)
              n1012 = global write "S2C_FPGA_InterfaceGlobals.vi" "C2/P3/B3"(w2828) -> ()
            }
          }
        }
        frame "C2/P3/B4" {
          n1013 = case "Node or Element Type Case Structure" shown="\"Read I/O\"" w2836 {
            tunnel: w2841 -> [w2846 w2851 w2856]
            tunnel: [w2845 w2851 w2855] -> w2840
            tunnel: w2839 -> [w2844 w2850 w2858]
            tunnel: [w2843 w2850 w2858] -> w2838
            tunnel: [variant[] [] w2847 _] -> w2837
            tunnel: w2835 -> [_ _ w2857]
            frame Default {
              # "5"
              n1014 = call <vilib>:"Report Support Error.vi"("sim I/O info in"=w2844, "error in (no error)"=w2846) -> ("sim I/O info out"=w2843:T1, "error out"=w2845:errorcluster)  [unwired: 12 out]
            }
            frame "Read I/O" {
              n1015 = global read "S2C_FPGA_InterfaceGlobals.vi" "C2/P3/B4"() -> (w2849:bool)
              n1016 = To Variant(anything=w2849) -> (Variant=w2848:variant)
              n1017 = Build Array(w2848) -> (w2847:variant[])
            }
            frame "Write I/O" {
              n1018 = Index Array(array=w2857) -> (element=w2853:variant)  [unwired: 1 in]
              n1019 = Variant To Data(error in=w2856, type=TRUE, Variant=w2853) -> (data=w2852:bool, error out=w2855:errorcluster)
              n1020 = global write "S2C_FPGA_InterfaceGlobals.vi" "C2/P3/B4"(w2852) -> ()
            }
          }
        }
        frame "C2/P3/B5" {
          n1021 = case "Node or Element Type Case Structure" shown="\"Write I/O\"" w2860 {
            tunnel: w2865 -> [w2870 w2875 w2880]
            tunnel: [w2869 w2875 w2879] -> w2864
            tunnel: w2863 -> [w2868 w2874 w2882]
            tunnel: [w2867 w2874 w2882] -> w2862
            tunnel: [variant[] [] w2871 _] -> w2861
            tunnel: w2859 -> [_ _ w2881]
            frame Default {
              # "5"
              n1022 = call <vilib>:"Report Support Error.vi"("sim I/O info in"=w2868, "error in (no error)"=w2870) -> ("sim I/O info out"=w2867:T1, "error out"=w2869:errorcluster)  [unwired: 12 out]
            }
            frame "Read I/O" {
              n1023 = global read "S2C_FPGA_InterfaceGlobals.vi" "C2/P3/B5"() -> (w2873:bool)
              n1024 = To Variant(anything=w2873) -> (Variant=w2872:variant)
              n1025 = Build Array(w2872) -> (w2871:variant[])
            }
            frame "Write I/O" {
              n1026 = Index Array(array=w2881) -> (element=w2877:variant)  [unwired: 1 in]
              n1027 = Variant To Data(error in=w2880, type=TRUE, Variant=w2877) -> (data=w2876:bool, error out=w2879:errorcluster)
              n1028 = global write "S2C_FPGA_InterfaceGlobals.vi" "C2/P3/B5"(w2876) -> ()
            }
          }
        }
        frame "C2/P3/B6" {
          n1029 = case "Node or Element Type Case Structure" shown="\"Read I/O\"" w2884 {
            tunnel: w2889 -> [w2894 w2899 w2904]
            tunnel: [w2893 w2899 w2903] -> w2888
            tunnel: w2887 -> [w2892 w2898 w2906]
            tunnel: [w2891 w2898 w2906] -> w2886
            tunnel: [variant[] [] w2895 _] -> w2885
            tunnel: w2883 -> [_ _ w2905]
            frame Default {
              # "5"
              n1030 = call <vilib>:"Report Support Error.vi"("sim I/O info in"=w2892, "error in (no error)"=w2894) -> ("sim I/O info out"=w2891:T1, "error out"=w2893:errorcluster)  [unwired: 12 out]
            }
            frame "Read I/O" {
              n1031 = global read "S2C_FPGA_InterfaceGlobals.vi" "C2/P3/B6"() -> (w2897:bool)
              n1032 = To Variant(anything=w2897) -> (Variant=w2896:variant)
              n1033 = Build Array(w2896) -> (w2895:variant[])
            }
            frame "Write I/O" {
              n1034 = Index Array(array=w2905) -> (element=w2901:variant)  [unwired: 1 in]
              n1035 = Variant To Data(error in=w2904, type=TRUE, Variant=w2901) -> (data=w2900:bool, error out=w2903:errorcluster)
              n1036 = global write "S2C_FPGA_InterfaceGlobals.vi" "C2/P3/B6"(w2900) -> ()
            }
          }
        }
        frame "C2/P3/B7" {
          n1037 = case "Node or Element Type Case Structure" shown="\"Write I/O\"" w2908 {
            tunnel: w2913 -> [w2918 w2923 w2928]
            tunnel: [w2917 w2923 w2927] -> w2912
            tunnel: w2911 -> [w2916 w2922 w2930]
            tunnel: [w2915 w2922 w2930] -> w2910
            tunnel: [variant[] [] w2919 _] -> w2909
            tunnel: w2907 -> [_ _ w2929]
            frame Default {
              # "5"
              n1038 = call <vilib>:"Report Support Error.vi"("sim I/O info in"=w2916, "error in (no error)"=w2918) -> ("sim I/O info out"=w2915:T1, "error out"=w2917:errorcluster)  [unwired: 12 out]
            }
            frame "Read I/O" {
              n1039 = global read "S2C_FPGA_InterfaceGlobals.vi" "C2/P3/B7"() -> (w2921:bool)
              n1040 = To Variant(anything=w2921) -> (Variant=w2920:variant)
              n1041 = Build Array(w2920) -> (w2919:variant[])
            }
            frame "Write I/O" {
              n1042 = Index Array(array=w2929) -> (element=w2925:variant)  [unwired: 1 in]
              n1043 = Variant To Data(error in=w2928, type=TRUE, Variant=w2925) -> (data=w2924:bool, error out=w2927:errorcluster)
              n1044 = global write "S2C_FPGA_InterfaceGlobals.vi" "C2/P3/B7"(w2924) -> ()
            }
          }
        }
        frame "C2/P4/B0" {
          n1045 = case "Node or Element Type Case Structure" shown="\"Read I/O\"" w2932 {
            tunnel: w2937 -> [w2942 w2947 w2952]
            tunnel: [w2941 w2947 w2951] -> w2936
            tunnel: w2935 -> [w2940 w2946 w2954]
            tunnel: [w2939 w2946 w2954] -> w2934
            tunnel: [variant[] [] w2943 _] -> w2933
            tunnel: w2931 -> [_ _ w2953]
            frame Default {
              # "5"
              n1046 = call <vilib>:"Report Support Error.vi"("sim I/O info in"=w2940, "error in (no error)"=w2942) -> ("sim I/O info out"=w2939:T1, "error out"=w2941:errorcluster)  [unwired: 12 out]
            }
            frame "Read I/O" {
              n1047 = global read "S2C_FPGA_InterfaceGlobals.vi" "C2/P4/B0"() -> (w2945:bool)
              n1048 = To Variant(anything=w2945) -> (Variant=w2944:variant)
              n1049 = Build Array(w2944) -> (w2943:variant[])
            }
            frame "Write I/O" {
              n1050 = Index Array(array=w2953) -> (element=w2949:variant)  [unwired: 1 in]
              n1051 = Variant To Data(error in=w2952, type=TRUE, Variant=w2949) -> (data=w2948:bool, error out=w2951:errorcluster)
              n1052 = global write "S2C_FPGA_InterfaceGlobals.vi" "C2/P4/B0"(w2948) -> ()
            }
          }
        }
        frame "C2/P4/B1" {
          n1053 = case "Node or Element Type Case Structure" shown="\"Write I/O\"" w2956 {
            tunnel: w2961 -> [w2966 w2971 w2976]
            tunnel: [w2965 w2971 w2975] -> w2960
            tunnel: w2959 -> [w2964 w2970 w2978]
            tunnel: [w2963 w2970 w2978] -> w2958
            tunnel: [variant[] [] w2967 _] -> w2957
            tunnel: w2955 -> [_ _ w2977]
            frame Default {
              # "5"
              n1054 = call <vilib>:"Report Support Error.vi"("sim I/O info in"=w2964, "error in (no error)"=w2966) -> ("sim I/O info out"=w2963:T1, "error out"=w2965:errorcluster)  [unwired: 12 out]
            }
            frame "Read I/O" {
              n1055 = global read "S2C_FPGA_InterfaceGlobals.vi" "C2/P4/B1"() -> (w2969:bool)
              n1056 = To Variant(anything=w2969) -> (Variant=w2968:variant)
              n1057 = Build Array(w2968) -> (w2967:variant[])
            }
            frame "Write I/O" {
              n1058 = Index Array(array=w2977) -> (element=w2973:variant)  [unwired: 1 in]
              n1059 = Variant To Data(error in=w2976, type=TRUE, Variant=w2973) -> (data=w2972:bool, error out=w2975:errorcluster)
              n1060 = global write "S2C_FPGA_InterfaceGlobals.vi" "C2/P4/B1"(w2972) -> ()
            }
          }
        }
        frame "C2/P4/B2" {
          n1061 = case "Node or Element Type Case Structure" shown="\"Read I/O\"" w2980 {
            tunnel: w2985 -> [w2990 w2995 w3000]
            tunnel: [w2989 w2995 w2999] -> w2984
            tunnel: w2983 -> [w2988 w2994 w3002]
            tunnel: [w2987 w2994 w3002] -> w2982
            tunnel: [variant[] [] w2991 _] -> w2981
            tunnel: w2979 -> [_ _ w3001]
            frame Default {
              # "5"
              n1062 = call <vilib>:"Report Support Error.vi"("sim I/O info in"=w2988, "error in (no error)"=w2990) -> ("sim I/O info out"=w2987:T1, "error out"=w2989:errorcluster)  [unwired: 12 out]
            }
            frame "Read I/O" {
              n1063 = global read "S2C_FPGA_InterfaceGlobals.vi" "C2/P4/B2"() -> (w2993:bool)
              n1064 = To Variant(anything=w2993) -> (Variant=w2992:variant)
              n1065 = Build Array(w2992) -> (w2991:variant[])
            }
            frame "Write I/O" {
              n1066 = Index Array(array=w3001) -> (element=w2997:variant)  [unwired: 1 in]
              n1067 = Variant To Data(error in=w3000, type=TRUE, Variant=w2997) -> (data=w2996:bool, error out=w2999:errorcluster)
              n1068 = global write "S2C_FPGA_InterfaceGlobals.vi" "C2/P4/B2"(w2996) -> ()
            }
          }
        }
        frame "C2/P4/B3" {
          n1069 = case "Node or Element Type Case Structure" shown="\"Write I/O\"" w3004 {
            tunnel: w3009 -> [w3014 w3019 w3024]
            tunnel: [w3013 w3019 w3023] -> w3008
            tunnel: w3007 -> [w3012 w3018 w3026]
            tunnel: [w3011 w3018 w3026] -> w3006
            tunnel: [variant[] [] w3015 _] -> w3005
            tunnel: w3003 -> [_ _ w3025]
            frame Default {
              # "5"
              n1070 = call <vilib>:"Report Support Error.vi"("sim I/O info in"=w3012, "error in (no error)"=w3014) -> ("sim I/O info out"=w3011:T1, "error out"=w3013:errorcluster)  [unwired: 12 out]
            }
            frame "Read I/O" {
              n1071 = global read "S2C_FPGA_InterfaceGlobals.vi" "C2/P4/B3"() -> (w3017:bool)
              n1072 = To Variant(anything=w3017) -> (Variant=w3016:variant)
              n1073 = Build Array(w3016) -> (w3015:variant[])
            }
            frame "Write I/O" {
              n1074 = Index Array(array=w3025) -> (element=w3021:variant)  [unwired: 1 in]
              n1075 = Variant To Data(error in=w3024, type=TRUE, Variant=w3021) -> (data=w3020:bool, error out=w3023:errorcluster)
              n1076 = global write "S2C_FPGA_InterfaceGlobals.vi" "C2/P4/B3"(w3020) -> ()
            }
          }
        }
        frame "C2/P4/B4" {
          n1077 = case "Node or Element Type Case Structure" shown="\"Read I/O\"" w3028 {
            tunnel: w3033 -> [w3038 w3043 w3048]
            tunnel: [w3037 w3043 w3047] -> w3032
            tunnel: w3031 -> [w3036 w3042 w3050]
            tunnel: [w3035 w3042 w3050] -> w3030
            tunnel: [variant[] [] w3039 _] -> w3029
            tunnel: w3027 -> [_ _ w3049]
            frame Default {
              # "5"
              n1078 = call <vilib>:"Report Support Error.vi"("sim I/O info in"=w3036, "error in (no error)"=w3038) -> ("sim I/O info out"=w3035:T1, "error out"=w3037:errorcluster)  [unwired: 12 out]
            }
            frame "Read I/O" {
              n1079 = global read "S2C_FPGA_InterfaceGlobals.vi" "C2/P4/B4"() -> (w3041:bool)
              n1080 = To Variant(anything=w3041) -> (Variant=w3040:variant)
              n1081 = Build Array(w3040) -> (w3039:variant[])
            }
            frame "Write I/O" {
              n1082 = Index Array(array=w3049) -> (element=w3045:variant)  [unwired: 1 in]
              n1083 = Variant To Data(error in=w3048, type=TRUE, Variant=w3045) -> (data=w3044:bool, error out=w3047:errorcluster)
              n1084 = global write "S2C_FPGA_InterfaceGlobals.vi" "C2/P4/B4"(w3044) -> ()
            }
          }
        }
        frame "C2/P4/B5" {
          n1085 = case "Node or Element Type Case Structure" shown="\"Write I/O\"" w3052 {
            tunnel: w3057 -> [w3062 w3067 w3072]
            tunnel: [w3061 w3067 w3071] -> w3056
            tunnel: w3055 -> [w3060 w3066 w3074]
            tunnel: [w3059 w3066 w3074] -> w3054
            tunnel: [variant[] [] w3063 _] -> w3053
            tunnel: w3051 -> [_ _ w3073]
            frame Default {
              # "5"
              n1086 = call <vilib>:"Report Support Error.vi"("sim I/O info in"=w3060, "error in (no error)"=w3062) -> ("sim I/O info out"=w3059:T1, "error out"=w3061:errorcluster)  [unwired: 12 out]
            }
            frame "Read I/O" {
              n1087 = global read "S2C_FPGA_InterfaceGlobals.vi" "C2/P4/B5"() -> (w3065:bool)
              n1088 = To Variant(anything=w3065) -> (Variant=w3064:variant)
              n1089 = Build Array(w3064) -> (w3063:variant[])
            }
            frame "Write I/O" {
              n1090 = Index Array(array=w3073) -> (element=w3069:variant)  [unwired: 1 in]
              n1091 = Variant To Data(error in=w3072, type=TRUE, Variant=w3069) -> (data=w3068:bool, error out=w3071:errorcluster)
              n1092 = global write "S2C_FPGA_InterfaceGlobals.vi" "C2/P4/B5"(w3068) -> ()
            }
          }
        }
        frame "C2/P4/B6" {
          n1093 = case "Node or Element Type Case Structure" shown="\"Read I/O\"" w3076 {
            tunnel: w3081 -> [w3086 w3091 w3096]
            tunnel: [w3085 w3091 w3095] -> w3080
            tunnel: w3079 -> [w3084 w3090 w3098]
            tunnel: [w3083 w3090 w3098] -> w3078
            tunnel: [variant[] [] w3087 _] -> w3077
            tunnel: w3075 -> [_ _ w3097]
            frame Default {
              # "5"
              n1094 = call <vilib>:"Report Support Error.vi"("sim I/O info in"=w3084, "error in (no error)"=w3086) -> ("sim I/O info out"=w3083:T1, "error out"=w3085:errorcluster)  [unwired: 12 out]
            }
            frame "Read I/O" {
              n1095 = global read "S2C_FPGA_InterfaceGlobals.vi" "C2/P4/B6"() -> (w3089:bool)
              n1096 = To Variant(anything=w3089) -> (Variant=w3088:variant)
              n1097 = Build Array(w3088) -> (w3087:variant[])
            }
            frame "Write I/O" {
              n1098 = Index Array(array=w3097) -> (element=w3093:variant)  [unwired: 1 in]
              n1099 = Variant To Data(error in=w3096, type=TRUE, Variant=w3093) -> (data=w3092:bool, error out=w3095:errorcluster)
              n1100 = global write "S2C_FPGA_InterfaceGlobals.vi" "C2/P4/B6"(w3092) -> ()
            }
          }
        }
        frame "C2/P4/B7" {
          n1101 = case "Node or Element Type Case Structure" shown="\"Write I/O\"" w3100 {
            tunnel: w3105 -> [w3110 w3115 w3120]
            tunnel: [w3109 w3115 w3119] -> w3104
            tunnel: w3103 -> [w3108 w3114 w3122]
            tunnel: [w3107 w3114 w3122] -> w3102
            tunnel: [variant[] [] w3111 _] -> w3101
            tunnel: w3099 -> [_ _ w3121]
            frame Default {
              # "5"
              n1102 = call <vilib>:"Report Support Error.vi"("sim I/O info in"=w3108, "error in (no error)"=w3110) -> ("sim I/O info out"=w3107:T1, "error out"=w3109:errorcluster)  [unwired: 12 out]
            }
            frame "Read I/O" {
              n1103 = global read "S2C_FPGA_InterfaceGlobals.vi" "C2/P4/B7"() -> (w3113:bool)
              n1104 = To Variant(anything=w3113) -> (Variant=w3112:variant)
              n1105 = Build Array(w3112) -> (w3111:variant[])
            }
            frame "Write I/O" {
              n1106 = Index Array(array=w3121) -> (element=w3117:variant)  [unwired: 1 in]
              n1107 = Variant To Data(error in=w3120, type=TRUE, Variant=w3117) -> (data=w3116:bool, error out=w3119:errorcluster)
              n1108 = global write "S2C_FPGA_InterfaceGlobals.vi" "C2/P4/B7"(w3116) -> ()
            }
          }
        }
      }
    }
    frame "Shutting Down" {
    }
    frame Default {
    }
  }
  "data to node output terminals" <- w9
  n1109 = call <vilib>:"Error Handler.vi"("sim I/O info in"=w6, "error in"=w4) -> ("sim I/O info out"=→"sim I/O info out":T1)  [unwired: 13 out]
  "output to node terminal error out" <- "input from node terminal error in"
